vi "Main_Marvin Remake.vi"() -> ()   [LabVIEW 2017]
uses:
  PCAN_Driver/ControlCAN.llb/DevType.ctl
  PCAN_Driver/ControlCAN.llb/CAN Channel.ctl
  PCAN_Driver/ControlCAN.llb/VCI_INIT_CONFIG.ctl
  PCAN_Driver/ControlCAN.llb/InitFlag.ctl
  PCAN_Driver/ControlCAN.llb/Fliter.ctl
  PCAN_Driver/ControlCAN.llb/Mode.ctl
  <vilib>/Utility/miscctls.llb/LVRowAndColumnTypeDef.ctl
  <vilib>/Utility/config.llb/Read Key (String).vi
  <vilib>/Utility/config.llb/Write Key (String).vi
  <vilib>/Utility/cursorutil.llb/Set Cursor (Icon Pict).vi
  PCAN_Driver/ControlCAN.lvlib
  <vilib>/Utility/config.llb/NI_LVConfig.lvlib
panel:
  out "ClosePanel":bool=TRUE
  out "UUT SN Report":string
  out "Automation":bool
  out "Test Failed":bool
  out "AuxiOFFResult":bool
  out "AuxiONResult":bool
  out "SensCalResult":bool
  out "VisualInspectionResult":bool
  out "BurnResult":bool
  out "BurnSpeed":bool
  out "BurnTemp":bool
  out "BurnDC":bool
  out "TempControlResult":bool
  out "MotorTempResult":bool
  out "StopTimeResult":bool
  out "SpeedResult":bool=TRUE
  out "VenableDirectionResult":bool
  out "VenableResult":bool
  out "ComTestResult":bool=TRUE
  out "UUT SoftwareVer":string
  out "Next SN":i32
  in  "SetSN":bool
  out "Current SN":i32
  out "Cal":dbl
  out "AO[1]Meas":dbl
  out "FullSpeed2 Speed":dbl
  out "FullSpeed2 Current":dbl
  out "FullSpeed1 Current":dbl
  out "FullSpeed1 Speed":dbl
  out "MaxBurnInTempVal":dbl
  in  "Stop Burn-in":bool
  out "VISA Tester":refnum<visa-resource-name>
  out "UUT":u8
  out "CAN Status":bool
  in  "Channel 2":T1 caption="Channel" items=["Channel 1", "Channel 2"]
  out "Config_CANAT":T7 {"DevType" items=["USB-CAN"=3, "USB-CAN2"=4]; "CanIndex" items=["通道1", "通道2"]; "VCI_INIT_CONFIG"."Fliter" items=["接收所有类型"=3, "只接收标准帧"=4, "只接收扩展帧"=7]; "VCI_INIT_CONFIG"."Mode" items=["正常工作", "自测模式（环回）", "仅侦听模式"]; "VCI_INIT_CONFIG"."InitFlag" items=["使用Flash参数", "使用界面设置参数"]}
  out "Array":u64[][](array[numeric]) format="%016x"
  out "Motor Phase Current RMS":dbl
  out "Ambient Temperature":dbl
  out "Speed error":bool
  out "Commutation err":bool
  out "Under voltage/Over voltage":bool
  out "Derated drive temp":bool
  out "Motor Over temperature":bool
  out "Motor Sensor temp Fauilre":bool
  out "Drive Over temperature":bool
  out "Drive Sensor temp Failure":bool
  out "Ambient Over temp":bool
  out "Ambient Sensor temp":bool
  out "DC Voltage":dbl
  out "DC Current":dbl
  out "Power transistor Heat sink Temp.":dbl
  out "Motor Stator Temp.":dbl
  out "Motor Speed RPM":dbl
  out "ECS State":u16
  out "UUT":string="EBAY"
  in  "Logger Path":path
  in  "Report":bool
  in  "Start":bool
  in  "ATR":string[][](table)=[["Test Communication", "-", "-", "-", "-", ""], ["Set S/N", "-", "-", "-", "-", ""], ["Set Board Number", "-", "-", "-", "-", ""], [" ", "", "", "", "", ""], ["Test Communication", "-", "-", "-", "-", ""], ["Get S/N", "-", "-", "-", "", ""], ["Get Board Number", "-", "-", "-", "", ""], ["Get FW", "-", "-", "-", "", ""], ["Enable Motor", "", "", "", "", ""], ["Small position command", "", "", "", "", ""], ["Measure delta", "", "", "", "", ""], ["Velocity command", "", "", "", "", ""]]
  in  "Settings":bool
  in  "Refresh Button":bool
  out "Status":bool
  in  "VISA Marvin":refnum<visa-resource-name>="COM6"
  in  "Serial Com":bool
  in  "Help Button":bool
  out "Pannel User Message":string
  in  "Stop Button":bool
  # "Marvin"
  # "REDLER TECHNOLOGIES LTD"
  # "ver 1.2l"
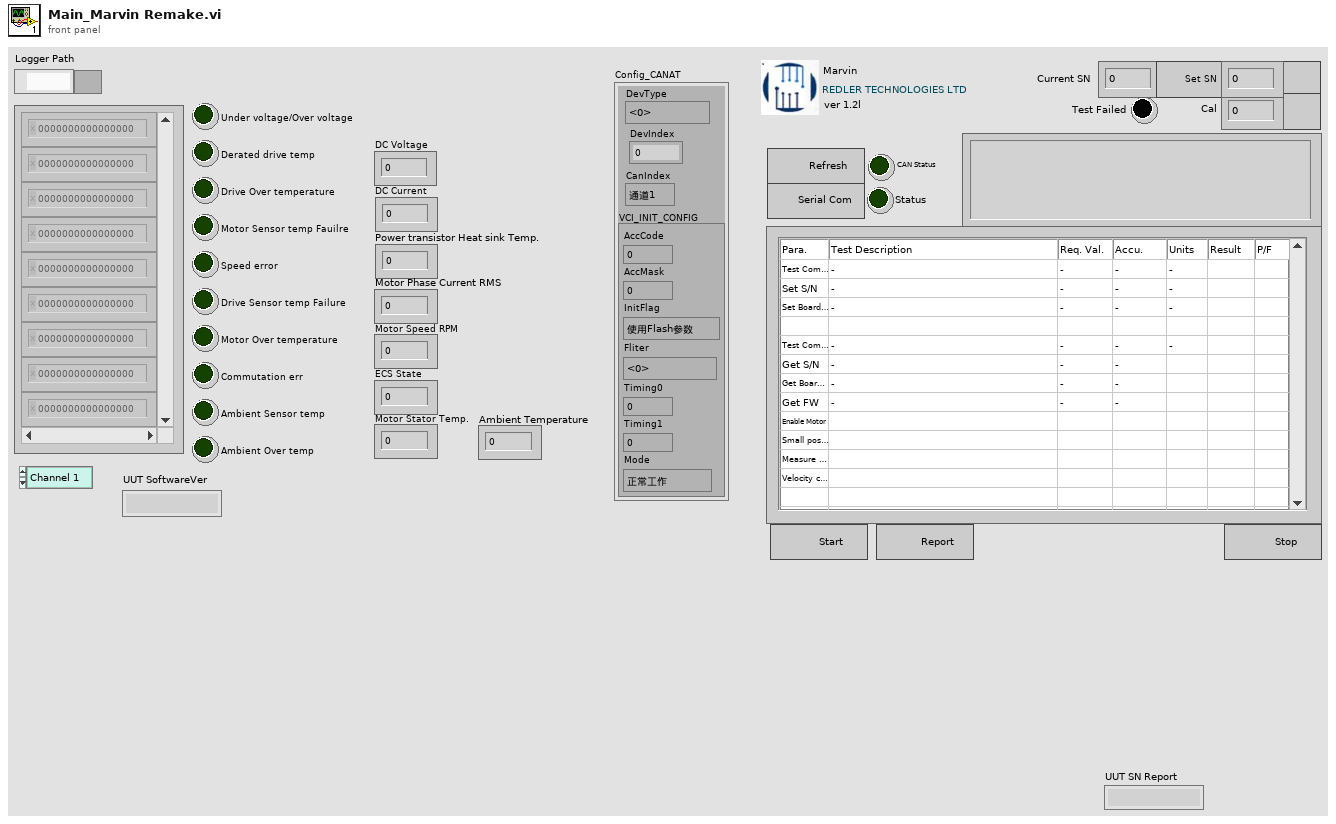
[diagram p1: front panel]
types:
  T1 = typedef "ControlCAN.lvlib/CAN Channel.ctl" = u32
  T2 = typedef "ControlCAN.lvlib/DevType.ctl" = u32
  T3 = typedef "ControlCAN.lvlib/VCI_INIT_CONFIG.ctl" = cluster{"AccCode":u32, "AccMask":u32, "InitFlag":T4, "Fliter":T5, "Timing0":u8, "Timing1":u8, "Mode":T6}
  T4 = typedef "ControlCAN.lvlib/InitFlag.ctl" = u32
  T5 = typedef "ControlCAN.lvlib/Fliter.ctl" = u8
  T6 = typedef "ControlCAN.lvlib/Mode.ctl" = u8
  T7 = cluster{"DevType":T2, "DevIndex":u32, "CanIndex":T1, "VCI_INIT_CONFIG":T3}
  T8 = cluster{"VISA":refnum<visa-resource-name>, "Array Test":enum16{"Auxiliary", "Temp Sens Cal", "Com Test", "Enable Test", "Speed Command", "Stop Time", "Temp Control", "Burn in", "Visual Inspec", "Empty"}[]}
  T9 = cluster{"ID":u32, "MSGTYPE":u8, "LEN":u8, "aDATA":u8[]}[]
  T10 = enum16{"Erase ATR Table", "Stop", "MainProgram", "Initialize"}
  T11 = enum16{"K15", "K16", "K17", "Venable", "Firmeware", "Fan", "Power", "120C", "110C", "100C", "90C", "80C", "70C", "60C", "50C", "40C", "30C", "25C", "20C", "10C", "0C"}
  T12 = enum16{"Stop", "Result", "FullSpeed2", "MD[1]=1", "FullSpeed1", "MD[1]=0"}
  T13 = enum8{"Term1", "Term2", "Current", "Fan", "TempCPU"}
  T14 = enum16{"Stop", "AO[1]=Meas.", "TA[5]", "AO[1]=0", "Start"}
  T15 = enum16{"Stop", "BurnIn", "Ambient Temp", "MotorSpeed", "DC Current Measure", "Start"}
  T16 = enum16{"Auxiliary", "Temp Sens Cal", "Com Test", "Enable Test", "Speed Command", "Stop Time", "Temp Control", "Burn in", "Visual Inspec", "Empty"}[]
  T17 = enum16{"K15", "K16", "K17", "Venable", "Firmeware", "Fan", "Power", "120C", "110C", "100C", "90C", "80C", "70C", "60C", "50C", "40C", "30C", "25C", "20C", "10C", "0C"}[]
  T18 = enum32{"6000", "11500", "15100", "11500-2", "6000-2"}[]
  T19 = enum8{"Enabled", "Disabled", "Disabled and Grayed Out"}
  T20 = typedef "LVRowAndColumnTypeDef.ctl" = cluster{"Row":i32, "Column":i32}
  T21 = enum32{"Invalid", "Standard", "Closed", "Hidden", "Minimized", "Maximized"}
  T22 = cluster{"ID":u32, "MSGTYPE":u8, "LEN":u8, "aDATA":u8[]}
  T23 = enum16{"Auxiliary", "Temp Sens Cal", "Com Test", "Enable Test", "Speed Command", "Stop Time", "Temp Control", "Burn in", "Visual Inspec", "Empty"}
  T24 = enum16{"open", "replace", "create", "open or create", "replace or create", "replace or create with confirmation"}
  T25 = typedef "NI_LVConfig.lvlib/Config Data RefNum.ctl" = refnum<k1>
  T26 = typedef "ControlCAN.lvlib/VCI_CAN_OBJ.ctl" = cluster{"ID":u32, "TimeStamp":u32, "TimeFlag":u8, "SendType":u8, "RemoteFlag":u8, "ExternFlag":u8, "DataLen":u8, "Data":u8[], "Reserved":u8[]}
  T27 = cluster{"Type":enum16{"接收", "发送"}, "Channel":T1, "Time":timestamp, "VCI_CAN_OBJ":T26}[]
  T28 = cluster{"Type":enum16{"接收", "发送"}, "Channel":T1, "Time":timestamp, "VCI_CAN_OBJ":T26}
  T29 = typedef "LVPoint32TypeDef.ctl" = cluster{"Horizontal":i32, "Vertical":i32}
  T30 = enum8{"Term1", "Term2", "Current", "Fan", "TempCPU"}[]
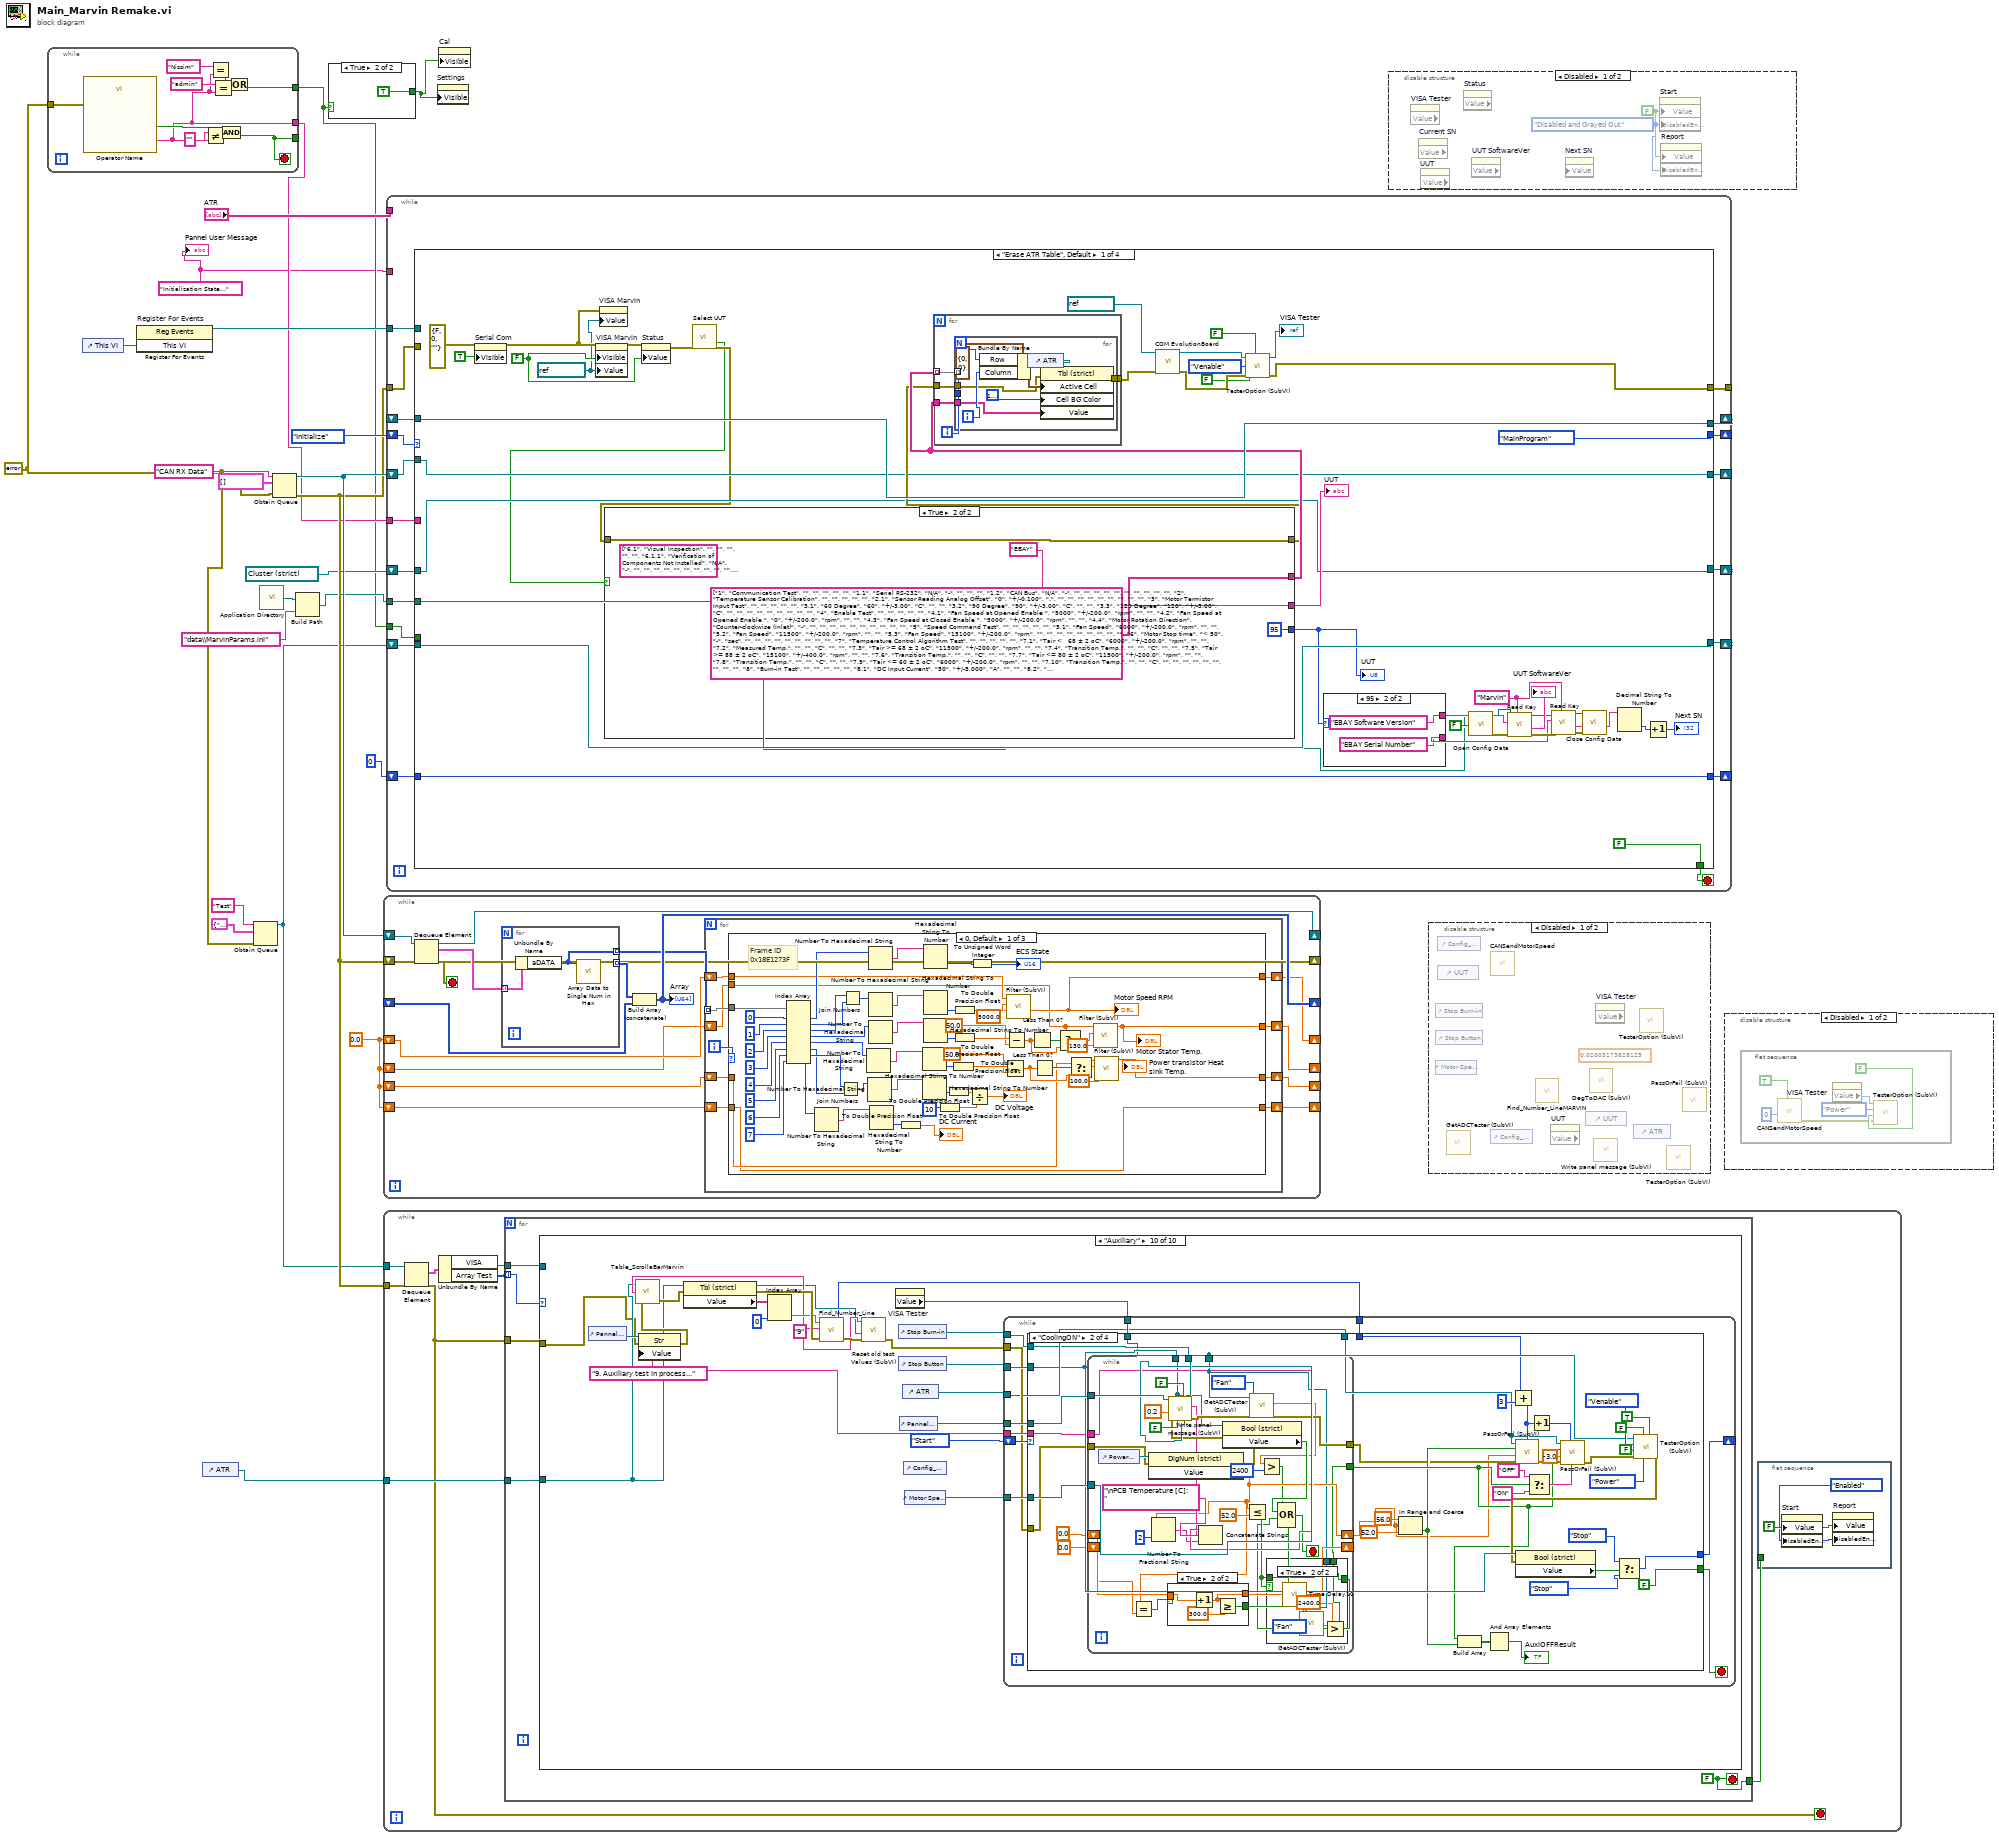
[diagram p0: block diagram]
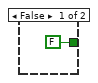
[diagram p2: hidden frame]
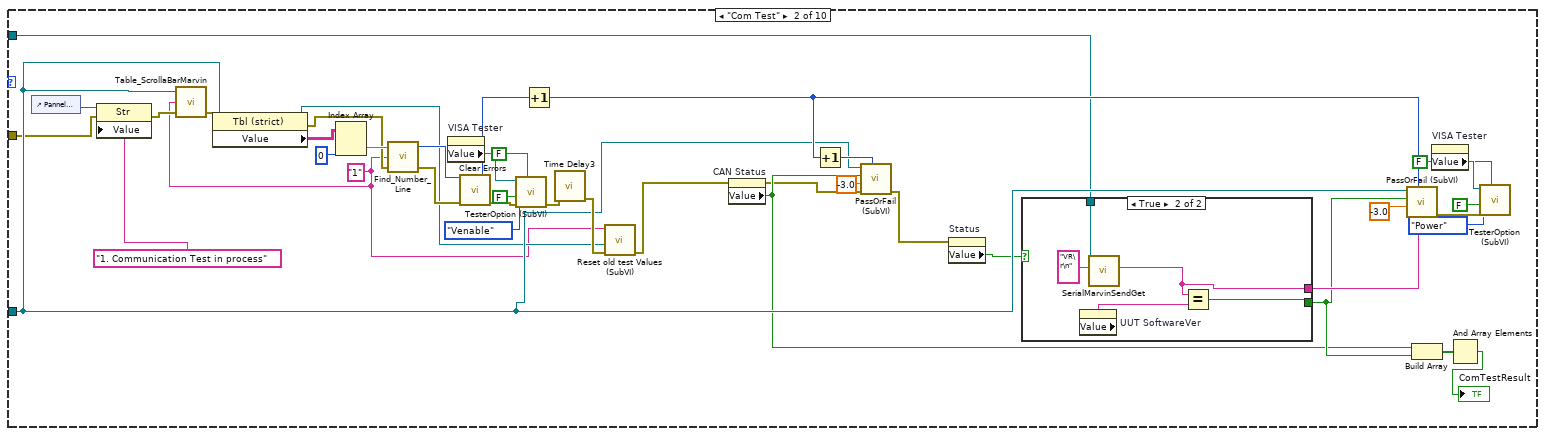
[diagram p7: hidden frame]
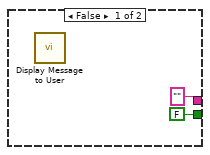
[diagram p8: hidden frame]
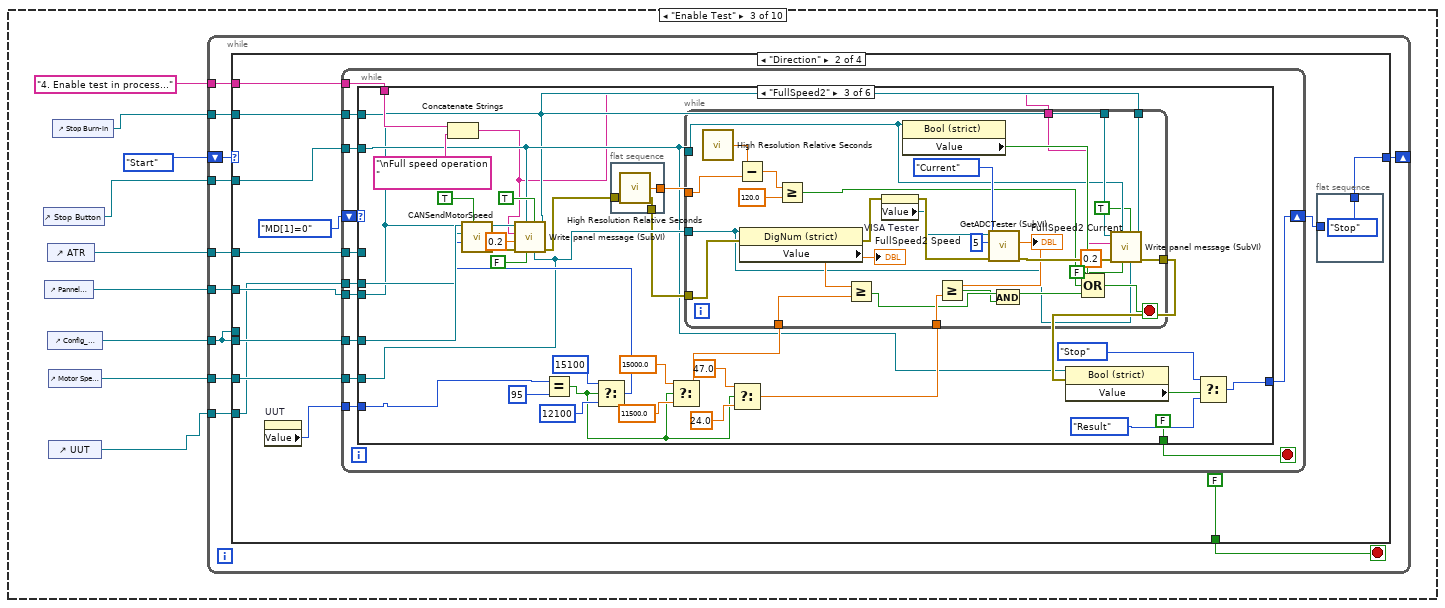
[diagram p9: hidden frame]
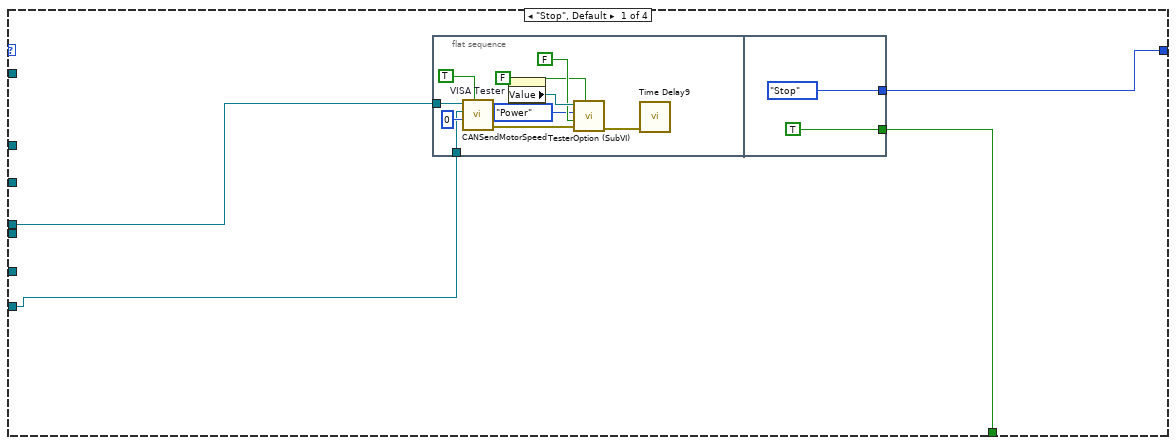
[diagram p10: hidden frame]
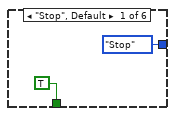
[diagram p11: hidden frame]
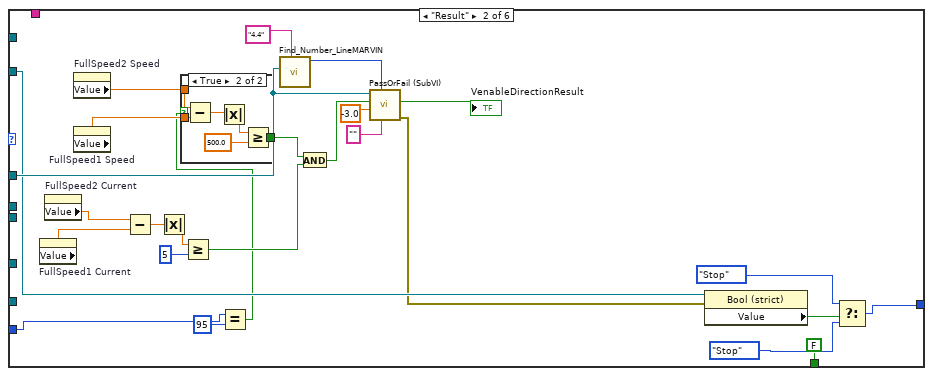
[diagram p12: hidden frame]
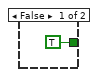
[diagram p13: hidden frame]
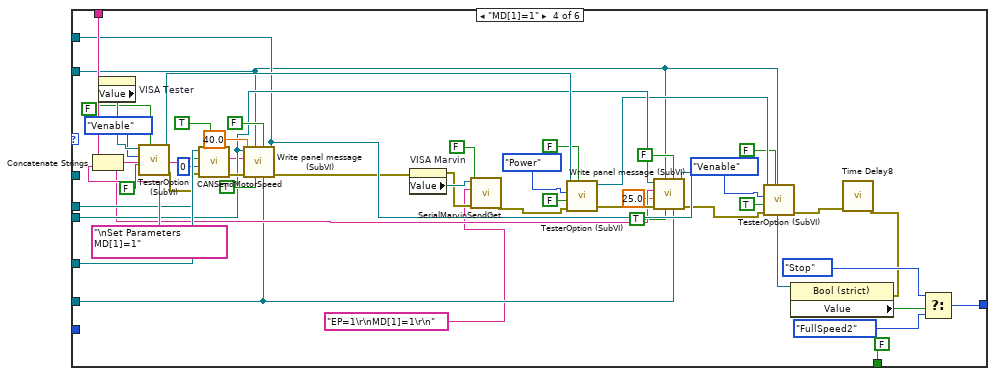
[diagram p14: hidden frame]
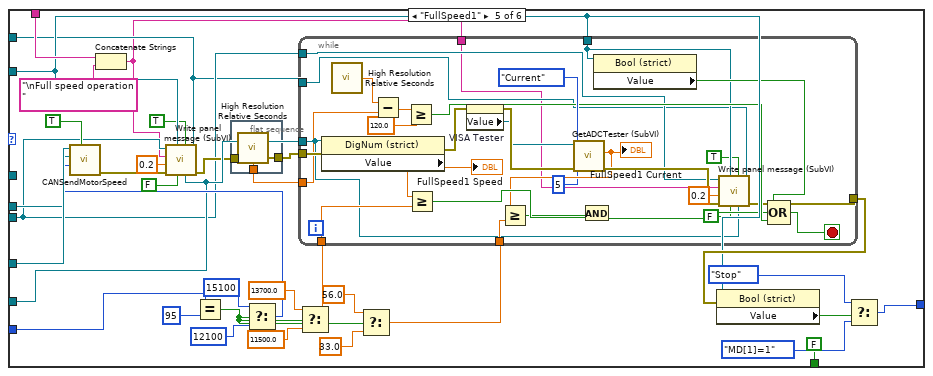
[diagram p15: hidden frame]
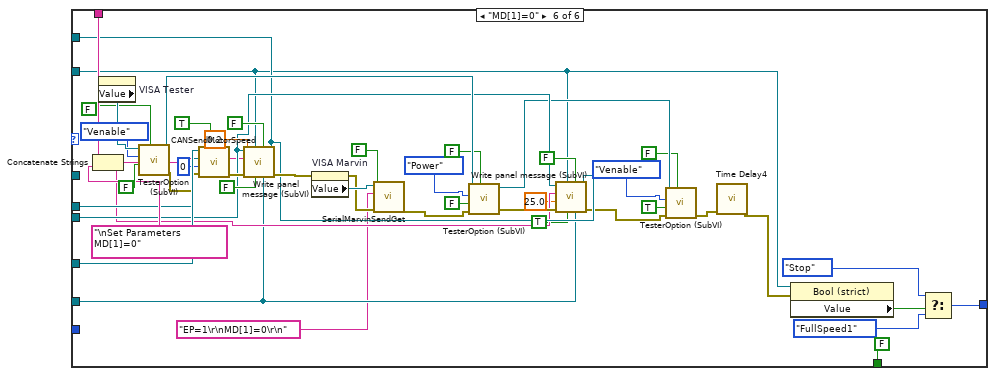
[diagram p16: hidden frame]
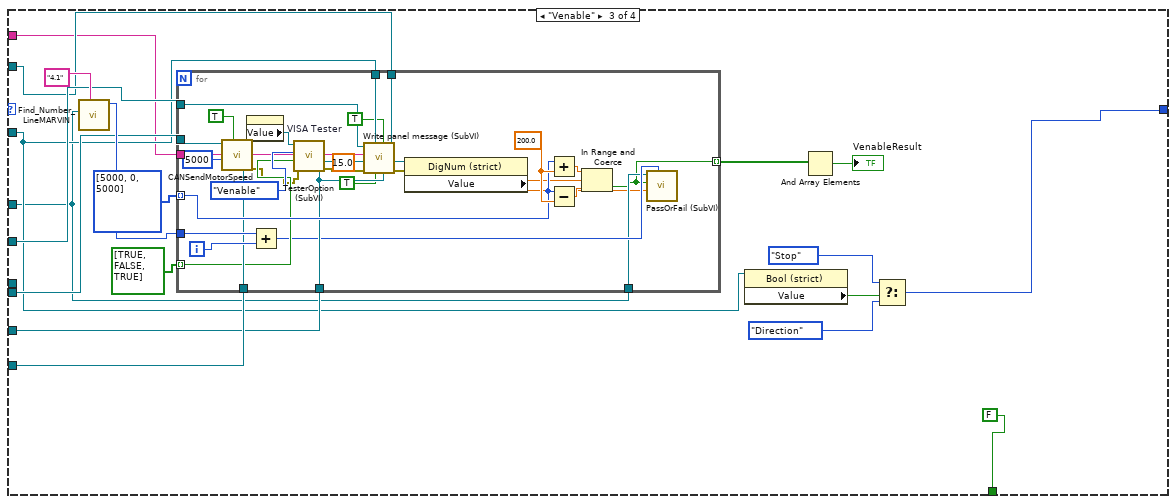
[diagram p17: hidden frame]
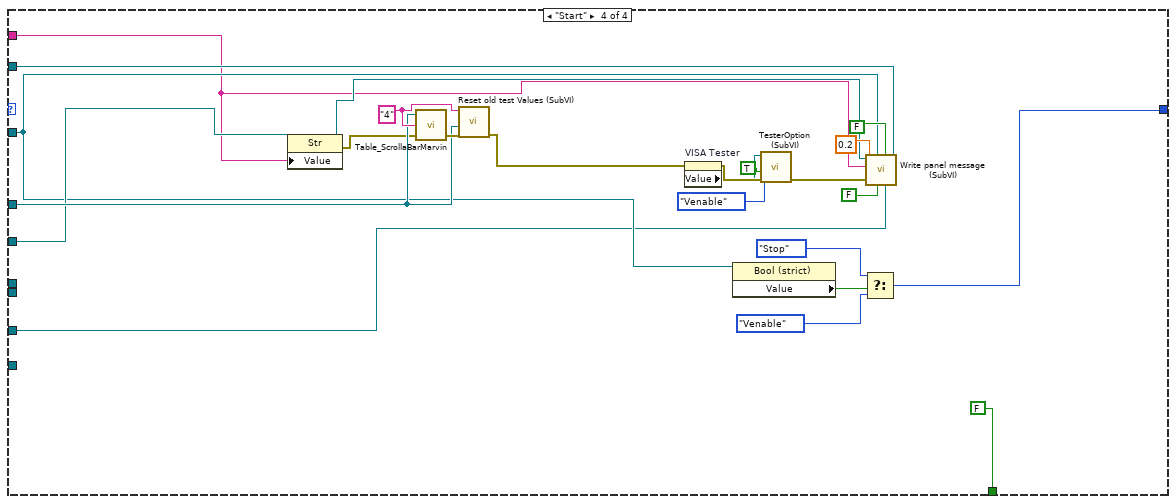
[diagram p18: hidden frame]
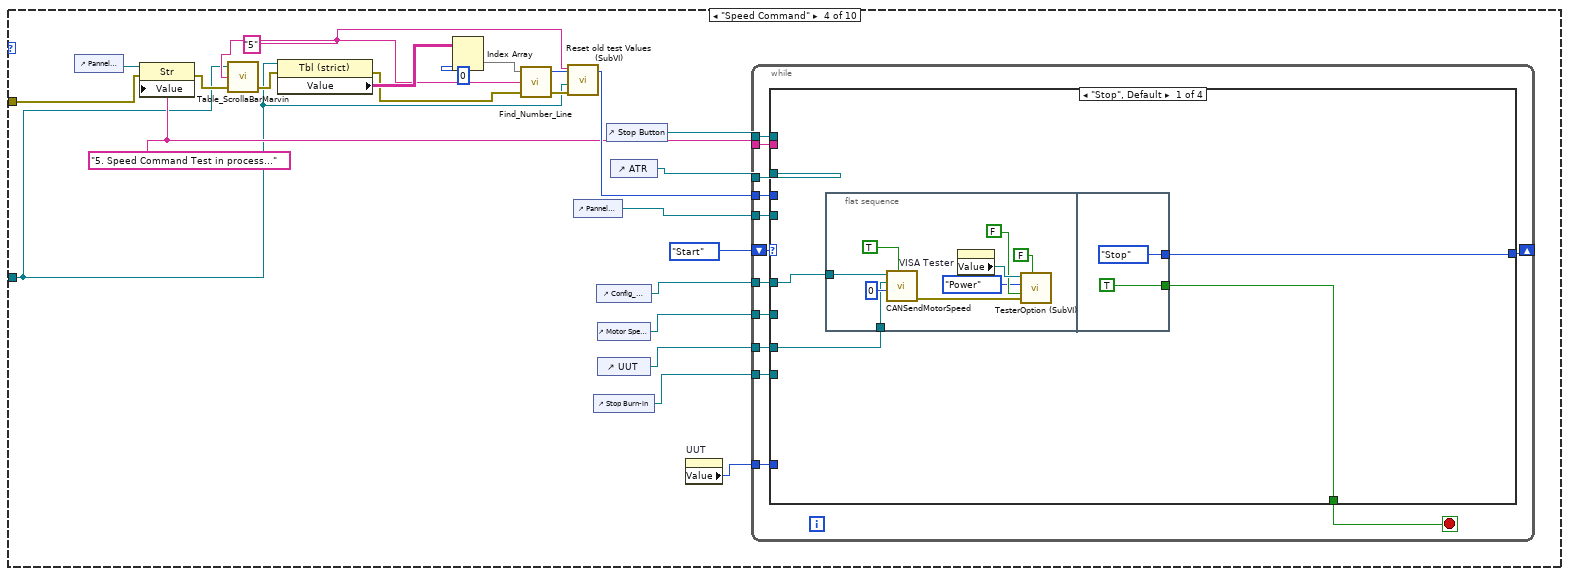
[diagram p19: hidden frame]
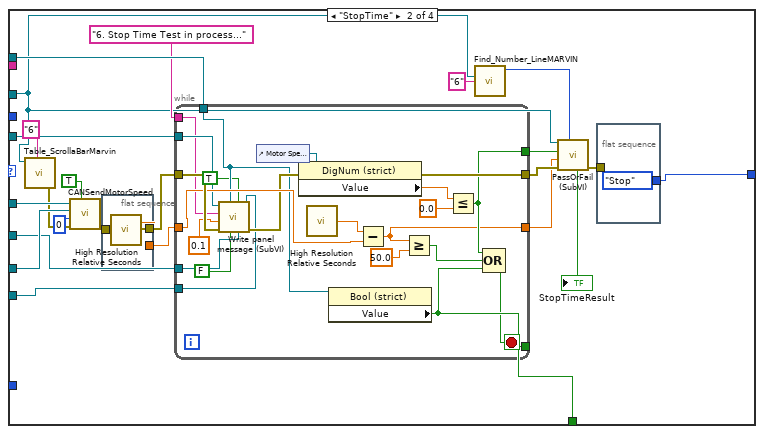
[diagram p20: hidden frame]
diagram:
  w2 = "Initialization State..."
  w13 = 0.0
  w12 = errorcluster {"status"=FALSE, "code"=0, "source"=""} ("error in (no error)")
  n1 = while {
    tunnel: [w31] -> _
    tunnel: [w27] -> w7
    tunnel: [w28] -> w3
    tunnel: w12 -> [w24]
    stop <- w31 stop-if-true
    n2 = call "Operator Name"("error in (no error)"=w24) -> ("Operator Name"=w27:string, "OK"=w32:bool)  [unwired: 16 in, 1 out]
    n3 = Not Equal?(x=w27, y="") -> (x != y?=w33:bool)
    n4 = Equal?(x="Nissim", y=w27) -> (x = y?=w25:bool)
    n5 = Equal?(x="admin", y=w27) -> (x = y?=w29:bool)
    n6 = And(x=w32, y=w33) -> (x .and. y?=w31:bool)
    n7 = Or(x=w25, y=w29) -> (x .or. y?=w28:bool)
  }
  n8 = control-ref of="This VI"() -> (w9:refnum<vi>)
  n9 = register-events "Register For Events"(w9) -> (reference out=w8:refnum<event-registration>)  [unwired: 2 in, 1 out]
  n10 = control-ref of="ATR"() -> (w1:refnum<vi>)
  n11 = Obtain Queue(name (unnamed)="Test", element data type=T8 {"VISA"="COM1", "Array Test"=[]}, error in (no error)=w12) -> (queue out=w17:refnum<queue>)  [unwired: 2 in, 2 out]
  n12 = call <vilib>:"Application Directory.vi"() -> ("Application Directory"=w11:path)
  n13 = Obtain Queue(name (unnamed)="CAN RX Data", element data type=T9 [], error in (no error)=w12) -> (queue out=w20:refnum<queue>, error out=w18:errorcluster)  [unwired: 2 in, 1 out]
  n14 = Build Path(base path=w11, name or relative path="data\\MarvinParams.ini") -> (appended path=w5:path)
  n15 = case shown="True" w3 {
    tunnel: [FALSE TRUE] -> w4
    frame False {
    }
    frame True {
    }
  }
  n16 = while {
    shift-right: [w51] -> _
    shift-left: w20 -> [w53]
    shift-right: [w49] -> _
    shift-left: _ -> [w50]
    shift-right: [w45] -> _
    shift-left: w18 -> [w45]
    shift-right: [w43] -> _
    shift-left: w13 -> [w44]
    shift-right: [w42] -> _
    shift-left: w13 -> [w41]
    shift-right: [w40] -> _
    shift-left: w13 -> [w39]
    shift-right: [w38] -> _
    shift-left: w13 -> [w37]
    stop <- w52 stop-if-true
    n17 = Dequeue Element(queue=w53, error in (no error)=w45) -> (queue out=w51:refnum<queue>, element=w46:T9, error out=w52:errorcluster)  [unwired: 1 in, 1 out]
    n18 = for {
      tunnel: [w182] -> w48 mode=indexing
      tunnel: w46 -> [w181] mode=indexing
      tunnel: [w180] -> w47 mode=indexing
      n19 = Unbundle By Name(w181) -> ("aDATA"=w180:u8[])
      n20 = call "Array Data to Single Num in Hex.vi"("aDATA"=w180) -> ("Numeric"=w182:u64)  [unwired: 10 in]
    }
    n21 = Build Array (concatenate)(w48, w50) -> (w49:u64[][])
    "Array" <- w49
    n22 = for {
      tunnel: w47 -> [w63] mode=indexing
      shift-right: [w60] -> w43
      shift-left: w44 -> [w61]
      shift-right: [w59] -> w42
      shift-left: w41 -> [w58]
      shift-right: [w57] -> w40
      shift-left: w39 -> [w56]
      shift-right: [w55] -> w38
      shift-left: w37 -> [w54]
      i -> [w62]
      n23 = case shown="0, Default" w62 {
        tunnel: w63 -> [w103 w136 w175]
        tunnel: w61 -> [w77 w125 w164]
        tunnel: [w75 w125 w164] -> w60
        tunnel: [w72 w124 w163] -> w59
        tunnel: w58 -> [w71 w124 w163]
        tunnel: [w66 w123 w162] -> w57
        tunnel: w56 -> [w65 w123 w162]
        tunnel: [w64 w122 w157] -> w55
        tunnel: w54 -> [w64 w122 w156]
        frame 0, Default {
          # "Frame ID\n0x18E1273F"
          n24 = Index Array(array=w103, index #1=0 ("index"), index #2=1 ("index"), index #3=2 ("index"), index #4=3 ("index"), index #5=4 ("index"), index #6=5 ("index"), index #7=6 ("index"), index #8=7 ("index")) -> (element #1=w87:u8, element #2=w89:u8, element #3=w90:u8, element #4=w94:u8, element #5=w97:u8, element #6=w101:u8, element #7=w102:u8, element #8=w100:u8)
          n25 = Number To Hexadecimal String(2:w100) -> (0:w114:string)  [unwired: 1 in]
          n26 = Join Numbers(hi=w102, lo=w101) -> ((hi.lo)=w121:u16)
          n27 = Join Numbers(hi=w90, lo=w89) -> ((hi.lo)=w91:u16)
          n28 = Number To Hexadecimal String(2:w97) -> (0:w98:string)  [unwired: 1 in]
          n29 = Number To Hexadecimal String(2:w121) -> (0:w120:string)  [unwired: 1 in]
          n30 = Number To Hexadecimal String(2:w87) -> (0:w88:string)  [unwired: 1 in]
          n31 = Number To Hexadecimal String(2:w91) -> (0:w92:string)  [unwired: 1 in]
          n32 = Number To Hexadecimal String(2:w94) -> (0:w95:string)  [unwired: 1 in]
          n33 = Hexadecimal String To Number(string=w114) -> (number=w113:u32)  [unwired: 2 in, 1 out]
          n34 = To Double Precision Float(number=w113) -> (double precision float=→"DC Current":dbl)
          n35 = Hexadecimal String To Number(string=w98) -> (number=w99:u32)  [unwired: 2 in, 1 out]
          n36 = Hexadecimal String To Number(string=w120) -> (number=w119:u32)  [unwired: 2 in, 1 out]
          n37 = Hexadecimal String To Number(string=w88) -> (number=w85:u32)  [unwired: 2 in, 1 out]
          n38 = Hexadecimal String To Number(string=w92) -> (number=w93:u32)  [unwired: 2 in, 1 out]
          n39 = Hexadecimal String To Number(string=w95) -> (number=w96:u32)  [unwired: 2 in, 1 out]
          n40 = To Double Precision Float(number=u32 10 ("y")) -> (double precision float=w117:dbl)
          n41 = To Double Precision Float(number=w119) -> (double precision float=w116:dbl)
          n42 = To Double Precision Float(number=w99) -> (double precision float=w82:dbl)
          n43 = To Double Precision Float(number=w93) -> (double precision float=w78:dbl)
          n44 = To Double Precision Float(number=w96) -> (double precision float=w84:dbl)
          n45 = Divide(x=w116, y=w117) -> (x/y=→"DC Voltage":dbl)
          n46 = To Unsigned Word Integer(number=w85) -> (unsigned 16bit integer=→"ECS State":u16)
          n47 = Subtract(x=w82, y=50.0 ("x")) -> (x-y=w70:dbl)
          n48 = Subtract(x=w84, y=50.0 ("x")) -> (x-y=w73:dbl)
          n49 = call "Filter (SubVI).vi"("Delta"=5000.0, "NewVal"=w78, "OldVal"=w77) -> ("Val"=w75:dbl)  [unwired: 8 in]
          "Motor Speed RPM" <- w75
          n50 = Less Than 0?(x=w73) -> (x < 0?=w80:bool)
          n51 = Less Than 0?(x=w70) -> (x < 0?=w79:bool)
          n52 = Select(t=w71, s=w80, f=w73) -> (s? t:f=w74:dbl)
          n53 = Select(t=w65, s=w79, f=w70) -> (s? t:f=w69:dbl)
          n54 = call "Filter (SubVI).vi"("Delta"=130.0, "NewVal"=w74, "OldVal"=w71) -> ("Val"=w72:dbl)  [unwired: 8 in]
          "Motor Stator Temp." <- w72
          n55 = call "Filter (SubVI).vi"("Delta"=100.0, "NewVal"=w69, "OldVal"=w65) -> ("Val"=w66:dbl)  [unwired: 8 in]
          "Power transistor Heat sink Temp." <- w66
        }
        frame 1 {
          # "Framde ID\n0x18E3273F"
          n56 = control-ref of="UUT"() -> (w126:refnum<vi>)
          n57 = property on="Property Node" class="DigNum (strict)"(reference=w126) -> ("Value"=w127:u8)  [unwired: 1 in, 2 out]
          n58 = Index Array(array=w136, index #1=0 ("index"), index #2=1 ("index")) -> (element #1=w134:u8, element #2=w129:u8)
          n59 = Number To Boolean Array(number=w134) -> (Boolean array=w133:bool[])
          n60 = Number To Boolean Array(number=w129) -> (Boolean array=w131:bool[])
          n61 = Boolean To (0,1)(Boolean=w131) -> (0, 1=w128:i16[])
          n62 = Boolean To (0,1)(Boolean=w133) -> (0, 1=w132:i16[])
          n63 = case shown="95" w127 {
            tunnel: w128 -> [_ w137]
            frame 0, Default {
            }
            frame 95 {
              n64 = for {
                tunnel: w137 -> [w142] mode=indexing
                i -> [w138]
                stop <- w140 stop-if-true
                n65 = Not Equal To 0?(x=w142) -> (x != 0?=w141:bool)
                n66 = case shown="0, Default" w138 {
                  tunnel: w141 -> [w143 w144]
                  frame 0, Default {
                    "Ambient Sensor temp" <- w143
                  }
                  frame 1 {
                    "Ambient Over temp" <- w144
                  }
                }
                n67 = Equal?(x=w138, y=1.0) -> (x = y?=w140:bool)
              }
            }
          }
          n68 = for {
            tunnel: w132 -> [w146] mode=indexing
            i -> [w147]
            n69 = Not Equal To 0?(x=w146) -> (x != 0?=w145:bool)
            n70 = case shown="1" w147 {
              tunnel: w145 -> [w148 w149 w150 w151 w152 w153 w154 w155]
              frame 0, Default {
                "Drive Sensor temp Failure" <- w148
              }
              frame 1 {
                "Drive Over temperature" <- w149
              }
              frame 2 {
                "Motor Sensor temp Fauilre" <- w150
              }
              frame 3 {
                "Motor Over temperature" <- w151
              }
              frame 4 {
                "Derated drive temp" <- w152
              }
              frame 5 {
                "Under voltage/Over voltage" <- w153
              }
              frame 6 {
                "Commutation err" <- w154
              }
              frame 7 {
                "Speed error" <- w155
              }
            }
          }
        }
        frame 2 {
          # "Frame ID\n0x18E2273F"
          n71 = Index Array(array=w175, index #1=0 ("index"), index #2=1 ("index")) -> (element #1=w172:u8, element #2=w169:u8)
          n72 = disable-structure shown="Enabled" {
            disable-tunnel: [w178 w179] -> w173
            disable-tunnel: w172 -> [w177 w179]
            frame Disabled {
              n73 = Number To Hexadecimal String(2:w177) -> (0:w176:string)  [unwired: 1 in]
              n74 = Hexadecimal String To Number(string=w176) -> (number=w178:u32)  [unwired: 2 in, 1 out]
            }
            frame Enabled {
            }
          }
          n75 = Number To Hexadecimal String(2:w169) -> (0:w167:string)  [unwired: 1 in]
          n76 = Hexadecimal String To Number(string=w167) -> (number=w168:u32)  [unwired: 2 in, 1 out]
          n77 = To Double Precision Float(number=w168) -> (double precision float=w166:dbl)
          n78 = To Double Precision Float(number=w173) -> (double precision float=→"Motor Phase Current RMS":dbl)
          n79 = Subtract(x=w166, y=50.0) -> (x-y=w160:dbl)
          n80 = Less Than 0?(x=w160) -> (x < 0?=w161:bool)
          n81 = Select(t=w156, s=w161, f=w160) -> (s? t:f=w159:dbl)
          n82 = call "Filter (SubVI).vi"("Delta"=65.0, "NewVal"=w159, "OldVal"=w156) -> ("Val"=w157:dbl)  [unwired: 8 in]
          "Ambient Temperature" <- w157
        }
      }
    }
  }
  n83 = while {
    tunnel: w1 -> [w190]
    tunnel: w18 -> [w188]
    tunnel: w17 -> [w189]
    stop <- w184 stop-if-true
    n84 = Dequeue Element(queue=w189, error in (no error)=w188) -> (element=w187:T8, error out=w184:errorcluster)  [unwired: 1 in, 2 out]
    n85 = Unbundle By Name(w187) -> ("VISA"=w186:refnum<visa-resource-name>, "Array Test"=w185:T16)
    n86 = for {
      tunnel: w185 -> [w194] mode=indexing
      tunnel: w186 -> [w197]
      tunnel: w190 -> [w196]
      tunnel: w184 -> [w195]
      tunnel: [w193] -> w183
      stop <- w193 stop-if-true
      w193 = FALSE
      n87 = case shown="\"Auxiliary\"" w194 {
        tunnel: w197 -> [_ w221 _ _ w803 _ _ _ w1358 _]
        tunnel: w196 -> [_ w228 _ w638 w799 w962 _ w1344 w1365 w1577]
        tunnel: w195 -> [_ w225 _ w653 w809 w960 _ w1343 w1363 w1576]
        frame "Empty", Default {
        }
        frame "Com Test" {
          w204 = "1" ("Test Paragraph")
          n88 = control-ref of="Pannel User Message"() -> (w226:refnum<vi>)
          n89 = property class="Str"(reference=w226, error in=w225, "Value"="1. Communication Test in process") -> (error out=w224:errorcluster)  [unwired: 1 out]
          n90 = call "Table_ScrollaBarMarvin.vi"("error in"=w224, "Line to focus"=w204, "reference in"=w228) -> ("error out"=w227:errorcluster)  [unwired: 2 out]
          n91 = property class="Tbl (strict)"(reference=w228, error in=w227) -> (reference out=w205:refnum<vi>, error out=w235:errorcluster, "Value"=w236:string[][])
          n92 = Index Array(array=w236, index (col)=0 ("disabled index (col)")) -> (element=w237:string[])  [unwired: 1 in]
          n93 = call "Find_Number_Line.vi"("error in"=w235, "Test Paragraph"=w204, "Row Headers[]"=w237) -> ("error out"=w233:errorcluster, "Line number"=w232:i32)  [unwired: 1 out]
          n94 = property on="VISA Tester" class="VISAName"() -> ("Value"=w215:refnum<visa-resource-name>)  [unwired: 2 in, 2 out]
          n95 = call <vilib>:"Clear Errors.vi"("error in (no error)"=w233) -> ("error out"=w217:errorcluster)  [unwired: 5 in, 1 out]
          n96 = call "TesterOption (SubVI).vi"("2 Options"=FALSE, "error in (no error)"=w217, "On/Off"=FALSE, "Tester Option"=T11."Venable", "VISA Refnum in"=w215) -> ("error out"=w216:errorcluster)  [unwired: 5 in, 1 out]
          n97 = Increment(x=w232) -> (x+1=w231:i32)
          n98 = call "Time Delay3"("error in (no error)"=w216) -> ("error out"=w229:errorcluster)  [unwired: 10 in]
          n99 = call "Reset old test Values (SubVI).vi"("error in"=w229, "Atr in"=w205, "Test Paragraph"=w204) -> ("error out"=w199:errorcluster)  [unwired: 8 in]
          n100 = property on="CAN Status" class="Bool (strict)"(error in=w199) -> (error out=w198:errorcluster, "Value"=w200:bool)  [unwired: 1 in, 1 out]
          n101 = Increment(x=w231) -> (x+1=w230:i32)
          n102 = call "PassOrFail (SubVI).vi"("index (row)"=w230, "error in (no error)"=w198, "Data in"=-3.0, "Pass?Fail"=w200, "Table in"=w228) -> ("error out"=w220:errorcluster)  [unwired: 6 in]
          n103 = property on="Status" class="Bool (strict)"(error in=w220) -> ("Value"=w222:bool)  [unwired: 1 in, 2 out]
          n104 = case shown="True" w222 {
            tunnel: w221 -> [_ w244]
            tunnel: [FALSE w241] -> w202
            tunnel: ["" ("read buffer") w240] -> w219
            frame False {
              n105 = call "Display Message to User"() -> ()  [unwired: 10 in, 2 out]
            }
            frame True {
              n106 = property on="UUT SoftwareVer" class="Str"() -> ("Value"=w242:string)  [unwired: 2 in, 2 out]
              n107 = call "SerialMarvinSendGet.vi"("write buffer"="VR\r\n", "VISA resource name"=w244) -> ("read buffer"=w240:string)  [unwired: 8 in, 1 out]
              n108 = Equal?(x=w240, y=w242) -> (x = y?=w241:bool)
            }
          }
          n109 = call "PassOrFail (SubVI).vi"("String Res"=w219, "index (row)"=w231, "Data in"=-3.0, "Pass?Fail"=w202, "Table in"=w228) -> ("error out"=w211:errorcluster)  [unwired: 6 in]
          n110 = Build Array(w200, w202) -> (w203:bool[])
          n111 = property on="VISA Tester" class="VISAName"() -> ("Value"=w210:refnum<visa-resource-name>)  [unwired: 2 in, 2 out]
          n112 = And Array Elements(Boolean array=w203) -> (logical AND=→"ComTestResult":bool)
          n113 = call "TesterOption (SubVI).vi"("2 Options"=FALSE, "error in (no error)"=w211, "On/Off"=FALSE, "Tester Option"=T11."Power", "VISA Refnum in"=w210) -> ()  [unwired: 5 in, 2 out]
        }
        frame "Enable Test" {
          n114 = control-ref of="Stop Button"() -> (w247:refnum<vi>)
          n115 = control-ref of="Pannel User Message"() -> (w249:refnum<vi>)
          n116 = control-ref of="ATR"() -> (w248:refnum<vi>)
          n117 = control-ref of="Config_CANAT"() -> (w250:refnum<vi>)
          n118 = control-ref of="Motor Speed RPM"() -> (w251:refnum<vi>)
          n119 = control-ref of="UUT"() -> (w252:refnum<vi>)
          n120 = control-ref of="Stop Burn-in"() -> (w253:refnum<vi>)
          n121 = while {
            shift-right: [w258] -> _
            shift-left: enum16{"Stop", "Direction", "Venable", "Start"}."Start" -> [w264]
            tunnel: w247 -> [w263]
            tunnel: w248 -> [w262]
            tunnel: w249 -> [w261]
            tunnel: w250 -> [w254]
            tunnel: w251 -> [w260]
            tunnel: w252 -> [w255]
            tunnel: w253 -> [w257]
            tunnel: "4. Enable test in process..." ("Strin") -> [w256]
            stop <- w259 stop-if-true
            n122 = case shown="\"Direction\"" w264 {
              tunnel: w263 -> [_ w291 w572 w617]
              tunnel: w262 -> [_ w286 w570 w624]
              tunnel: w261 -> [_ w289 w574 w623]
              tunnel: w254 -> [_ w292 w577 _]
              tunnel: w260 -> [_ w288 w575 w615]
              tunnel: w255 -> [w265 w282 w576 _]
              tunnel: [w268 FALSE FALSE FALSE] -> w259
              tunnel: [w266 w285 w571 w621] -> w258
              tunnel: w257 -> [_ w290 w573 w616]
              tunnel: w256 -> [_ w287 w569 w614]
              tunnel: w254 -> [w267 _ _ _]
              frame "Stop", Default {
                n123 = flat-sequence {
                  tunnel: w265 -> [w274]
                  tunnel: w267 -> [w273]
                  tunnel: [TRUE] -> w268
                  tunnel: [enum16{"Stop", "Direction", "Venable", "Start"}."Stop"] -> w266
                  frame #0 {
                    n124 = call "CANSendMotorSpeed.vi"("Remote"=TRUE, "Motor Speed RPM"=u16 0, "UUT"=w274, "CAN Cluster in"=w273) -> ("error out"=w277:errorcluster)  [unwired: 7 in]
                    n125 = property on="VISA Tester" class="VISAName"() -> ("Value"=w278:refnum<visa-resource-name>)  [unwired: 2 in, 2 out]
                    n126 = call "TesterOption (SubVI).vi"("2 Options"=FALSE, "error in (no error)"=w277, "On/Off"=FALSE, "Tester Option"=T11."Power", "VISA Refnum in"=w278) -> ("error out"=w269:errorcluster)  [unwired: 5 in, 1 out]
                    n127 = call "Time Delay9"("error in (no error)"=w269) -> ()  [unwired: 10 in, 1 out]
                  }
                  frame #1 {
                  }
                }
              }
              frame "Direction" {
                n128 = property on="UUT" class="DigNum (strict)"() -> ("Value"=w281:u8)  [unwired: 2 in, 2 out]
                n129 = while {
                  shift-right: [w305] -> w284
                  shift-left: T12."MD[1]=0" -> [w306]
                  tunnel: w292 -> [w303]
                  tunnel: w282 -> [w302]
                  tunnel: w291 -> [w301]
                  tunnel: w290 -> [w300]
                  tunnel: w289 -> [w299]
                  tunnel: w288 -> [w298]
                  tunnel: w287 -> [w297]
                  tunnel: w286 -> [w296]
                  tunnel: w281 -> [w295]
                  stop <- w304 stop-if-true
                  n130 = case shown="\"FullSpeed2\"" w306 {
                    tunnel: [T12."Stop" w330 w372 w452 w485 w565] -> w305
                    tunnel: [TRUE FALSE FALSE FALSE FALSE FALSE] -> w304
                    tunnel: w303 -> [_ _ w370 w446 w483 w559]
                    tunnel: w302 -> [_ _ w366 w425 w479 w537]
                    tunnel: w301 -> [_ w317 w345 w416 w461 w527]
                    tunnel: w300 -> [_ _ w343 w426 w459 w538]
                    tunnel: w299 -> [_ _ w344 w427 w460 w539]
                    tunnel: w298 -> [_ _ w361 w414 w475 w533]
                    tunnel: w297 -> [_ _ w356 w435 w473 w547]
                    tunnel: w296 -> [_ w321 _ _ _ _]
                    tunnel: w295 -> [_ w309 w341 _ w454 _]
                    frame "Stop", Default {
                    }
                    frame "Result" {
                      n131 = property on="FullSpeed1 Current" class="DigNum (strict)"() -> ("Value"=w325:dbl)  [unwired: 2 in, 2 out]
                      n132 = property on="FullSpeed2 Current" class="DigNum (strict)"() -> ("Value"=w326:dbl)  [unwired: 2 in, 2 out]
                      n133 = property on="FullSpeed2 Speed" class="DigNum (strict)"() -> ("Value"=w328:dbl)  [unwired: 2 in, 2 out]
                      n134 = property on="FullSpeed1 Speed" class="DigNum (strict)"() -> ("Value"=w327:dbl)  [unwired: 2 in, 2 out]
                      n135 = Subtract(x=w326, y=w325) -> (x-y=w324:dbl)
                      n136 = Absolute Value(x=w324) -> (abs(x)=w313:dbl)
                      n137 = Greater Or Equal?(x=w313, y=u32 5) -> (x >= y?=w319:bool)
                      n138 = Equal?(x=w309, y=u8 95) -> (x = y?=w311:bool)
                      n139 = case shown="True" w311 {
                        tunnel: w328 -> [_ w339]
                        tunnel: w327 -> [_ w338]
                        tunnel: [TRUE w335] -> w320
                        frame False {
                        }
                        frame True {
                          n140 = Subtract(x=w339, y=w338) -> (x-y=w340:dbl)
                          n141 = Absolute Value(x=w340) -> (abs(x)=w337:dbl)
                          n142 = Greater Or Equal?(x=w337, y=500.0) -> (x >= y?=w335:bool)
                        }
                      }
                      n143 = call "Find_Number_LineMARVIN.vi"("Test Paragraph"="4.4", "TableIn"=w321) -> ("Line number"=w318:i32)  [unwired: 3 in, 3 out]
                      n144 = And(x=w320, y=w319) -> (x .and. y?=w310:bool)
                      "VenableDirectionResult" <- w310
                      n145 = call "PassOrFail (SubVI).vi"("String Res"="", "index (row)"=w318, "Data in"=-3.0, "Pass?Fail"=w310, "Table in"=w321) -> ("error out"=w316:errorcluster)  [unwired: 6 in]
                      n146 = property class="Bool (strict)"(reference=w317, error in=w316) -> ("Value"=w333:bool)  [unwired: 2 out]
                      n147 = Select(t=T12."Stop", s=w333, f=T12."Stop") -> (s? t:f=w330:T12)
                    }
                    frame "FullSpeed2" {
                      n148 = Concatenate Strings(w356, "\nFull speed operation " ("string")) -> (w342:string)
                      n149 = Equal?(x=w341, y=u8 95) -> (x = y?=w351:bool)
                      n150 = Select(t=u16 15100, s=w351, f=u16 12100 ("y")) -> (s? t:f=w365:u16)
                      n151 = call "CANSendMotorSpeed.vi"("Remote"=TRUE, "Motor Speed RPM"=w365, "UUT"=w366, "CAN Cluster in"=w370) -> ("error out"=w363:errorcluster)  [unwired: 7 in]
                      n152 = call "Write panel message (SubVI).vi"("Stop BurnIn"=w343, 4:"rpm"=w361, 5:"rpm"=TRUE ("rpm"), "PrintTime"=FALSE, "Stop"=w345, "error in (no error)"=w363, "Time to wait"=0.2, "Strin"=w342, "String in"=w344) -> ("error out"=w348:errorcluster)  [unwired: 2 in]
                      n153 = flat-sequence {
                        tunnel: w348 -> [w377]
                        tunnel: [w377] -> w347
                        tunnel: [w376] -> w346
                        frame #0 {
                          n154 = call <vilib>:"High Resolution Relative Seconds.vi"() -> ("relative seconds"=w376:dbl)
                        }
                      }
                      n155 = Select(t=15000.0, s=w351, f=11500.0) -> (s? t:f=w350:dbl)
                      n156 = Select(t=47.0, s=w351, f=24.0) -> (s? t:f=w349:dbl)
                      n157 = while {
                        tunnel: w361 -> [w379]
                        tunnel: w347 -> [w407]
                        tunnel: [w387] -> w358
                        tunnel: w350 -> [w400]
                        tunnel: w349 -> [w399]
                        tunnel: w346 -> [w395]
                        tunnel: w345 -> [w385]
                        tunnel: w344 -> [w386]
                        tunnel: w343 -> [w383]
                        tunnel: w342 -> [w382]
                        stop <- w397 stop-if-true
                        n158 = call <vilib>:"High Resolution Relative Seconds.vi"() -> ("relative seconds"=w396:dbl)
                        n159 = Subtract(x=w396, y=w395) -> (x-y=w394:dbl)
                        n160 = property class="DigNum (strict)"(reference=w379, error in=w407) -> (error out=w406:errorcluster, "Value"=w401:dbl)  [unwired: 1 out]
                        "FullSpeed2 Speed" <- w401
                        n161 = Greater Or Equal?(x=w394, y=120.0) -> (x >= y?=w392:bool)
                        n162 = Greater Or Equal?(x=w401, y=w400) -> (x >= y?=w391:bool)
                        n163 = property on="VISA Tester" class="VISAName"(error in=w406) -> (error out=w405:errorcluster, "Value"=w404:refnum<visa-resource-name>)  [unwired: 1 in, 1 out]
                        n164 = property class="Bool (strict)"(reference=w385) -> ("Value"=w390:bool)  [unwired: 1 in, 2 out]
                        n165 = call "GetADCTester (SubVI).vi"("error in (no error)"=w405, "GetADCTester"=T13."Current", "TimeToGet"=5, "VISA Refnum in"=w404) -> ("error out"=w402:errorcluster, "ADCValOutput Single"=w398:dbl)  [unwired: 5 in, 1 out]
                        "FullSpeed2 Current" <- w398
                        n166 = Greater Or Equal?(x=w398, y=w399) -> (x >= y?=w388:bool)
                        n167 = And(x=w391, y=w388) -> (x .and. y?=w389:bool)
                        n168 = Compound Arithmetic op=OR(w390, w392, w389) -> (w397:bool)
                        n169 = call "Write panel message (SubVI).vi"("Stop BurnIn"=w383, 4:"rpm"=w379, 5:"rpm"=TRUE ("rpm"), "PrintTime"=FALSE, "Stop"=w385, "error in (no error)"=w402, "Time to wait"=0.2, "Strin"=w382, "String in"=w386) -> ("error out"=w387:errorcluster)  [unwired: 2 in]
                      }
                      n170 = property class="Bool (strict)"(reference=w345, error in=w358) -> ("Value"=w375:bool)  [unwired: 2 out]
                      n171 = Select(t=T12."Stop", s=w375, f=T12."Result") -> (s? t:f=w372:T12)
                    }
                    frame "MD[1]=1" {
                      n172 = Concatenate Strings(w435, "\nSet Parameters MD[1]=1" ("Strin")) -> (w424:string)
                      n173 = property on="VISA Tester" class="VISAName"() -> ("Value"=w440:refnum<visa-resource-name>)  [unwired: 2 in, 2 out]
                      n174 = call "TesterOption (SubVI).vi"("2 Options"=FALSE, "On/Off"=FALSE, "Tester Option"=T11."Venable", "VISA Refnum in"=w440) -> ("error out"=w441:errorcluster, "VISA Refnum out"=w431:refnum<visa-resource-name>)  [unwired: 6 in]
                      n175 = call "CANSendMotorSpeed.vi"("Remote"=TRUE, "error in (no error)"=w441, "Motor Speed RPM"=u16 0, "UUT"=w425, "CAN Cluster in"=w446) -> ("error out"=w443:errorcluster)  [unwired: 6 in]
                      n176 = call "Write panel message (SubVI).vi"("Stop BurnIn"=w426, 4:"rpm"=w414, 5:"rpm"=FALSE ("rpm"), "PrintTime"=TRUE, "Stop"=w416, "error in (no error)"=w443, "Time to wait"=40.0, "Strin"=w424, "String in"=w427) -> ("error out"=w413:errorcluster)  [unwired: 2 in]
                      n177 = property on="VISA Marvin" class="VISAName"(error in=w413) -> (error out=w442:errorcluster, "Value"=w448:refnum<visa-resource-name>)  [unwired: 1 in, 1 out]
                      n178 = call "SerialMarvinSendGet.vi"("error in (no error)"=w442, "Clear Log"=FALSE, "write buffer"="EP=1\r\nMD[1]=1\r\n", "VISA resource name"=w448) -> ("error out"=w430:errorcluster)  [unwired: 6 in, 1 out]
                      n179 = call "TesterOption (SubVI).vi"("2 Options"=FALSE, "error in (no error)"=w430, "On/Off"=FALSE, "Tester Option"=T11."Power", "VISA Refnum in"=w431) -> ("error out"=w428:errorcluster, "VISA Refnum out"=w417:refnum<visa-resource-name>)  [unwired: 5 in]
                      n180 = call "Write panel message (SubVI).vi"("Stop BurnIn"=w426, 4:"rpm"=w414, 5:"rpm"=FALSE ("rpm"), "PrintTime"=TRUE, "Stop"=w416, "error in (no error)"=w428, "Time to wait"=25.0, "Strin"=w424, "String in"=w427) -> ("error out"=w418:errorcluster)  [unwired: 2 in]
                      n181 = call "TesterOption (SubVI).vi"("2 Options"=FALSE, "error in (no error)"=w418, "On/Off"=TRUE, "Tester Option"=T11."Venable", "VISA Refnum in"=w417) -> ("error out"=w415:errorcluster)  [unwired: 5 in, 1 out]
                      n182 = call "Time Delay8"("error in (no error)"=w415) -> ("error out"=w411:errorcluster)  [unwired: 10 in]
                      n183 = property class="Bool (strict)"(reference=w416, error in=w411) -> ("Value"=w453:bool)  [unwired: 2 out]
                      n184 = Select(t=T12."Stop", s=w453, f=T12."FullSpeed2") -> (s? t:f=w452:T12)
                    }
                    frame "FullSpeed1" {
                      n185 = Concatenate Strings(w473, "\nFull speed operation " ("string")) -> (w458:string)
                      n186 = Equal?(x=w454, y=u8 95) -> (x = y?=w471:bool)
                      n187 = flat-sequence {
                        tunnel: w464 -> [w490]
                        tunnel: [w490] -> w463
                        tunnel: [w489] -> w462
                        frame #0 {
                          n188 = call <vilib>:"High Resolution Relative Seconds.vi"() -> ("relative seconds"=w489:dbl)
                        }
                      }
                      n189 = Select(t=u16 15100, s=w471, f=u16 12100 ("y")) -> (s? t:f=w478:u16)
                      n190 = call "CANSendMotorSpeed.vi"("Remote"=TRUE, "Motor Speed RPM"=w478, "UUT"=w479, "CAN Cluster in"=w483) -> ("error out"=w476:errorcluster)  [unwired: 7 in]
                      n191 = call "Write panel message (SubVI).vi"("Stop BurnIn"=w459, 4:"rpm"=w475, 5:"rpm"=TRUE ("rpm"), "PrintTime"=FALSE, "Stop"=w461, "error in (no error)"=w476, "Time to wait"=0.2, "Strin"=w458, "String in"=w460) -> ("error out"=w464:errorcluster)  [unwired: 2 in]
                      n192 = Select(t=13700.0, s=w471, f=11500.0) -> (s? t:f=w466:dbl)
                      n193 = Select(t=56.0, s=w471, f=33.0) -> (s? t:f=w465:dbl)
                      n194 = while {
                        tunnel: w475 -> [w492]
                        tunnel: w463 -> [w520]
                        tunnel: [w500] -> w474
                        tunnel: w466 -> [w512]
                        tunnel: w465 -> [w509]
                        tunnel: w462 -> [w507]
                        tunnel: w461 -> [w498]
                        tunnel: w460 -> [w499]
                        tunnel: w459 -> [w496]
                        tunnel: w458 -> [w495]
                        stop <- w514 stop-if-true
                        n195 = property class="DigNum (strict)"(reference=w492, error in=w520) -> (error out=w519:errorcluster, "Value"=w513:dbl)  [unwired: 1 out]
                        "FullSpeed1 Speed" <- w513
                        n196 = call <vilib>:"High Resolution Relative Seconds.vi"() -> ("relative seconds"=w508:dbl)
                        n197 = Subtract(x=w508, y=w507) -> (x-y=w506:dbl)
                        n198 = Greater Or Equal?(x=w506, y=120.0) -> (x >= y?=w504:bool)
                        n199 = Greater Or Equal?(x=w513, y=w512) -> (x >= y?=w511:bool)
                        n200 = property on="VISA Tester" class="VISAName"(error in=w519) -> (error out=w518:errorcluster, "Value"=w517:refnum<visa-resource-name>)  [unwired: 1 in, 1 out]
                        n201 = call "GetADCTester (SubVI).vi"("error in (no error)"=w518, "GetADCTester"=T13."Current", "TimeToGet"=5, "VISA Refnum in"=w517) -> ("error out"=w515:errorcluster, "ADCValOutput Single"=w510:dbl)  [unwired: 5 in, 1 out]
                        "FullSpeed1 Current" <- w510
                        n202 = Greater Or Equal?(x=w510, y=w509) -> (x >= y?=w501:bool)
                        n203 = And(x=w501, y=w511) -> (x .and. y?=w502:bool)
                        n204 = property class="Bool (strict)"(reference=w498) -> ("Value"=w503:bool)  [unwired: 1 in, 2 out]
                        n205 = call "Write panel message (SubVI).vi"("Stop BurnIn"=w496, 4:"rpm"=w492, 5:"rpm"=TRUE ("rpm"), "PrintTime"=FALSE, "Stop"=w498, "error in (no error)"=w515, "Time to wait"=0.2, "Strin"=w495, "String in"=w499) -> ("error out"=w500:errorcluster)  [unwired: 2 in]
                        n206 = Compound Arithmetic op=OR(w503, w502, w504) -> (w514:bool)
                      }
                      n207 = property class="Bool (strict)"(reference=w461, error in=w474) -> ("Value"=w488:bool)  [unwired: 2 out]
                      n208 = Select(t=T12."Stop", s=w488, f=T12."MD[1]=1") -> (s? t:f=w485:T12)
                    }
                    frame "MD[1]=0" {
                      n209 = Concatenate Strings(w547, "\nSet Parameters MD[1]=0" ("Strin")) -> (w536:string)
                      n210 = property on="VISA Tester" class="VISAName"() -> ("Value"=w553:refnum<visa-resource-name>)  [unwired: 2 in, 2 out]
                      n211 = call "TesterOption (SubVI).vi"("2 Options"=FALSE, "On/Off"=FALSE, "Tester Option"=T11."Venable", "VISA Refnum in"=w553) -> ("error out"=w554:errorcluster, "VISA Refnum out"=w543:refnum<visa-resource-name>)  [unwired: 6 in]
                      n212 = call "CANSendMotorSpeed.vi"("Remote"=TRUE, "error in (no error)"=w554, "Motor Speed RPM"=u16 0, "UUT"=w537, "CAN Cluster in"=w559) -> ("error out"=w556:errorcluster)  [unwired: 6 in]
                      n213 = call "Write panel message (SubVI).vi"("Stop BurnIn"=w538, 4:"rpm"=w533, 5:"rpm"=FALSE ("rpm"), "PrintTime"=FALSE, "Stop"=w527, "error in (no error)"=w556, "Time to wait"=0.2, "Strin"=w536, "String in"=w539) -> ("error out"=w550:errorcluster)  [unwired: 2 in]
                      n214 = property on="VISA Marvin" class="VISAName"(error in=w550) -> (error out=w555:errorcluster, "Value"=w561:refnum<visa-resource-name>)  [unwired: 1 in, 1 out]
                      n215 = call "SerialMarvinSendGet.vi"("error in (no error)"=w555, "Clear Log"=FALSE, "write buffer"="EP=1\r\nMD[1]=0\r\n", "VISA resource name"=w561) -> ("error out"=w542:errorcluster)  [unwired: 6 in, 1 out]
                      n216 = call "TesterOption (SubVI).vi"("2 Options"=FALSE, "error in (no error)"=w542, "On/Off"=FALSE, "Tester Option"=T11."Power", "VISA Refnum in"=w543) -> ("error out"=w540:errorcluster, "VISA Refnum out"=w528:refnum<visa-resource-name>)  [unwired: 5 in]
                      n217 = call "Write panel message (SubVI).vi"("Stop BurnIn"=w538, 4:"rpm"=w533, 5:"rpm"=FALSE ("rpm"), "PrintTime"=TRUE, "Stop"=w527, "error in (no error)"=w540, "Time to wait"=25.0, "Strin"=w536, "String in"=w539) -> ("error out"=w529:errorcluster)  [unwired: 2 in]
                      n218 = call "TesterOption (SubVI).vi"("2 Options"=FALSE, "error in (no error)"=w529, "On/Off"=TRUE, "Tester Option"=T11."Venable", "VISA Refnum in"=w528) -> ("error out"=w526:errorcluster)  [unwired: 5 in, 1 out]
                      n219 = call "Time Delay4"("error in (no error)"=w526) -> ("error out"=w522:errorcluster)  [unwired: 10 in]
                      n220 = property class="Bool (strict)"(reference=w527, error in=w522) -> ("Value"=w566:bool)  [unwired: 2 out]
                      n221 = Select(t=T12."Stop", s=w566, f=T12."FullSpeed1") -> (s? t:f=w565:T12)
                    }
                  }
                }
                n222 = flat-sequence {
                  tunnel: [enum16{"Stop", "Direction", "Venable", "Start"}."Stop"] -> w285
                  tunnel: w284 -> [_]
                  frame #0 {
                  }
                }
              }
              frame "Venable" {
                n223 = call "Find_Number_LineMARVIN.vi"("Test Paragraph"="4.1", "TableIn"=w570) -> ("Line number"=w578:i32)  [unwired: 3 in, 3 out]
                n224 = for {
                  tunnel: u16[] [5000, 0, 5000] -> [w607] mode=indexing
                  tunnel: bool[] [TRUE, FALSE, TRUE] -> [w602] mode=indexing
                  tunnel: w578 -> [w608]
                  tunnel: w577 -> [w606]
                  tunnel: w576 -> [w605]
                  tunnel: w575 -> [w593]
                  tunnel: w574 -> [w597]
                  tunnel: w572 -> [w596]
                  tunnel: w573 -> [w595]
                  tunnel: w570 -> [w589]
                  tunnel: w569 -> [w587]
                  tunnel: [w586] -> w568 mode=indexing
                  i -> [w609]
                  w611 = 200.0 ("y")
                  n225 = call "CANSendMotorSpeed.vi"("Remote"=TRUE, "Motor Speed RPM"=u16 5000, "UUT"=w605, "CAN Cluster in"=w606) -> ("error out"=w601:errorcluster)  [unwired: 7 in]
                  n226 = property on="VISA Tester" class="VISAName"() -> ("Value"=w600:refnum<visa-resource-name>)  [unwired: 2 in, 2 out]
                  n227 = Add(x=w608, y=w609) -> (x+y=w590:i32)
                  n228 = call "TesterOption (SubVI).vi"("error in (no error)"=w601, "On/Off"=w602, "Tester Option"=T11."Venable", "VISA Refnum in"=w600) -> ("error out"=w599:errorcluster)  [unwired: 6 in, 1 out]
                  n229 = call "Write panel message (SubVI).vi"("Stop BurnIn"=w595, 4:"rpm"=w593, 5:"rpm"=TRUE ("rpm"), "PrintTime"=TRUE, "Stop"=w596, "error in (no error)"=w599, "Time to wait"=15.0, "Strin"=w587, "String in"=w597) -> ("error out"=w598:errorcluster)  [unwired: 2 in]
                  n230 = property class="DigNum (strict)"(reference=w593, error in=w598) -> ("Value"=w588:dbl)  [unwired: 2 out]
                  n231 = Add(x=w607, y=w611) -> (x+y=w613:dbl)
                  n232 = Subtract(x=w607, y=w611) -> (x-y=w612:dbl)
                  n233 = In Range and Coerce(upper limit=w613, x=w588, lower limit=w612) -> (In Range?=w586:bool)  [unwired: 1 out]
                  n234 = call "PassOrFail (SubVI).vi"("index (row)"=w590, "Data in"=w588, "Pass?Fail"=w586, "Table in"=w589) -> ()  [unwired: 7 in, 1 out]
                }
                n235 = property class="Bool (strict)"(reference=w572) -> ("Value"=w585:bool)  [unwired: 1 in, 2 out]
                n236 = And Array Elements(Boolean array=w568) -> (logical AND=→"VenableResult":bool)
                n237 = Select(t=enum16{"Stop", "Direction", "Venable", "Start"}."Stop", s=w585, f=enum16{"Stop", "Direction", "Venable", "Start"}."Direction") -> (s? t:f=w571:enum16{"Stop", "Direction", "Venable", "Start"})
              }
              frame "Start" {
                w632 = "4" ("Test Paragraph")
                n238 = property class="Str"(reference=w623, "Value"=w614) -> (reference out=w633:refnum<vi>, error out=w620:errorcluster)  [unwired: 1 in]
                n239 = call "Table_ScrollaBarMarvin.vi"("error in"=w620, "Line to focus"=w632, "reference in"=w624) -> ("error out"=w629:errorcluster)  [unwired: 2 out]
                n240 = call "Reset old test Values (SubVI).vi"("error in"=w629, "Atr in"=w624, "Test Paragraph"=w632) -> ("error out"=w628:errorcluster)  [unwired: 8 in]
                n241 = property on="VISA Tester" class="VISAName"(error in=w628) -> (error out=w627:errorcluster, "Value"=w626:refnum<visa-resource-name>)  [unwired: 1 in, 1 out]
                n242 = property class="Bool (strict)"(reference=w617) -> ("Value"=w637:bool)  [unwired: 1 in, 2 out]
                n243 = call "TesterOption (SubVI).vi"("error in (no error)"=w627, "On/Off"=TRUE, "Tester Option"=T11."Venable", "VISA Refnum in"=w626) -> ("error out"=w625:errorcluster)  [unwired: 6 in, 1 out]
                n244 = Select(t=enum16{"Stop", "Direction", "Venable", "Start"}."Stop", s=w637, f=enum16{"Stop", "Direction", "Venable", "Start"}."Venable") -> (s? t:f=w621:enum16{"Stop", "Direction", "Venable", "Start"})
                n245 = call "Write panel message (SubVI).vi"("Stop BurnIn"=w616, 4:"rpm"=w615, 5:"rpm"=FALSE ("rpm"), "PrintTime"=FALSE, "Stop"=w617, "error in (no error)"=w625, "Time to wait"=0.2, "Strin"=w614, "String in"=w633) -> ()  [unwired: 2 in, 1 out]
              }
            }
          }
        }
        frame "Speed Command" {
          w642 = "5. Speed Command Test in process..." ("Value")
          w639 = "5" ("Test Paragraph")
          n246 = control-ref of="Pannel User Message"() -> (w654:refnum<vi>)
          n247 = property class="Str"(reference=w654, error in=w653, "Value"=w642) -> (error out=w652:errorcluster)  [unwired: 1 out]
          n248 = call "Table_ScrollaBarMarvin.vi"("error in"=w652, "Line to focus"=w639, "reference in"=w638) -> ("error out"=w655:errorcluster)  [unwired: 2 out]
          n249 = property class="Tbl (strict)"(reference=w638, error in=w655) -> (error out=w657:errorcluster, "Value"=w658:string[][])  [unwired: 1 out]
          n250 = Index Array(array=w658, index (col)=0 ("disabled index (col)")) -> (element=w659:string[])  [unwired: 1 in]
          n251 = call "Find_Number_Line.vi"("error in"=w657, "Test Paragraph"=w639, "Row Headers[]"=w659) -> ("error out"=w640:errorcluster, "Line number"=w643:i32)  [unwired: 1 out]
          n252 = call "Reset old test Values (SubVI).vi"("error in"=w640, "Atr in"=w638, "Test Paragraph"=w639) -> ()  [unwired: 8 in, 1 out]
          n253 = control-ref of="Pannel User Message"() -> (w647:refnum<vi>)
          n254 = control-ref of="Stop Burn-in"() -> (w651:refnum<vi>)
          n255 = control-ref of="Config_CANAT"() -> (w648:refnum<vi>)
          n256 = control-ref of="Motor Speed RPM"() -> (w649:refnum<vi>)
          n257 = control-ref of="UUT"() -> (w650:refnum<vi>)
          n258 = control-ref of="Stop Button"() -> (w645:refnum<vi>)
          n259 = control-ref of="ATR"() -> (w646:refnum<vi>)
          n260 = property on="UUT" class="DigNum (strict)"() -> ("Value"=w641:u8)  [unwired: 2 in, 2 out]
          n261 = while {
            shift-right: [w671] -> _
            shift-left: enum16{"Stop", "StopTime", "Speeds", "Start"}."Start" -> [w672]
            tunnel: w645 -> [w670]
            tunnel: w646 -> [w669]
            tunnel: w647 -> [w668]
            tunnel: w648 -> [w667]
            tunnel: w649 -> [w666]
            tunnel: w650 -> [w665]
            tunnel: w651 -> [w664]
            tunnel: w643 -> [w663]
            tunnel: w642 -> [w662]
            tunnel: w641 -> [w660]
            stop <- w661 stop-if-true
            n262 = case shown="\"Stop\", Default" w672 {
              tunnel: [w676 w705 w746 w790] -> w671
              tunnel: w670 -> [_ w700 w750 w788]
              tunnel: w669 -> [_ w690 w754 _]
              tunnel: w668 -> [_ w701 w751 _]
              tunnel: w667 -> [w674 w703 w753 _]
              tunnel: w666 -> [_ w698 w748 _]
              tunnel: w665 -> [w675 w702 w745 _]
              tunnel: w664 -> [_ w699 w749 _]
              tunnel: w663 -> [_ _ w755 _]
              tunnel: w662 -> [_ _ w752 _]
              tunnel: [w673 w704 w747 FALSE ("Value")] -> w661
              tunnel: w660 -> [_ _ w738 _]
              frame "Stop", Default {
                n263 = flat-sequence {
                  tunnel: w675 -> [w679]
                  tunnel: w674 -> [w678]
                  tunnel: [enum16{"Stop", "StopTime", "Speeds", "Start"}."Stop"] -> w676
                  tunnel: [TRUE] -> w673
                  frame #0 {
                    n264 = call "CANSendMotorSpeed.vi"("Remote"=TRUE, "Motor Speed RPM"=u16 0, "UUT"=w679, "CAN Cluster in"=w678) -> ("error out"=w684:errorcluster)  [unwired: 7 in]
                    n265 = property on="VISA Tester" class="VISAName"() -> ("Value"=w685:refnum<visa-resource-name>)  [unwired: 2 in, 2 out]
                    n266 = call "TesterOption (SubVI).vi"("2 Options"=FALSE, "error in (no error)"=w684, "On/Off"=FALSE, "Tester Option"=T11."Power", "VISA Refnum in"=w685) -> ()  [unwired: 5 in, 2 out]
                  }
                  frame #1 {
                  }
                }
              }
              frame "StopTime" {
                n267 = call "Table_ScrollaBarMarvin.vi"("Line to focus"="6", "reference in"=w690) -> ("error out"=w691:errorcluster)  [unwired: 1 in, 2 out]
                n268 = call "CANSendMotorSpeed.vi"("Remote"=TRUE, "error in (no error)"=w691, "Motor Speed RPM"=u16 0, "UUT"=w702, "CAN Cluster in"=w703) -> ("error out"=w709:errorcluster)  [unwired: 6 in]
                n269 = flat-sequence {
                  tunnel: [w735] -> w708
                  tunnel: w709 -> [w734]
                  tunnel: [w734] -> w710
                  frame #0 {
                    n270 = call <vilib>:"High Resolution Relative Seconds.vi"() -> ("relative seconds"=w735:dbl)
                  }
                }
                n271 = while {
                  tunnel: [w730] -> w704
                  tunnel: w701 -> [w728]
                  tunnel: w700 -> [w727]
                  tunnel: w699 -> [w725]
                  tunnel: w698 -> [w724]
                  tunnel: "6. Stop Time Test in process..." ("Value") -> [w712]
                  tunnel: [w720] -> w688
                  tunnel: w710 -> [w732]
                  tunnel: [w721] -> w696
                  tunnel: w708 -> [w731]
                  tunnel: [w719] -> w692
                  stop <- w711 stop-if-true
                  n272 = call "Write panel message (SubVI).vi"("Stop BurnIn"=w725, 4:"rpm"=w724, 5:"rpm"=TRUE ("rpm"), "PrintTime"=FALSE, "Stop"=w727, "error in (no error)"=w732, "Time to wait"=0.1, "Strin"=w712, "String in"=w728) -> ("error out"=w729:errorcluster)  [unwired: 2 in]
                  n273 = control-ref of="Motor Speed RPM"() -> (w718:refnum<vi>)
                  n274 = property class="DigNum (strict)"(reference=w718, error in=w729) -> (error out=w721:errorcluster, "Value"=w717:dbl)  [unwired: 1 out]
                  n275 = call <vilib>:"High Resolution Relative Seconds.vi"() -> ("relative seconds"=w715:dbl)
                  n276 = property class="Bool (strict)"(reference=w727) -> ("Value"=w730:bool)  [unwired: 1 in, 2 out]
                  n277 = Subtract(x=w715, y=w731) -> (x-y=w719:dbl)
                  n278 = Greater Or Equal?(x=w719, y=50.0) -> (x >= y?=w713:bool)
                  n279 = Less Or Equal?(x=w717, y=0.0) -> (x <= y?=w720:bool)
                  n280 = Compound Arithmetic op=OR(w720, w713, w730) -> (w711:bool)
                }
                "StopTimeResult" <- w688
                n281 = call "Find_Number_LineMARVIN.vi"("Test Paragraph"="6", "TableIn"=w690) -> ("Line number"=w693:i32)  [unwired: 3 in, 3 out]
                n282 = call "PassOrFail (SubVI).vi"("index (row)"=w693, "error in (no error)"=w696, "Data in"=w692, "Pass?Fail"=w688, "Table in"=w690) -> ("error out"=w695:errorcluster)  [unwired: 6 in]
                n283 = flat-sequence {
                  tunnel: [enum16{"Stop", "StopTime", "Speeds", "Start"}."Stop"] -> w705
                  tunnel: w695 -> [_]
                  frame #0 {
                  }
                }
              }
              frame "Speeds" {
                n284 = Equal?(x=w738, y=u8 95) -> (x = y?=w743:bool)
                n285 = Select(t=u16[] [6000, 11500, 15100], s=w743, f=u16[] [6000, 9000, 12100]) -> (s? t:f=w740:u16[])
                n286 = for {
                  tunnel: w740 -> [w781] mode=indexing
                  tunnel: w755 -> [w774]
                  tunnel: w754 -> [w773]
                  tunnel: w745 -> [w772]
                  tunnel: w753 -> [w771]
                  tunnel: w752 -> [w770]
                  tunnel: w751 -> [w769]
                  tunnel: w750 -> [w768]
                  tunnel: w749 -> [w766]
                  tunnel: w748 -> [w764]
                  tunnel: [w762] -> w747
                  tunnel: [w761] -> w739
                  tunnel: [w760] -> w737 mode=indexing
                  i -> [w780]
                  stop <- w762 stop-if-true
                  w782 = 200.0 ("y")
                  n287 = Increment(x=w780) -> (x+1=w779:i32)
                  n288 = Add(x=w774, y=w779) -> (x+y=w775:i32)
                  n289 = call "CANSendMotorSpeed.vi"("Remote"=TRUE, "Motor Speed RPM"=w781, "UUT"=w772, "CAN Cluster in"=w771) -> ("error out"=w786:errorcluster)  [unwired: 7 in]
                  n290 = control-ref of="Motor Speed RPM"() -> (w787:refnum<vi>)
                  n291 = call "Write panel message (SubVI).vi"("Stop BurnIn"=w766, 4:"rpm"=w764, 5:"rpm"=TRUE ("rpm"), "PrintTime"=TRUE, "Stop"=w768, "error in (no error)"=w786, "Time to wait"=25.0 ("Delay Time (sec)"), "Strin"=w770, "String in"=w769) -> ("error out"=w778:errorcluster)  [unwired: 2 in]
                  n292 = property class="DigNum (strict)"(reference=w787, error in=w778) -> (error out=w785:errorcluster, "Value"=w763:dbl)  [unwired: 1 out]
                  n293 = property class="Bool (strict)"(reference=w768) -> ("Value"=w762:bool)  [unwired: 1 in, 2 out]
                  n294 = Add(x=w781, y=w782) -> (x+y=w784:dbl)
                  n295 = Subtract(x=w781, y=w782) -> (x-y=w783:dbl)
                  n296 = In Range and Coerce(upper limit=w784, x=w763, lower limit=w783) -> (In Range?=w760:bool)  [unwired: 1 out]
                  n297 = call "PassOrFail (SubVI).vi"("index (row)"=w775, "error in (no error)"=w785, "Data in"=w763, "Pass?Fail"=w760, "Table in"=w773) -> ("error out"=w761:errorcluster)  [unwired: 6 in]
                }
                n298 = flat-sequence {
                  tunnel: w747 -> [w759]
                  tunnel: [w757] -> w746
                  tunnel: w739 -> [_]
                  frame #0 {
                    n299 = Select(t=enum16{"Stop", "StopTime", "Speeds", "Start"}."Stop", s=w759, f=enum16{"Stop", "StopTime", "Speeds", "Start"}."StopTime") -> (s? t:f=w757:enum16{"Stop", "StopTime", "Speeds", "Start"})
                  }
                }
                n300 = And Array Elements(Boolean array=w737) -> (logical AND=→"SpeedResult":bool)
              }
              frame "Start" {
                n301 = property on="VISA Tester" class="VISAName"() -> ("Value"=w798:refnum<visa-resource-name>)  [unwired: 2 in, 2 out]
                n302 = call "TesterOption (SubVI).vi"("2 Options"=FALSE, "On/Off"=TRUE, "Tester Option"=T11."Venable", "VISA Refnum in"=w798) -> ("error out"=w789:errorcluster)  [unwired: 6 in, 1 out]
                n303 = property class="Bool (strict)"(reference=w788, error in=w789) -> ("Value"=w794:bool)  [unwired: 2 out]
                n304 = Select(t=enum16{"Stop", "StopTime", "Speeds", "Start"}."Stop", s=w794, f=enum16{"Stop", "StopTime", "Speeds", "Start"}."Speeds") -> (s? t:f=w790:enum16{"Stop", "StopTime", "Speeds", "Start"})
              }
            }
          }
        }
        frame "Stop Time" {
          w802 = "3. Motor Temperature test in process..." ("Value")
          w800 = "3" ("Test Paragraph")
          n305 = control-ref of="Pannel User Message"() -> (w810:refnum<vi>)
          n306 = property class="Str"(reference=w810, error in=w809, "Value"=w802) -> (error out=w808:errorcluster)  [unwired: 1 out]
          n307 = call "Table_ScrollaBarMarvin.vi"("error in"=w808, "Line to focus"=w800, "reference in"=w799) -> ("error out"=w812:errorcluster)  [unwired: 2 out]
          n308 = property class="Tbl (strict)"(reference=w799, error in=w812) -> (reference out=w805:refnum<vi>, error out=w814:errorcluster, "Value"=w815:string[][])
          n309 = Index Array(array=w815, index (col)=0 ("disabled index (col)")) -> (element=w816:string[])  [unwired: 1 in]
          n310 = call "Find_Number_LineMARVIN.vi"("Test Paragraph"=w800, "error in"=w814, "TableIn"=w799, "Row Headers[]"=w816) -> ("error out"=w811:errorcluster, "Line number"=w804:i32)  [unwired: 1 in, 2 out]
          n311 = call "Reset old test Values (SubVI).vi"("error in"=w811, "Atr in"=w799, "Test Paragraph"=w800) -> ("error out"=w801:errorcluster)  [unwired: 8 in]
          n312 = property on="Status" class="Bool (strict)"(error in=w801) -> (error out=w806:errorcluster, "Value"=w807:bool)  [unwired: 1 in, 1 out]
          n313 = case shown="True" w807 {
            selector: w807 -> [w820 _]
            tunnel: w806 -> [w822 _]
            tunnel: w805 -> [w819 _]
            tunnel: w804 -> [w818 w825]
            tunnel: w803 -> [_ w830]
            tunnel: w802 -> [_ w826]
            frame False {
              n314 = flat-sequence {
                tunnel: w822 -> [w823]
                tunnel: [w823] -> w821
                frame #0 {
                  n315 = One Button Dialog(message="Please establish RS connection.") -> ()  [unwired: 1 in, 1 out]
                }
              }
              n316 = Increment(x=w818) -> (x+1=w817:i32)
              n317 = call "PassOrFail (SubVI).vi"("index (row)"=w817, "error in (no error)"=w821, "Pass?Fail"=w820, "Table in"=w819) -> ()  [unwired: 7 in, 1 out]
            }
            frame True {
              n318 = control-ref of="Stop Burn-in"() -> (w832:refnum<vi>)
              n319 = control-ref of="Pannel User Message"() -> (w834:refnum<vi>)
              n320 = control-ref of="Config_CANAT"() -> (w828:refnum<vi>)
              n321 = control-ref of="ATR"() -> (w835:refnum<vi>)
              n322 = control-ref of="Motor Speed RPM"() -> (w836:refnum<vi>)
              n323 = control-ref of="UUT"() -> (w827:refnum<vi>)
              n324 = control-ref of="Stop Button"() -> (w833:refnum<vi>)
              n325 = property on="VISA Tester" class="VISAName"() -> ("Value"=w829:refnum<visa-resource-name>)  [unwired: 2 in, 2 out]
              n326 = while {
                shift-right: [w840] -> _
                shift-left: T14."Start" -> [w850]
                tunnel: w832 -> [w849]
                tunnel: w833 -> [w848]
                tunnel: w834 -> [w847]
                tunnel: w835 -> [w846]
                tunnel: w836 -> [w845]
                tunnel: w830 -> [w844]
                tunnel: w829 -> [w843]
                tunnel: w828 -> [w842]
                tunnel: w827 -> [w841]
                tunnel: w826 -> [w838]
                tunnel: w825 -> [w837]
                stop <- w839 stop-if-true
                n327 = case shown="\"TA[5]\"" w850 {
                  tunnel: w849 -> [_ w873 w932]
                  tunnel: w848 -> [_ w865 w934]
                  tunnel: w847 -> [_ w874 w936]
                  tunnel: w846 -> [_ w863 _]
                  tunnel: w845 -> [_ w872 w931]
                  tunnel: w844 -> [_ w877 _]
                  tunnel: w843 -> [w853 w876 w925]
                  tunnel: w842 -> [_ _ w942]
                  tunnel: w841 -> [_ _ w941]
                  tunnel: [w851 w866 w927] -> w840
                  tunnel: [w852 FALSE FALSE] -> w839
                  tunnel: w838 -> [_ w875 _]
                  tunnel: w837 -> [_ w862 _]
                  frame "Stop", Default {
                    n328 = flat-sequence {
                      tunnel: w853 -> [w854]
                      tunnel: [TRUE] -> w852
                      tunnel: [T14."Stop"] -> w851
                      frame #0 {
                        n329 = call "TesterOption (SubVI).vi"("2 Options"=FALSE, "On/Off"=FALSE, "Tester Option"=T11."Power", "VISA Refnum in"=w854) -> ()  [unwired: 6 in, 2 out]
                      }
                      frame #1 {
                      }
                    }
                  }
                  frame "TA[5]" {
                    w878 = T17 [enum."60C", enum."90C", enum."120C"] items=["K15", "K16", "K17", "Venable", "Firmeware", "Fan", "Power", "120C", "110C", "100C", "90C", "80C", "70C", "60C", "50C", "40C", "30C", "25C", "20C", "10C", "0C"]
                    n330 = for {
                      tunnel: w878 -> [w902] mode=indexing
                      tunnel: w877 -> [w901]
                      tunnel: w876 -> [w900]
                      tunnel: w875 -> [w899]
                      tunnel: w874 -> [w898]
                      tunnel: w865 -> [w897]
                      tunnel: w873 -> [w896]
                      tunnel: w872 -> [w895]
                      tunnel: dbl[] [60.0, 90.0, 120.0] -> [w885] mode=indexing
                      tunnel: [w884] -> w864
                      tunnel: w863 -> [w891]
                      tunnel: w862 -> [w890]
                      tunnel: [w879] -> w861 mode=indexing
                      i -> [w888]
                      w883 = 3.0 ("y")
                      n331 = for {
                        N: 5 -> [_]
                        tunnel: w902 -> [w904]
                        tunnel: w901 -> [w920]
                        tunnel: w900 -> [w916]
                        tunnel: w899 -> [w914]
                        tunnel: w898 -> [w913]
                        tunnel: w897 -> [w912]
                        tunnel: w896 -> [w910]
                        tunnel: w895 -> [w907]
                        tunnel: [w906] -> w894 mode=indexing
                        tunnel: [w905] -> w892
                        n332 = call "TesterOption (SubVI).vi"("2 Options"=FALSE, "On/Off"=TRUE, "Tester Option"=w904, "VISA Refnum in"=w916) -> ("error out"=w917:errorcluster)  [unwired: 6 in, 1 out]
                        n333 = call "Write panel message (SubVI).vi"("Stop BurnIn"=w910, 4:"rpm"=w907, 5:"rpm"=FALSE ("rpm"), "PrintTime"=FALSE, "Stop"=w912, "error in (no error)"=w917, "Time to wait"=1.0, "Strin"=w914, "String in"=w913) -> ("error out"=w915:errorcluster)  [unwired: 2 in]
                        n334 = call "SerialMarvinSendGet.vi"("error in (no error)"=w915, "write buffer"="TA[2]\r\n", "VISA resource name"=w920) -> ("error out"=w905:errorcluster, "read buffer"=w918:string)  [unwired: 7 in]
                        n335 = Fract/Exp String To Number(string=w918) -> (number=w906:dbl)  [unwired: 3 in, 1 out]
                      }
                      n336 = Increment(x=w888) -> (x+1=w887:i32)
                      n337 = Add Array Elements(numeric array=w894) -> (sum=w893:dbl)
                      n338 = Add(x=w885, y=w883) -> (x+y=w882:dbl)
                      n339 = Subtract(x=w885, y=w883) -> (x-y=w881:dbl)
                      n340 = Divide(x=w893, y=5.0) -> (x/y=w880:dbl)
                      n341 = In Range and Coerce(upper limit=w882, x=w880, lower limit=w881) -> (In Range?=w879:bool)  [unwired: 1 out]
                      n342 = Add(x=w890, y=w887) -> (x+y=w889:i32)
                      n343 = call "PassOrFail (SubVI).vi"("index (row)"=w889, "error in (no error)"=w892, "Data in"=w880, "Pass?Fail"=w879, "Table in"=w891) -> ("error out"=w884:errorcluster)  [unwired: 6 in]
                    }
                    n344 = property class="Bool (strict)"(reference=w865, error in=w864) -> ("Value"=w870:bool)  [unwired: 2 out]
                    n345 = Select(t=T14."Stop", s=w870, f=T14."Stop") -> (s? t:f=w866:T14)
                    n346 = And Array Elements(Boolean array=w861) -> (logical AND=→"MotorTempResult":bool)
                  }
                  frame "Start" {
                    n347 = call "Write panel message (SubVI).vi"("Stop BurnIn"=w932, 4:"rpm"=w931, 5:"rpm"=FALSE ("rpm"), "PrintTime"=FALSE, "Stop"=w934, "Time to wait"=0.1, "Strin"="3. Motor Temperature test in process...\nInitialization state...", "String in"=w936) -> ("error out"=w937:errorcluster)  [unwired: 3 in]
                    n348 = call "TesterOption (SubVI).vi"("2 Options"=FALSE, "error in (no error)"=w937, "On/Off"=FALSE, "Tester Option"=T11."Venable", "VISA Refnum in"=w925) -> ("error out"=w939:errorcluster)  [unwired: 5 in, 1 out]
                    n349 = call "CANSendMotorSpeed.vi"("Remote"=TRUE, "error in (no error)"=w939, "Motor Speed RPM"=u16 0, "UUT"=w941, "CAN Cluster in"=w942) -> ("error out"=w924:errorcluster)  [unwired: 6 in]
                    n350 = property class="Bool (strict)"(reference=w934, error in=w924) -> ("Value"=w946:bool)  [unwired: 2 out]
                    n351 = Select(t=T14."Stop", s=w946, f=T14."TA[5]") -> (s? t:f=w927:T14)
                  }
                }
              }
            }
          }
        }
        frame "Temp Control" {
          w949 = "7. Temperature control test in process..." ("Value")
          w947 = "7" ("Test Paragraph")
          n352 = control-ref of="Pannel User Message"() -> (w961:refnum<vi>)
          n353 = property class="Str"(reference=w961, error in=w960, "Value"=w949) -> (error out=w959:errorcluster)  [unwired: 1 out]
          n354 = control-ref of="Pannel User Message"() -> (w954:refnum<vi>)
          n355 = control-ref of="Motor Speed RPM"() -> (w952:refnum<vi>)
          n356 = control-ref of="Stop Button"() -> (w956:refnum<vi>)
          n357 = control-ref of="ATR"() -> (w955:refnum<vi>)
          n358 = control-ref of="Config_CANAT"() -> (w953:refnum<vi>)
          n359 = control-ref of="UUT"() -> (w951:refnum<vi>)
          n360 = control-ref of="Stop Burn-in"() -> (w950:refnum<vi>)
          n361 = call "Table_ScrollaBarMarvin.vi"("error in"=w959, "Line to focus"=w947, "reference in"=w962) -> ("error out"=w958:errorcluster)  [unwired: 2 out]
          n362 = call "Reset old test Values (SubVI).vi"("error in"=w958, "Atr in"=w962, "Test Paragraph"=w947) -> ("error out"=w948:errorcluster)  [unwired: 8 in]
          n363 = while {
            tunnel: w948 -> [w974]
            shift-right: [w972] -> _
            shift-left: enum16{"Stop", "Algorithm", "Start"}."Start" -> [w973]
            tunnel: w956 -> [w971]
            tunnel: w955 -> [w970]
            tunnel: w954 -> [w969]
            tunnel: w953 -> [w968]
            tunnel: w952 -> [w967]
            tunnel: w951 -> [w966]
            tunnel: w950 -> [w964]
            tunnel: w949 -> [w963]
            stop <- w965 stop-if-true
            n364 = case shown="\"Start\"" w973 {
              tunnel: w974 -> [_ _ w1095]
              tunnel: [w975 w995 w1084] -> w972
              tunnel: w971 -> [_ w1006 w1088]
              tunnel: w970 -> [_ w1002 _]
              tunnel: w969 -> [_ w1007 _]
              tunnel: w968 -> [w978 _ w1081]
              tunnel: w967 -> [_ w1003 _]
              tunnel: w966 -> [w977 _ w1080]
              tunnel: [w976 FALSE FALSE] -> w965
              tunnel: w964 -> [_ w1005 _]
              tunnel: w963 -> [_ w1004 _]
              frame "Stop", Default {
                n365 = flat-sequence {
                  tunnel: w978 -> [w983]
                  tunnel: w977 -> [w981]
                  tunnel: [TRUE] -> w976
                  tunnel: [enum16{"Stop", "Algorithm", "Start"}."Stop"] -> w975
                  frame #0 {
                    n366 = call "CANSendMotorSpeed.vi"("Remote"=TRUE, "Motor Speed RPM"=u16 0, "UUT"=w981, "CAN Cluster in"=w983) -> ("error out"=w979:errorcluster)  [unwired: 7 in]
                    n367 = property on="VISA Tester" class="VISAName"() -> ("Value"=w987:refnum<visa-resource-name>)  [unwired: 2 in, 2 out]
                    n368 = call "TesterOption (SubVI).vi"("2 Options"=FALSE, "error in (no error)"=w979, "On/Off"=FALSE, "Tester Option"=T11."Power", "VISA Refnum in"=w987) -> ()  [unwired: 5 in, 2 out]
                  }
                  frame #1 {
                  }
                  frame #2 {
                  }
                }
              }
              frame "Algorithm" {
                w990 = T18 [enum."6000", enum."11500", enum."15100", enum."11500-2", enum."6000-2"] items=["6000", "11500", "15100", "11500-2", "6000-2"]
                # "Speed Goal"
                # "Speed Ind"
                # "Temp Goal"
                # "50 Deg"
                n369 = for {
                  tunnel: w1007 -> [w1034]
                  tunnel: w1006 -> [w1033]
                  tunnel: w1005 -> [w1032]
                  tunnel: w1004 -> [w1031]
                  tunnel: w1003 -> [w1030]
                  tunnel: w1002 -> [w1017]
                  tunnel: string[] ["7.1", "7.3", "7.5", "7.7", "7.9"] -> [w1015] mode=indexing
                  shift-right: [w1027] -> _
                  shift-left: 1202.0 ("Rt") -> [w1028]
                  tunnel: dbl[] [68.0, 68.0, 88.0, 80.0, 60.0] -> [w1026] mode=indexing
                  tunnel: dbl[] [6000.0, 11500.0, 15100.0, 11500.0, 6000.0] -> [w1025] mode=indexing
                  tunnel: dbl[] [6000.0, 6400.0, 11700.0, 14600.0, 11000.0] -> [w1024] mode=indexing
                  tunnel: [w1013] -> w996
                  tunnel: [w1012] -> w992 mode=indexing
                  tunnel: [w1011] -> w993 mode=indexing
                  tunnel: w990 -> [w1010] mode=indexing
                  stop <- w1029 stop-if-true
                  n370 = call <vilib>:"High Resolution Relative Seconds.vi"() -> ("relative seconds"=w1023:dbl)
                  n371 = while {
                    tunnel: w1034 -> [w1062]
                    tunnel: w1033 -> [w1054]
                    tunnel: w1032 -> [w1061]
                    tunnel: w1031 -> [w1040]
                    tunnel: w1030 -> [w1063]
                    shift-right: [w1059] -> w1027
                    shift-left: w1028 -> [w1058]
                    tunnel: w1010 -> [w1060]
                    tunnel: w1026 -> [w1057]
                    tunnel: w1025 -> [w1056]
                    tunnel: w1024 -> [w1055]
                    tunnel: w1023 -> [w1051]
                    tunnel: [w1046] -> w1018
                    tunnel: [w1045] -> w1011
                    tunnel: [w1044] -> w1016
                    tunnel: [w1043] -> w1012
                    tunnel: [w1042] -> w1014
                    stop <- w1052 stop-if-true
                    n372 = call "DegToDAC (SubVI).vi"("R2"=0.0, "Rt"=w1058) -> ("error out"=w1070:errorcluster, "output array"=w1071:u8[])  [unwired: 8 in]
                    n373 = call <vilib>:"High Resolution Relative Seconds.vi"() -> ("relative seconds"=w1050:dbl)
                    n374 = property on="VISA Tester" class="VISAName"() -> ("Value"=w1073:refnum<visa-resource-name>)  [unwired: 2 in, 2 out]
                    n375 = Byte Array To String(unsigned byte array=w1071) -> (string=w1072:string)
                    n376 = Subtract(x=w1051, y=w1050) -> (x-y=w1049:dbl)
                    n377 = VISA Write(VISA resource name=w1073, write buffer=w1072, error in (no error)=w1070) -> (error out=w1069:errorcluster)  [unwired: 2 out]
                    n378 = Greater Or Equal?(x=w1049, y=120.0) -> (x >= y?=w1047:bool)
                    n379 = call <vilib>:"Clear Errors.vi"("error in (no error)"=w1069) -> ("error out"=w1068:errorcluster)  [unwired: 5 in, 1 out]
                    n380 = control-ref of="Ambient Temperature"() -> (w1041:refnum<vi>)
                    n381 = property class="DigNum (strict)"(reference=w1041) -> ("Value"=w1039:dbl)  [unwired: 1 in, 2 out]
                    n382 = property class="Bool (strict)"(reference=w1054) -> ("Value"=w1053:bool)  [unwired: 1 in, 2 out]
                    n383 = Number To Fractional String(number=w1039, precision (6)=i16 2) -> (F-format string=w1036:string)  [unwired: 2 in]
                    n384 = Concatenate Strings(w1040, "\nAmbient  Temp. [C]: " ("string"), w1036) -> (w1035:string)
                    n385 = call "Write panel message (SubVI).vi"("Stop BurnIn"=w1061, 4:"rpm"=w1063, 5:"rpm"=TRUE ("rpm"), "PrintTime"=TRUE, "Stop"=w1054, "error in (no error)"=w1068, "Time to wait"=3.0, "Strin"=w1035, "String in"=w1062) -> ("error out"=w1067:errorcluster)  [unwired: 2 in]
                    n386 = call "TempAlgoTest (SubVI).vi"("Temp"=w1041, "Speed Ind"=w1055, "Motor Speed RPM"=w1063, "Round"=w1060, "Temp Up In"=w1058, "error in (no error)"=w1067, "String in"=w1062, "Temp Goal"=w1057, "Stop"=w1054, "Speed Goal"=w1056, "Stop BurnIn"=w1061, "Strin"=w1035) -> (14:"Speed Pass/Fail"=w1045:bool, "Temp  Pass/Fail"=w1044:dbl, "Temp Up Out"=w1059:dbl, 17:"Speed Pass/Fail"=w1046:dbl, "Temp Pass/Fail"=w1043:bool, "error out"=w1042:errorcluster)  [unwired: 2 in]
                    n387 = Compound Arithmetic op=OR(w1047, w1045, w1053) -> (w1052:bool)
                  }
                  n388 = property class="Bool (strict)"(reference=w1033) -> ("Value"=w1029:bool)  [unwired: 1 in, 2 out]
                  n389 = call "Find_Number_LineMARVIN.vi"("Test Paragraph"=w1015, "error in"=w1014, "TableIn"=w1017) -> ("error out"=w1019:errorcluster, "Line number"=w1022:i32)  [unwired: 2 in, 2 out]
                  n390 = Increment(x=w1022) -> (x+1=w1021:i32)
                  n391 = call "PassOrFail (SubVI).vi"("index (row)"=w1021, "error in (no error)"=w1019, "Data in"=w1016, "Pass?Fail"=w1012, "Table in"=w1017) -> ("error out"=w1020:errorcluster)  [unwired: 6 in]
                  n392 = call "PassOrFail (SubVI).vi"("index (row)"=w1022, "error in (no error)"=w1020, "Data in"=w1018, "Pass?Fail"=w1011, "Table in"=w1017) -> ("error out"=w1013:errorcluster)  [unwired: 6 in]
                }
                n393 = Build Array (concatenate)(w993, w992) -> (w994:bool[])
                n394 = flat-sequence {
                  tunnel: w996 -> [_]
                  tunnel: [enum16{"Stop", "Algorithm", "Start"}."Stop"] -> w995
                  frame #0 {
                  }
                }
                n395 = And Array Elements(Boolean array=w994) -> (logical AND=→"TempControlResult":bool)
              }
              frame "Start" {
                n396 = call <vilib>:"Clear Errors.vi"("error in (no error)"=w1095) -> ("error out"=w1077:errorcluster)  [unwired: 5 in, 1 out]
                n397 = property on="VISA Tester" class="VISAName"() -> ("Value"=w1094:refnum<visa-resource-name>)  [unwired: 2 in, 2 out]
                n398 = call "TesterOption (SubVI).vi"("On/Off 2"=TRUE, "Tester Option 2"=T11."Venable", "2 Options"=TRUE, "error in (no error)"=w1077, "On/Off"=TRUE, "Tester Option"=T11."K16", "VISA Refnum in"=w1094) -> ("error out"=w1076:errorcluster)  [unwired: 3 in, 1 out]
                n399 = call "Time Delay12"("error in (no error)"=w1076) -> ("error out"=w1075:errorcluster)  [unwired: 10 in]
                n400 = call "CANSendMotorSpeed.vi"("Remote"=FALSE, "error in (no error)"=w1075, "Motor Speed RPM"=u16 0, "UUT"=w1080, "CAN Cluster in"=w1081) -> ("error out"=w1082:errorcluster)  [unwired: 6 in]
                n401 = property class="Bool (strict)"(reference=w1088, error in=w1082) -> ("Value"=w1087:bool)  [unwired: 2 out]
                n402 = Select(t=enum16{"Stop", "Algorithm", "Start"}."Stop", s=w1087, f=enum16{"Stop", "Algorithm", "Start"}."Algorithm") -> (s? t:f=w1084:enum16{"Stop", "Algorithm", "Start"})
              }
            }
          }
        }
        frame "Burn in" {
          n403 = control-ref of="Stop Button"() -> (w1099:refnum<vi>)
          n404 = control-ref of="Pannel User Message"() -> (w1102:refnum<vi>)
          n405 = control-ref of="ATR"() -> (w1098:refnum<vi>)
          n406 = control-ref of="Config_CANAT"() -> (w1101:refnum<vi>)
          n407 = control-ref of="UUT"() -> (w1100:refnum<vi>)
          n408 = control-ref of="Stop Burn-in"() -> (w1097:refnum<vi>)
          n409 = property on="UUT" class="DigNum (strict)"() -> ("Value"=w1096:u8)  [unwired: 2 in, 2 out]
          n410 = while {
            tunnel: w1102 -> [w1113]
            tunnel: w1098 -> [w1112]
            tunnel: w1101 -> [w1111]
            tunnel: w1100 -> [w1110]
            tunnel: w1099 -> [w1109]
            shift-right: [w1108] -> _
            shift-left: T15."Start" -> [w1115]
            shift-right: [w1114] -> _
            shift-left: _ -> [w1106]
            tunnel: w1097 -> [w1105]
            tunnel: w1096 -> [w1104]
            stop <- w1107 stop-if-true
            n411 = case shown="\"DC Current Measure\"" w1115 {
              tunnel: [w1118 w1152 w1220 w1249 w1282 w1318] -> w1114
              tunnel: w1113 -> [_ w1144 _ _ _ w1317]
              tunnel: w1112 -> [_ w1147 w1193 w1236 w1268 w1304]
              tunnel: w1111 -> [_ w1143 _ _ _ w1316]
              tunnel: w1110 -> [_ w1140 _ _ _ w1295]
              tunnel: w1109 -> [_ _ w1222 w1251 w1286 w1310]
              tunnel: [w1116 T15."Stop" w1223 w1252 w1287 w1306] -> w1108
              tunnel: [w1117 FALSE FALSE FALSE FALSE FALSE] -> w1107
              tunnel: w1106 -> [w1118 w1152 w1220 w1249 w1282 _]
              tunnel: w1105 -> [_ _ _ _ _ w1300]
              tunnel: w1104 -> [_ w1132 w1184 w1228 w1260 w1294]
              frame "Stop", Default {
                n412 = flat-sequence {
                  tunnel: [TRUE] -> w1117
                  tunnel: [T15."Stop"] -> w1116
                  frame #0 {
                    n413 = property on="VISA Tester" class="VISAName"() -> ("Value"=w1122:refnum<visa-resource-name>)  [unwired: 2 in, 2 out]
                    n414 = call "TesterOption (SubVI).vi"("On/Off"=FALSE, "Tester Option"=T11."Power", "VISA Refnum in"=w1122) -> ("error out"=w1119:errorcluster)  [unwired: 7 in, 1 out]
                    n415 = property on="Stop Burn-in" class="Bool (strict)"(error in=w1119, "Visible"=FALSE) -> ()  [unwired: 1 in, 2 out]
                  }
                  frame #1 {
                  }
                }
              }
              frame "BurnIn" {
                w1136 = FALSE ("Stop Burn-in")
                n416 = control-ref of="Motor Speed RPM"() -> (w1146:refnum<vi>)
                n417 = control-ref of="Stop Button"() -> (w1145:refnum<vi>)
                n418 = property on="Stop Burn-in" class="Bool (strict)"("Visible"=TRUE) -> (error out=w1148:errorcluster)  [unwired: 2 in, 1 out]
                n419 = Equal?(x=w1132, y=u8 95) -> (x = y?=w1129:bool)
                n420 = Select(t="8. " ("Test Paragraph"), s=w1129, f="7. " ("Test Paragraph")) -> (s? t:f=w1128:string)
                n421 = Select(t="8.4" ("Test Paragraph"), s=w1129, f="7.4" ("Test Paragraph")) -> (s? t:f=w1133:string)
                n422 = call "Find_Number_LineMARVIN.vi"("Test Paragraph"=w1133, "error in"=w1148, "TableIn"=w1147) -> ("error out"=w1150:errorcluster, "Line number"=w1151:i32)  [unwired: 2 in, 2 out]
                n423 = Select(t=u16 15100, s=w1129, f=u16 12100 ("y")) -> (s? t:f=w1138:u16)
                n424 = for {
                  tunnel: w1150 -> [w1172]
                  tunnel: dbl[] [600.0, 600.0, 600.0] -> [w1176] mode=indexing
                  tunnel: w1151 -> [w1181]
                  tunnel: w1147 -> [w1171]
                  tunnel: w1146 -> [w1170]
                  tunnel: w1145 -> [w1169]
                  tunnel: w1144 -> [w1168]
                  tunnel: w1143 -> [w1164]
                  tunnel: w1140 -> [w1163]
                  tunnel: w1138 -> [w1162]
                  tunnel: [w1160] -> w1137
                  tunnel: w1128 -> [w1157]
                  tunnel: [w1156] -> w1127 mode=indexing
                  i -> [w1178]
                  n425 = call "CANSendMotorSpeed.vi"("Remote"=TRUE, "error in (no error)"=w1172, "Motor Speed RPM"=w1162, "UUT"=w1163, "CAN Cluster in"=w1164) -> ("error out"=w1166:errorcluster)  [unwired: 6 in]
                  n426 = control-ref of="Stop Burn-in"() -> (w1167:refnum<vi>)
                  n427 = Concatenate Strings(w1157, "Burn-in test in process..." ("Strin")) -> (w1158:string)
                  n428 = Add(x=w1181, y=w1178) -> (x+y=w1177:i32)
                  n429 = call "Write panel message (SubVI).vi"("Stop BurnIn"=w1167, 4:"rpm"=w1170, 5:"rpm"=TRUE ("rpm"), "PrintTime"=TRUE, "Stop"=w1169, "error in (no error)"=w1166, "Time to wait"=w1176, "Strin"=w1158, "String in"=w1168) -> ("error out"=w1173:errorcluster)  [unwired: 2 in]
                  n430 = control-ref of="Power transistor Heat sink Temp."() -> (w1182:refnum<vi>)
                  n431 = property on="MaxBurnInTempVal" class="DigNum (strict)"() -> ("Value"=w1180:dbl)  [unwired: 2 in, 2 out]
                  n432 = property class="DigNum (strict)"(reference=w1182, error in=w1173) -> (error out=w1161:errorcluster, "Value"=w1179:dbl)  [unwired: 1 out]
                  n433 = Less Or Equal?(x=w1179, y=w1180) -> (x <= y?=w1156:bool)
                  n434 = call "PassOrFail (SubVI).vi"("index (row)"=w1177, "error in (no error)"=w1161, "Data in"=w1179, "Pass?Fail"=w1156, "Table in"=w1171) -> ("error out"=w1160:errorcluster)  [unwired: 6 in]
                }
                n435 = And Array Elements(Boolean array=w1127) -> (logical AND=→"BurnResult":bool)
                n436 = property on="Stop Burn-in" class="Bool (strict)"(error in=w1137, "Value"=w1136, "Visible"=w1136) -> ()  [unwired: 1 in, 2 out]
              }
              frame "Ambient Temp" {
                w1198 = 2 ("disabled index (col)")
                n437 = control-ref of="Power transistor Heat sink Temp."() -> (w1208:refnum<vi>)
                n438 = Equal?(x=w1184, y=u8 95) -> (x = y?=w1187:bool)
                n439 = Select(t="8.3" ("Test Paragraph"), s=w1187, f="7.3" ("Test Paragraph")) -> (s? t:f=w1185:string)
                n440 = call "Find_Number_LineMARVIN.vi"("Test Paragraph"=w1185, "TableIn"=w1193) -> ("error out"=w1219:errorcluster, "Line number"=w1199:i32)  [unwired: 3 in, 2 out]
                n441 = property class="DigNum (strict)"(reference=w1208, error in=w1219) -> (error out=w1210:errorcluster, "Value"=w1200:dbl)  [unwired: 1 out]
                n442 = Select(t=25.0 ("y"), s=w1187, f=25.0 ("y")) -> (s? t:f=w1209:dbl)
                n443 = Select(t=13.0 ("y"), s=w1187, f=13.0) -> (s? t:f=w1211:dbl)
                n444 = Add(x=w1209, y=w1211) -> (x+y=w1218:dbl)
                n445 = Subtract(x=w1209, y=w1211) -> (x-y=w1217:dbl)
                n446 = In Range and Coerce(upper limit=w1218, x=w1200, lower limit=w1217) -> (In Range?=w1183:bool)  [unwired: 1 out]
                "BurnTemp" <- w1183
                n447 = call "PassOrFail (SubVI).vi"("index (row)"=w1199, "error in (no error)"=w1210, "Data in"=w1200, "Pass?Fail"=w1183, "Table in"=w1193) -> ("error out"=w1190:errorcluster)  [unwired: 6 in]
                n448 = property class="Tbl (strict)"(reference=w1193, error in=w1190) -> (reference out=w1192:refnum<vi>, error out=w1207:errorcluster, "Value"=w1206:string[][])
                n449 = Add(x=w1200, y=25.0) -> (x+y=w1191:dbl)
                "MaxBurnInTempVal" <- w1191
                n450 = Number To Fractional String(number=w1191, precision (6)=i16 0) -> (F-format string=w1205:string)  [unwired: 2 in]
                n451 = Concatenate Strings("< " ("string"), w1205) -> (w1194:string)
                n452 = Increment(x=w1199) -> (x+1=w1197:i32)
                n453 = Increment(x=w1197) -> (x+1=w1196:i32)
                n454 = Increment(x=w1196) -> (x+1=w1195:i32)
                n455 = Replace Array Subset(array=w1206, new element #1=w1194, index (row) #1=w1197, index (col) #1=w1198, new element #2=w1194, index (row) #2=w1196, index (col) #2=w1198, new element #3=w1194, index (row) #3=w1195, index (col) #3=w1198) -> (w1204:string[][])
                n456 = property class="Tbl (strict)"(reference=w1192, error in=w1207, "Value"=w1204) -> (error out=w1189:errorcluster)  [unwired: 1 out]
                n457 = property class="Bool (strict)"(reference=w1222, error in=w1189) -> ("Value"=w1226:bool)  [unwired: 2 out]
                n458 = Select(t=T15."Stop", s=w1226, f=T15."BurnIn") -> (s? t:f=w1223:T15)
              }
              frame "MotorSpeed" {
                n459 = control-ref of="Motor Speed RPM"() -> (w1234:refnum<vi>)
                n460 = Equal?(x=w1228, y=u8 95) -> (x = y?=w1231:bool)
                n461 = Select(t="8.2" ("Test Paragraph"), s=w1231, f="7.2" ("Test Paragraph")) -> (s? t:f=w1229:string)
                n462 = call "Find_Number_LineMARVIN.vi"("Test Paragraph"=w1229, "TableIn"=w1236) -> ("error out"=w1248:errorcluster, "Line number"=w1239:i32)  [unwired: 3 in, 2 out]
                n463 = property class="DigNum (strict)"(reference=w1234, error in=w1248) -> (error out=w1237:errorcluster, "Value"=w1238:dbl)  [unwired: 1 out]
                n464 = Select(t=15100.0 ("y"), s=w1231, f=12100.0 ("y")) -> (s? t:f=w1235:dbl)
                n465 = Select(t=200.0 ("y"), s=w1231, f=200.0) -> (s? t:f=w1240:dbl)
                n466 = Add(x=w1235, y=w1240) -> (x+y=w1247:dbl)
                n467 = Subtract(x=w1235, y=w1240) -> (x-y=w1246:dbl)
                n468 = In Range and Coerce(upper limit=w1247, x=w1238, lower limit=w1246) -> (In Range?=w1227:bool)  [unwired: 1 out]
                "BurnSpeed" <- w1227
                n469 = call "PassOrFail (SubVI).vi"("index (row)"=w1239, "error in (no error)"=w1237, "Data in"=w1238, "Pass?Fail"=w1227, "Table in"=w1236) -> ("error out"=w1233:errorcluster)  [unwired: 6 in]
                n470 = property class="Bool (strict)"(reference=w1251, error in=w1233) -> ("Value"=w1255:bool)  [unwired: 2 out]
                n471 = Select(t=T15."Stop", s=w1255, f=T15."Ambient Temp") -> (s? t:f=w1252:T15)
              }
              frame "DC Current Measure" {
                n472 = property on="VISA Tester" class="VISAName"() -> (error out=w1280:errorcluster, "Value"=w1284:refnum<visa-resource-name>)  [unwired: 2 in, 1 out]
                n473 = call "GetADCTester (SubVI).vi"("error in (no error)"=w1280, "GetADCTester"=T13."Current", "TimeToGet"=10, "VISA Refnum in"=w1284) -> ("error out"=w1281:errorcluster, "ADCValOutput Single"=w1267:dbl)  [unwired: 5 in, 1 out]
                n474 = Equal?(x=w1260, y=u8 95) -> (x = y?=w1264:bool)
                n475 = Select(t="8.1" ("Test Paragraph"), s=w1264, f="7.1" ("Test Paragraph")) -> (s? t:f=w1262:string)
                n476 = call "Find_Number_LineMARVIN.vi"("Test Paragraph"=w1262, "error in"=w1281, "TableIn"=w1268) -> ("error out"=w1279:errorcluster, "Line number"=w1269:i32)  [unwired: 2 in, 2 out]
                n477 = Select(t=50.0 ("y"), s=w1264, f=28.0 ("y")) -> (s? t:f=w1271:dbl)
                n478 = Select(t=5.0 ("y"), s=w1264, f=3.0) -> (s? t:f=w1270:dbl)
                n479 = Add(x=w1271, y=w1270) -> (x+y=w1278:dbl)
                n480 = Subtract(x=w1271, y=w1270) -> (x-y=w1277:dbl)
                n481 = In Range and Coerce(upper limit=w1278, x=w1267, lower limit=w1277) -> (In Range?=w1258:bool)  [unwired: 1 out]
                "BurnDC" <- w1258
                n482 = call "PassOrFail (SubVI).vi"("index (row)"=w1269, "error in (no error)"=w1279, "Data in"=w1267, "Pass?Fail"=w1258, "Table in"=w1268) -> ("error out"=w1266:errorcluster)  [unwired: 6 in]
                n483 = property class="Bool (strict)"(reference=w1286, error in=w1266) -> ("Value"=w1257:bool)  [unwired: 2 out]
                n484 = Not(x=w1258) -> (.not. x?=w1256:bool)
                n485 = Or(x=w1256, y=w1257) -> (x .or. y?=w1259:bool)
                n486 = Select(t=T15."Stop", s=w1259, f=T15."MotorSpeed") -> (s? t:f=w1287:T15)
              }
              frame "Start" {
                n487 = Equal?(x=w1294, y=u8 95) -> (x = y?=w1296:bool)
                n488 = Select(t="8" ("Test Paragraph"), s=w1296, f="7" ("Test Paragraph")) -> (s? t:f=w1291:string)
                n489 = Concatenate Strings(w1291, ". Burn-in test in process...\nFull Speed Operation" ("Value")) -> (w1290:string)
                n490 = property class="Str"(reference=w1317, "Value"=w1290) -> (reference out=w1314:refnum<vi>, error out=w1299:errorcluster)  [unwired: 1 in]
                n491 = call "Find_Number_LineMARVIN.vi"("Test Paragraph"=w1291, "error in"=w1299, "TableIn"=w1304) -> ("error out"=w1324:errorcluster, "Line number"=w1325:i32)  [unwired: 2 in, 2 out]
                n492 = Select(t=u16 15100 ("y"), s=w1296, f=u16 12100 ("y")) -> (s? t:f=w1331:u16)
                n493 = call "Table_ScrollaBarMarvin.vi"("error in"=w1324, "Line to focus"=w1291, "reference in"=w1304) -> ("error out"=w1326:errorcluster)  [unwired: 2 out]
                n494 = call "Reset old test Values (SubVI).vi"("error in"=w1326, "Atr in"=w1304, "Test Paragraph"=w1291) -> ("error out"=w1327:errorcluster)  [unwired: 8 in]
                n495 = Increment(x=w1325) -> (x+1=w1318:i32)
                n496 = property on="VISA Tester" class="VISAName"(error in=w1327) -> (error out=w1328:errorcluster, "Value"=w1329:refnum<visa-resource-name>)  [unwired: 1 in, 1 out]
                n497 = call "TesterOption (SubVI).vi"("2 Options"=FALSE, "error in (no error)"=w1328, "On/Off"=TRUE, "Tester Option"=T11."Venable", "VISA Refnum in"=w1329) -> ("error out"=w1330:errorcluster)  [unwired: 5 in, 1 out]
                n498 = call "CANSendMotorSpeed.vi"("Remote"=TRUE, "error in (no error)"=w1330, "Motor Speed RPM"=w1331, "UUT"=w1295, "CAN Cluster in"=w1316) -> ("error out"=w1315:errorcluster)  [unwired: 6 in]
                n499 = control-ref of="Motor Speed RPM"() -> (w1303:refnum<vi>)
                n500 = call "Write panel message (SubVI).vi"("Stop BurnIn"=w1300, 4:"rpm"=w1303, 5:"rpm"=TRUE ("rpm"), "PrintTime"=TRUE, "Stop"=w1310, "error in (no error)"=w1315, "Time to wait"=50.0, "Strin"=w1290, "String in"=w1314) -> ("error out"=w1302:errorcluster)  [unwired: 2 in]
                n501 = property class="Bool (strict)"(reference=w1310, error in=w1302) -> ("Value"=w1309:bool)  [unwired: 2 out]
                n502 = Select(t=T15."Stop", s=w1309, f=T15."DC Current Measure") -> (s? t:f=w1306:T15)
              }
            }
          }
        }
        frame "Visual Inspec" {
          n503 = property on="VISA Tester" class="VISAName"() -> ("Value"=w1342:refnum<visa-resource-name>)  [unwired: 2 in, 2 out]
          n504 = call "TesterOption (SubVI).vi"("2 Options"=FALSE, "error in (no error)"=w1343, "On/Off"=FALSE, "Tester Option"=T11."Power", "VISA Refnum in"=w1342) -> ("error out"=w1338:errorcluster)  [unwired: 5 in, 1 out]
          n505 = local read "UUT"() -> (w1334:u8)
          n506 = Equal?(x=w1334, y=u8 95) -> (x = y?=w1335:bool)
          n507 = case shown="False" w1335 {
            tunnel: w1344 -> [w1348 w1352]
            tunnel: w1338 -> [w1347 w1351]
            tunnel: [w1345 w1350] -> w1337
            tunnel: [w1346 w1349] -> w1333
            frame False {
              n508 = call "VisualInspectionAHU.vi"("error in (no error)"=w1347, "TableRef"=w1348) -> ("error out"=w1346:errorcluster, "VisualInspectionResult"=w1345:bool)  [unwired: 8 in]
            }
            frame True {
              n509 = call "VisualInspectionEBAY.vi"("error in (no error)"=w1351, "TableRef"=w1352) -> ("error out"=w1349:errorcluster, "VisualInspectionResult"=w1350:bool)  [unwired: 8 in]
            }
          }
          "VisualInspectionResult" <- w1337
          n510 = property on="Automation" class="Bool (strict)"(error in=w1333) -> ("Value"=w1332:bool)  [unwired: 1 in, 2 out]
          n511 = case shown="True" w1332 {
            frame False {
            }
            frame True {
              w1353 = TRUE ("Value (Signaling)")
              n512 = property on="SetSN" class="Bool (strict)"("Val(Sgnl)"=w1353, "Value"=w1353) -> ()  [unwired: 2 in, 2 out]
            }
          }
        }
        frame "Temp Sens Cal" {
          w1357 = "2. Temperature sensor calibration test in process..." ("Value")
          w1355 = "2" ("Test Paragraph")
          n513 = control-ref of="Pannel User Message"() -> (w1364:refnum<vi>)
          n514 = property class="Str"(reference=w1364, error in=w1363, "Value"=w1357) -> (error out=w1362:errorcluster)  [unwired: 1 out]
          n515 = call "Table_ScrollaBarMarvin.vi"("error in"=w1362, "Line to focus"=w1355, "reference in"=w1365) -> ("error out"=w1367:errorcluster)  [unwired: 2 out]
          n516 = property class="Tbl (strict)"(reference=w1365, error in=w1367) -> (reference out=w1354:refnum<vi>, error out=w1369:errorcluster, "Value"=w1370:string[][])
          n517 = Index Array(array=w1370, index (col)=0 ("disabled index (col)")) -> (element=w1371:string[])  [unwired: 1 in]
          n518 = call "Find_Number_Line.vi"("error in"=w1369, "Test Paragraph"=w1355, "Row Headers[]"=w1371) -> ("error out"=w1366:errorcluster, "Line number"=w1359:i32)  [unwired: 1 out]
          n519 = property on="Status" class="Bool (strict)"(error in=w1366) -> (error out=w1360:errorcluster, "Value"=w1361:bool)  [unwired: 1 in, 1 out]
          n520 = call "Reset old test Values (SubVI).vi"("error in"=w1360, "Atr in"=w1354, "Test Paragraph"=w1355) -> ("error out"=w1356:errorcluster)  [unwired: 8 in]
          n521 = case shown="True" w1361 {
            selector: w1361 -> [w1375 _]
            tunnel: w1356 -> [w1377 _]
            tunnel: w1354 -> [w1374 _]
            tunnel: w1359 -> [w1373 _]
            tunnel: w1358 -> [_ w1384]
            tunnel: w1357 -> [_ w1380]
            frame False {
              n522 = flat-sequence {
                tunnel: w1377 -> [w1378]
                tunnel: [w1378] -> w1376
                frame #0 {
                  n523 = One Button Dialog(message="Please establish RS connection.") -> ()  [unwired: 1 in, 1 out]
                }
              }
              n524 = Increment(x=w1373) -> (x+1=w1372:i32)
              n525 = call "PassOrFail (SubVI).vi"("index (row)"=w1372, "error in (no error)"=w1376, "Pass?Fail"=w1375, "Table in"=w1374) -> ()  [unwired: 7 in, 1 out]
            }
            frame True {
              n526 = control-ref of="Stop Burn-in"() -> (w1386:refnum<vi>)
              n527 = control-ref of="Pannel User Message"() -> (w1388:refnum<vi>)
              n528 = control-ref of="Config_CANAT"() -> (w1382:refnum<vi>)
              n529 = control-ref of="ATR"() -> (w1389:refnum<vi>)
              n530 = control-ref of="Motor Speed RPM"() -> (w1390:refnum<vi>)
              n531 = control-ref of="UUT"() -> (w1381:refnum<vi>)
              n532 = control-ref of="Stop Button"() -> (w1387:refnum<vi>)
              n533 = property on="VISA Tester" class="VISAName"() -> ("Value"=w1383:refnum<visa-resource-name>)  [unwired: 2 in, 2 out]
              n534 = while {
                shift-right: [w1393] -> _
                shift-left: T14."Start" -> [w1403]
                tunnel: w1386 -> [w1402]
                tunnel: w1387 -> [w1401]
                tunnel: w1388 -> [w1400]
                tunnel: w1389 -> [w1399]
                tunnel: w1390 -> [w1398]
                tunnel: w1384 -> [w1397]
                tunnel: w1383 -> [w1396]
                tunnel: w1382 -> [w1395]
                tunnel: w1381 -> [w1394]
                tunnel: w1380 -> [w1391]
                stop <- w1392 stop-if-true
                n535 = case shown="\"AO[1]=Meas.\"" w1403 {
                  tunnel: w1402 -> [_ w1438 w1465 w1520 w1550]
                  tunnel: w1401 -> [_ w1439 w1457 w1506 w1552]
                  tunnel: w1400 -> [_ w1436 w1466 w1518 w1554]
                  tunnel: w1399 -> [_ w1416 _ _ _]
                  tunnel: w1398 -> [_ w1440 w1464 w1521 w1549]
                  tunnel: w1397 -> [_ w1449 w1469 w1530 w1546]
                  tunnel: w1396 -> [w1406 w1445 w1468 w1526 w1534]
                  tunnel: w1395 -> [_ _ _ _ w1560]
                  tunnel: w1394 -> [_ _ _ _ w1559]
                  tunnel: [w1404 w1425 w1458 w1509 w1537] -> w1393
                  tunnel: [w1405 FALSE FALSE FALSE FALSE] -> w1392
                  tunnel: w1391 -> [_ _ w1467 _ _]
                  frame "Stop", Default {
                    n536 = flat-sequence {
                      tunnel: w1406 -> [w1407]
                      tunnel: [TRUE] -> w1405
                      tunnel: [T14."Stop"] -> w1404
                      frame #0 {
                        n537 = call "TesterOption (SubVI).vi"("2 Options"=FALSE, "On/Off"=FALSE, "Tester Option"=T11."Power", "VISA Refnum in"=w1407) -> ()  [unwired: 6 in, 2 out]
                      }
                      frame #1 {
                      }
                    }
                  }
                  frame "AO[1]=Meas." {
                    n538 = property on="AO[1]Meas" class="DigNum (strict)"() -> ("Value"=w1419:dbl)  [unwired: 2 in, 2 out]
                    n539 = Number To Fractional String(number=w1419) -> (F-format string=w1427:string)  [unwired: 3 in]
                    n540 = Search and Replace String(input string="EP=1\r\nAO[1]=0\r\n" ("write buffer"), search string="0", replace string=w1427) -> (result string=w1426:string)  [unwired: 5 in, 3 out]
                    n541 = call "SerialMarvinSendGet.vi"("Clear Log"=FALSE, "write buffer"=w1426, "VISA resource name"=w1449) -> ("error out"=w1444:errorcluster)  [unwired: 7 in, 1 out]
                    n542 = call "TesterOption (SubVI).vi"("2 Options"=FALSE, "error in (no error)"=w1444, "On/Off"=FALSE, "Tester Option"=T11."Power", "VISA Refnum in"=w1445) -> ("error out"=w1443:errorcluster, "VISA Refnum out"=w1430:refnum<visa-resource-name>)  [unwired: 5 in]
                    n543 = call "Write panel message (SubVI).vi"("Stop BurnIn"=w1438, 4:"rpm"=w1440, 5:"rpm"=FALSE ("rpm"), "PrintTime"=TRUE, "Stop"=w1439, "error in (no error)"=w1443, "Time to wait"=20.0, "Strin"="2. Temperature sensor calibration test in process...\nSet Parameters...", "String in"=w1436) -> ("error out"=w1431:errorcluster)  [unwired: 2 in]
                    n544 = call "TesterOption (SubVI).vi"("2 Options"=FALSE, "error in (no error)"=w1431, "On/Off"=FALSE, "Tester Option"=T11."Venable", "VISA Refnum in"=w1430) -> ("error out"=w1424:errorcluster)  [unwired: 5 in, 1 out]
                    n545 = flat-sequence {
                      tunnel: [T14."Stop"] -> w1425
                      tunnel: w1417 -> [_]
                      frame #0 {
                      }
                    }
                    n546 = In Range and Coerce(upper limit=0.1, x=w1419, lower limit=-0.1) -> (In Range?=w1414:bool)  [unwired: 1 out]
                    "SensCalResult" <- w1414
                    n547 = call "Find_Number_LineMARVIN.vi"("Test Paragraph"="2.1", "error in"=w1424, "TableIn"=w1416) -> ("error out"=w1418:errorcluster, "Line number"=w1422:i32)  [unwired: 2 in, 2 out]
                    n548 = call "PassOrFail (SubVI).vi"("Test#"="2", "index (row)"=w1422, "error in (no error)"=w1418, "Data in"=w1419, "Pass?Fail"=w1414, "Table in"=w1416) -> ("error out"=w1417:errorcluster)  [unwired: 5 in]
                  }
                  frame "TA[5]" {
                    w1470 = T17 [enum."50C", enum."80C", enum."100C", enum."120C"] items=["K15", "K16", "K17", "Venable", "Firmeware", "Fan", "Power", "120C", "110C", "100C", "90C", "80C", "70C", "60C", "50C", "40C", "30C", "25C", "20C", "10C", "0C"]
                    n549 = for {
                      tunnel: w1470 -> [w1485] mode=indexing
                      tunnel: w1469 -> [w1484]
                      tunnel: w1468 -> [w1483]
                      tunnel: w1467 -> [w1482]
                      tunnel: w1466 -> [w1481]
                      tunnel: w1457 -> [w1480]
                      tunnel: w1465 -> [w1479]
                      tunnel: w1464 -> [w1478]
                      tunnel: dbl[] [0.59774, 0.65238, 0.68545, 0.71584] -> [w1473] mode=indexing
                      tunnel: [w1472] -> w1453 mode=indexing
                      tunnel: [w1471] -> w1456
                      n550 = for {
                        N: 5 -> [_]
                        tunnel: w1485 -> [w1503]
                        tunnel: w1484 -> [w1502]
                        tunnel: w1483 -> [w1498]
                        tunnel: w1482 -> [w1496]
                        tunnel: w1481 -> [w1495]
                        tunnel: w1480 -> [w1494]
                        tunnel: w1479 -> [w1492]
                        tunnel: w1478 -> [w1489]
                        tunnel: [w1488] -> w1477 mode=indexing
                        tunnel: [w1487] -> w1471
                        n551 = call "TesterOption (SubVI).vi"("2 Options"=FALSE, "On/Off"=TRUE, "Tester Option"=w1503, "VISA Refnum in"=w1498) -> ("error out"=w1499:errorcluster)  [unwired: 6 in, 1 out]
                        n552 = call "Write panel message (SubVI).vi"("Stop BurnIn"=w1492, 4:"rpm"=w1489, 5:"rpm"=FALSE ("rpm"), "PrintTime"=FALSE, "Stop"=w1494, "error in (no error)"=w1499, "Time to wait"=1.0, "Strin"=w1496, "String in"=w1495) -> ("error out"=w1497:errorcluster)  [unwired: 2 in]
                        n553 = call "SerialMarvinSendGet.vi"("error in (no error)"=w1497, "write buffer"="TA[5]\r\n", "VISA resource name"=w1502) -> ("error out"=w1487:errorcluster, "read buffer"=w1500:string)  [unwired: 7 in]
                        n554 = Fract/Exp String To Number(string=w1500) -> (number=w1488:dbl)  [unwired: 3 in, 1 out]
                      }
                      n555 = Add Array Elements(numeric array=w1477) -> (sum=w1476:dbl)
                      n556 = Divide(x=w1476, y=5.0) -> (x/y=w1474:dbl)
                      n557 = Subtract(x=w1474, y=w1473) -> (x-y=w1472:dbl)
                    }
                    n558 = property class="Bool (strict)"(reference=w1457, error in=w1456) -> ("Value"=w1462:bool)  [unwired: 2 out]
                    n559 = Select(t=T14."Stop", s=w1462, f=T14."AO[1]=Meas.") -> (s? t:f=w1458:T14)
                    n560 = Array Size(array=w1453) -> (size(s)=w1452:i32)
                    n561 = Add Array Elements(numeric array=w1453) -> (sum=w1455:dbl)
                    n562 = Divide(x=w1455, y=w1452) -> (x/y=→"AO[1]Meas":dbl)
                  }
                  frame "AO[1]=0" {
                    n563 = call "SerialMarvinSendGet.vi"("write buffer"="EP=1\r\nAO[1]=0\r\n", "VISA resource name"=w1530) -> ("error out"=w1525:errorcluster)  [unwired: 8 in, 1 out]
                    n564 = call "TesterOption (SubVI).vi"("2 Options"=FALSE, "error in (no error)"=w1525, "On/Off"=FALSE, "Tester Option"=T11."Power", "VISA Refnum in"=w1526) -> ("error out"=w1524:errorcluster, "VISA Refnum out"=w1512:refnum<visa-resource-name>)  [unwired: 5 in]
                    n565 = call "Write panel message (SubVI).vi"("Stop BurnIn"=w1520, 4:"rpm"=w1521, 5:"rpm"=FALSE ("rpm"), "PrintTime"=TRUE, "Stop"=w1506, "error in (no error)"=w1524, "Time to wait"=20.0, "Strin"="2. Temperature sensor calibration test in process...\nSet Parameters...", "String in"=w1518) -> ("error out"=w1513:errorcluster)  [unwired: 2 in]
                    n566 = call "TesterOption (SubVI).vi"("2 Options"=FALSE, "error in (no error)"=w1513, "On/Off"=FALSE, "Tester Option"=T11."Venable", "VISA Refnum in"=w1512) -> ("error out"=w1507:errorcluster)  [unwired: 5 in, 1 out]
                    n567 = property class="Bool (strict)"(reference=w1506, error in=w1507) -> ("Value"=w1511:bool)  [unwired: 2 out]
                    n568 = Select(t=T14."Stop", s=w1511, f=T14."TA[5]") -> (s? t:f=w1509:T14)
                  }
                  frame "Start" {
                    n569 = call "Write panel message (SubVI).vi"("Stop BurnIn"=w1550, 4:"rpm"=w1549, 5:"rpm"=FALSE ("rpm"), "PrintTime"=FALSE, "Stop"=w1552, "Time to wait"=0.1, "Strin"="2. Temperature sensor calibration test in process...\nInitialization state...", "String in"=w1554) -> ("error out"=w1555:errorcluster)  [unwired: 3 in]
                    n570 = call "TesterOption (SubVI).vi"("2 Options"=FALSE, "error in (no error)"=w1555, "On/Off"=FALSE, "Tester Option"=T11."Venable", "VISA Refnum in"=w1534) -> ("error out"=w1557:errorcluster)  [unwired: 5 in, 1 out]
                    n571 = call "CANSendMotorSpeed.vi"("Remote"=TRUE, "error in (no error)"=w1557, "Motor Speed RPM"=u16 0, "UUT"=w1559, "CAN Cluster in"=w1560) -> ("error out"=w1544:errorcluster)  [unwired: 6 in]
                    n572 = call "SerialMarvinSendGet.vi"("error in (no error)"=w1544, "write buffer"="AO[1]\r\n", "VISA resource name"=w1546) -> ("error out"=w1533:errorcluster, "read buffer"=w1543:string)  [unwired: 7 in]
                    n573 = Equal?(x=w1543, y="0.0") -> (x = y?=w1535:bool)
                    n574 = property class="Bool (strict)"(reference=w1552, error in=w1533) -> ("Value"=w1564:bool)  [unwired: 2 out]
                    n575 = Select(t=T14."TA[5]", s=w1535, f=T14."AO[1]=0") -> (s? t:f=w1539:T14)
                    n576 = Select(t=T14."Stop", s=w1564, f=w1539) -> (s? t:f=w1537:T14)
                  }
                }
              }
            }
          }
        }
        frame "Auxiliary" {
          w1568 = "9. Auxiliary test in process..." ("Value")
          w1580 = "9" ("Test Paragraph")
          n577 = control-ref of="Pannel User Message"() -> (w1579:refnum<vi>)
          n578 = property class="Str"(reference=w1579, error in=w1576, "Value"=w1568) -> (error out=w1578:errorcluster)  [unwired: 1 out]
          n579 = call "Table_ScrollaBarMarvin.vi"("error in"=w1578, "Line to focus"=w1580, "reference in"=w1577) -> ("error out"=w1586:errorcluster)  [unwired: 2 out]
          n580 = property class="Tbl (strict)"(reference=w1577, error in=w1586) -> (reference out=w1575:refnum<vi>, error out=w1585:errorcluster, "Value"=w1584:string[][])
          n581 = Index Array(array=w1584, index (col)=0 ("disabled index (col)")) -> (element=w1583:string[])  [unwired: 1 in]
          n582 = call "Find_Number_Line.vi"("error in"=w1585, "Test Paragraph"=w1580, "Row Headers[]"=w1583) -> ("error out"=w1581:errorcluster, "Line number"=w1566:i32)  [unwired: 1 out]
          n583 = call "Reset old test Values (SubVI).vi"("error in"=w1581, "Atr in"=w1575, "Test Paragraph"=w1580) -> ("error out"=w1573:errorcluster)  [unwired: 8 in]
          n584 = property on="VISA Tester" class="VISAName"() -> ("Value"=w1567:refnum<visa-resource-name>)  [unwired: 2 in, 2 out]
          n585 = control-ref of="Stop Burn-in"() -> (w1570:refnum<vi>)
          n586 = control-ref of="Stop Button"() -> (w1571:refnum<vi>)
          n587 = control-ref of="Pannel User Message"() -> (w1572:refnum<vi>)
          n588 = control-ref of="ATR"() -> (w1565:refnum<vi>)
          n589 = control-ref of="Config_CANAT"() -> ()  [unwired: 1 out]
          n590 = control-ref of="Motor Speed RPM"() -> (w1569:refnum<vi>)
          n591 = while {
            shift-right: [w1591] -> _
            shift-left: enum16{"Stop", "CoolingON", "HotGunON", "Start"}."Start" -> [w1598]
            tunnel: w1573 -> [w1589]
            tunnel: w1572 -> [w1597]
            tunnel: w1571 -> [w1596]
            tunnel: w1570 -> [w1595]
            tunnel: w1569 -> [w1594]
            tunnel: w1568 -> [w1593]
            tunnel: w1567 -> [w1592]
            tunnel: w1566 -> [w1588]
            tunnel: w1565 -> [w1587]
            stop <- w1590 stop-if-true
            n592 = case shown="\"CoolingON\"" w1598 {
              tunnel: w1597 -> [_ w1644 w1736 w1796]
              tunnel: w1596 -> [_ w1636 w1731 w1782]
              tunnel: w1595 -> [_ w1643 w1735 w1795]
              tunnel: w1594 -> [_ w1642 w1734 w1791]
              tunnel: w1593 -> [_ w1629 w1724 w1790]
              tunnel: w1592 -> [_ w1630 w1725 w1783]
              tunnel: [w1600 w1632 w1727 w1778] -> w1591
              tunnel: [w1599 FALSE FALSE FALSE] -> w1590
              tunnel: w1589 -> [_ w1628 w1723 _]
              tunnel: w1588 -> [_ w1623 w1718 _]
              tunnel: w1587 -> [_ w1619 w1715 _]
              frame "Stop", Default {
                n593 = flat-sequence {
                  tunnel: [enum16{"Stop", "CoolingON", "HotGunON", "Start"}."Stop"] -> w1600
                  tunnel: [TRUE] -> w1599
                  frame #0 {
                    n594 = property on="VISA Tester" class="VISAName"() -> ("Value"=w1604:refnum<visa-resource-name>)  [unwired: 2 in, 2 out]
                    n595 = call "TesterOption (SubVI).vi"("2 Options"=FALSE, "On/Off"=FALSE, "Tester Option"=T11."Power", "VISA Refnum in"=w1604) -> ()  [unwired: 6 in, 2 out]
                  }
                  frame #1 {
                  }
                }
              }
              frame "CoolingON" {
                n596 = while {
                  tunnel: w1644 -> [w1679]
                  tunnel: w1643 -> [w1678]
                  tunnel: w1642 -> [w1674]
                  tunnel: [w1671] -> w1608
                  tunnel: w1636 -> [w1662]
                  tunnel: w1630 -> [w1648]
                  tunnel: w1629 -> [w1666]
                  tunnel: w1628 -> [w1663]
                  shift-right: [w1655] -> _
                  shift-left: 0.0 -> [w1656]
                  shift-right: [w1651] -> w1607
                  shift-left: 0.0 ("Value") -> [w1653]
                  tunnel: [w1646] -> w1611
                  stop <- w1660 stop-if-true
                  n597 = control-ref of="Power transistor Heat sink Temp."() -> (w1672:refnum<vi>)
                  n598 = property class="DigNum (strict)"(reference=w1672, error in=w1663) -> (error out=w1669:errorcluster, "Value"=w1651:dbl)  [unwired: 1 out]
                  n599 = Equal?(x=w1651, y=w1653) -> (x = y?=w1652:bool)
                  n600 = Number To Fractional String(number=w1651, precision (6)=i16 2) -> (F-format string=w1665:string)  [unwired: 2 in]
                  n601 = case shown="True" w1652 {
                    tunnel: w1656 -> [_ w1699]
                    tunnel: [0.0 w1697] -> w1655
                    tunnel: [FALSE w1696] -> w1654
                    frame False {
                    }
                    frame True {
                      n602 = Increment(x=w1699) -> (x+1=w1697:dbl)
                      n603 = Greater Or Equal?(x=w1697, y=300.0) -> (x >= y?=w1696:bool)
                    }
                  }
                  n604 = Concatenate Strings(w1666, "\nPCB Temperature [C]: " ("string"), w1665) -> (w1664:string)
                  n605 = call "Write panel message (SubVI).vi"("Stop BurnIn"=w1678, 4:"rpm"=w1674, 5:"rpm"=FALSE ("rpm"), "PrintTime"=FALSE, "Stop"=w1662, "error in (no error)"=w1669, "Time to wait"=0.2, "Strin"=w1664, "String in"=w1679) -> ("error out"=w1668:errorcluster)  [unwired: 2 in]
                  n606 = property class="Bool (strict)"(reference=w1662) -> ("Value"=w1661:bool)  [unwired: 1 in, 2 out]
                  n607 = Less Or Equal?(x=w1651, y=52.0) -> (x <= y?=w1650:bool)
                  n608 = call "GetADCTester (SubVI).vi"("error in (no error)"=w1668, "GetADCTester"=T13."Fan", "VISA Refnum in"=w1648) -> ("error out"=w1671:errorcluster, "ADCValOutput Single"=w1658:dbl)  [unwired: 6 in, 1 out]
                  n609 = Greater?(x=w1658, y=u32 2400) -> (0:w1647:bool)
                  n610 = case shown="True" w1650 {
                    tunnel: [w1686 w1693] -> w1649
                    tunnel: w1650 -> [w1686 w1693]
                    tunnel: w1648 -> [w1684 w1691]
                    tunnel: [w1680 w1687] -> w1646
                    frame False {
                      n611 = call "Time Delay11"() -> ("error out"=w1683:errorcluster)  [unwired: 11 in]
                      n612 = call "GetADCTester (SubVI).vi"("error in (no error)"=w1683, "GetADCTester"=T13."Fan", "VISA Refnum in"=w1684) -> ("ADCValOutput Single"=w1682:dbl)  [unwired: 6 in, 2 out]
                      n613 = Greater?(x=w1682, y=2400.0) -> (0:w1680:bool)
                    }
                    frame True {
                      n614 = call "Time Delay10"() -> ("error out"=w1690:errorcluster)  [unwired: 11 in]
                      n615 = call "GetADCTester (SubVI).vi"("error in (no error)"=w1690, "GetADCTester"=T13."Fan", "VISA Refnum in"=w1691) -> ("ADCValOutput Single"=w1689:dbl)  [unwired: 6 in, 2 out]
                      n616 = Greater?(x=w1689, y=2400.0) -> (0:w1687:bool)
                    }
                  }
                  n617 = Compound Arithmetic op=OR(w1647, w1661, w1649, w1654) -> (w1660:bool)
                }
                n618 = In Range and Coerce(upper limit=56.0, x=w1607, lower limit=52.0) -> (In Range?=w1610:bool)  [unwired: 1 out]
                n619 = Build Array(w1611, w1610) -> (w1612:bool[])
                n620 = And Array Elements(Boolean array=w1612) -> (logical AND=→"AuxiOFFResult":bool)
                n621 = Add(x=w1623, y=3) -> (x+y=w1621:i32)
                n622 = call "PassOrFail (SubVI).vi"("index (row)"=w1621, "error in (no error)"=w1608, "Data in"=w1607, "Pass?Fail"=w1610, "Table in"=w1619) -> ("error out"=w1625:errorcluster)  [unwired: 6 in]
                n623 = Select(t="OFF", s=w1611, f="ON") -> (s? t:f=w1615:string)
                n624 = Increment(x=w1621) -> (x+1=w1620:i32)
                n625 = call "PassOrFail (SubVI).vi"("String Res"=w1615, "index (row)"=w1620, "error in (no error)"=w1625, "Data in"=-3.0, "Pass?Fail"=w1611, "Table in"=w1619) -> ("error out"=w1624:errorcluster)  [unwired: 5 in]
                n626 = call "TesterOption (SubVI).vi"("On/Off 2"=TRUE, "Tester Option 2"=T11."Power", "2 Options"=FALSE, "error in (no error)"=w1624, "On/Off"=FALSE, "Tester Option"=T11."Venable", "VISA Refnum in"=w1630) -> ("error out"=w1635:errorcluster)  [unwired: 3 in, 1 out]
                n627 = property class="Bool (strict)"(reference=w1636, error in=w1635) -> ("Value"=w1645:bool)  [unwired: 2 out]
                n628 = Select(t=enum16{"Stop", "CoolingON", "HotGunON", "Start"}."Stop", s=w1645, f=enum16{"Stop", "CoolingON", "HotGunON", "Start"}."Stop") -> (s? t:f=w1632:enum16{"Stop", "CoolingON", "HotGunON", "Start"})
              }
              frame "HotGunON" {
                n629 = while {
                  tunnel: w1736 -> [w1769]
                  tunnel: w1735 -> [w1768]
                  tunnel: w1734 -> [w1764]
                  tunnel: [w1760] -> w1705
                  tunnel: w1731 -> [w1751]
                  tunnel: w1725 -> [w1761]
                  tunnel: w1724 -> [w1755]
                  tunnel: w1723 -> [w1752]
                  shift-right: [w1744] -> _
                  shift-left: 0.0 -> [w1745]
                  shift-right: [w1741] -> _
                  shift-left: 0.0 ("Value") -> [w1742]
                  tunnel: [w1739] -> w1703
                  stop <- w1749 stop-if-true
                  n630 = control-ref of="Power transistor Heat sink Temp."() -> (w1762:refnum<vi>)
                  n631 = property class="DigNum (strict)"(reference=w1762, error in=w1752) -> (error out=w1758:errorcluster, "Value"=w1741:dbl)  [unwired: 1 out]
                  n632 = Equal?(x=w1741, y=w1742) -> (x = y?=w1740:bool)
                  n633 = Number To Fractional String(number=w1741, precision (6)=i16 2) -> (F-format string=w1754:string)  [unwired: 2 in]
                  n634 = case shown="True" w1740 {
                    tunnel: w1745 -> [_ w1775]
                    tunnel: [0.0 w1773] -> w1744
                    tunnel: [FALSE w1772] -> w1743
                    frame False {
                    }
                    frame True {
                      n635 = Increment(x=w1775) -> (x+1=w1773:dbl)
                      n636 = Greater Or Equal?(x=w1773, y=300.0) -> (x >= y?=w1772:bool)
                    }
                  }
                  n637 = Concatenate Strings(w1755, "\nPCB Temperature [C]: " ("string"), w1754) -> (w1753:string)
                  n638 = call "Write panel message (SubVI).vi"("Stop BurnIn"=w1768, 4:"rpm"=w1764, 5:"rpm"=FALSE ("rpm"), "PrintTime"=FALSE, "Stop"=w1751, "error in (no error)"=w1758, "Time to wait"=0.2, "Strin"=w1753, "String in"=w1769) -> ("error out"=w1757:errorcluster)  [unwired: 2 in]
                  n639 = property class="Bool (strict)"(reference=w1751) -> ("Value"=w1750:bool)  [unwired: 1 in, 2 out]
                  n640 = call "GetADCTester (SubVI).vi"("error in (no error)"=w1757, "GetADCTester"=T13."Fan", "VISA Refnum in"=w1761) -> ("error out"=w1760:errorcluster, "ADCValOutput Single"=w1747:dbl)  [unwired: 6 in, 1 out]
                  n641 = Greater Or Equal?(x=w1741, y=61.0) -> (x >= y?=w1738:bool)
                  n642 = Less?(x=w1747, y=u32 100) -> (x < y?=w1739:bool)
                  n643 = Compound Arithmetic op=OR(w1739, w1750, w1738, w1743) -> (w1749:bool)
                }
                n644 = control-ref of="Power transistor Heat sink Temp."() -> (w1708:refnum<vi>)
                n645 = property class="DigNum (strict)"(reference=w1708, error in=w1705) -> (error out=w1707:errorcluster, "Value"=w1706:dbl)  [unwired: 1 out]
                n646 = In Range and Coerce(upper limit=62.0, x=w1706, lower limit=58.0) -> (In Range?=w1702:bool)  [unwired: 1 out]
                n647 = Build Array(w1703, w1702) -> (w1704:bool[])
                n648 = Increment(x=w1718) -> (x+1=w1717:i32)
                n649 = call "PassOrFail (SubVI).vi"("index (row)"=w1717, "error in (no error)"=w1707, "Data in"=w1706, "Pass?Fail"=w1702, "Table in"=w1715) -> ("error out"=w1720:errorcluster)  [unwired: 6 in]
                n650 = And Array Elements(Boolean array=w1704) -> (logical AND=→"AuxiONResult":bool)
                n651 = Increment(x=w1717) -> (x+1=w1716:i32)
                n652 = Select(t="ON", s=w1703, f="OFF") -> (s? t:f=w1713:string)
                n653 = call "PassOrFail (SubVI).vi"("String Res"=w1713, "index (row)"=w1716, "error in (no error)"=w1720, "Data in"=-3.0, "Pass?Fail"=w1703, "Table in"=w1715) -> ("error out"=w1719:errorcluster)  [unwired: 5 in]
                n654 = call "TesterOption (SubVI).vi"("2 Options"=FALSE, "error in (no error)"=w1719, "On/Off"=FALSE, "Tester Option"=T11."Fan", "VISA Refnum in"=w1725) -> ("error out"=w1730:errorcluster)  [unwired: 5 in, 1 out]
                n655 = property class="Bool (strict)"(reference=w1731, error in=w1730) -> ("Value"=w1737:bool)  [unwired: 2 out]
                n656 = Select(t=enum16{"Stop", "CoolingON", "HotGunON", "Start"}."Stop", s=w1737, f=enum16{"Stop", "CoolingON", "HotGunON", "Start"}."CoolingON") -> (s? t:f=w1727:enum16{"Stop", "CoolingON", "HotGunON", "Start"})
              }
              frame "Start" {
                n657 = call "Write panel message (SubVI).vi"("Stop BurnIn"=w1795, 4:"rpm"=w1791, 5:"rpm"=FALSE ("rpm"), "PrintTime"=FALSE, "Stop"=w1782, "Time to wait"=0.1, "Strin"=w1790, "String in"=w1796) -> ("error out"=w1789:errorcluster)  [unwired: 3 in]
                n658 = call "TesterOption (SubVI).vi"("On/Off 2"=TRUE, "Tester Option 2"=T11."Fan", "2 Options"=TRUE, "error in (no error)"=w1789, "On/Off"=FALSE, "Tester Option"=T11."Venable", "VISA Refnum in"=w1783) -> ("error out"=w1781:errorcluster)  [unwired: 3 in, 1 out]
                n659 = call "Time Delay"("error in (no error)"=w1781) -> ("error out"=w1776:errorcluster)  [unwired: 10 in]
                n660 = property class="Bool (strict)"(reference=w1782, error in=w1776) -> ("Value"=w1797:bool)  [unwired: 2 out]
                n661 = Select(t=enum16{"Stop", "CoolingON", "HotGunON", "Start"}."Stop", s=w1797, f=enum16{"Stop", "CoolingON", "HotGunON", "Start"}."HotGunON") -> (s? t:f=w1778:enum16{"Stop", "CoolingON", "HotGunON", "Start"})
              }
            }
          }
        }
      }
    }
    n662 = flat-sequence {
      tunnel: w183 -> [_]
      frame #0 {
        w191 = T19."Enabled" ("Disabled")
        w192 = FALSE ("Start")
        n663 = property on="Start" class="Bool (strict)"("Value"=w192, "DisabledEnum"=w191) -> ()  [unwired: 2 in, 2 out]
        n664 = property on="Report" class="Bool (strict)"("Value"=w192, "DisabledEnum"=w191) -> ()  [unwired: 2 in, 2 out]
      }
    }
  }
  n665 = while {
    shift-right: [w1816] -> _
    shift-left: T10."Initialize" -> [w1815]
    shift-right: [w1812] -> _
    shift-left: _ -> [w1811]
    shift-right: [w1810] -> _
    shift-left: w20 -> [w1808]
    shift-right: [w1809] -> _
    shift-left: refnum<vi> refnum ("Config_CANAT") -> [w1807]
    shift-right: [w1805] -> _
    shift-left: w17 -> [w1806]
    tunnel: "ATR" -> [_]
    tunnel: w8 -> [w1804]
    tunnel: w7 -> [w1803]
    shift-right: [w1801] -> _
    shift-left: 0 -> [w1802]
    tunnel: w5 -> [w1800]
    tunnel: w3 -> [w1799]
    tunnel: w2 -> [_]
    tunnel: w18 -> [w1814]
    tunnel: [w1813] -> _
    stop <- w1798 stop-if-true
    n666 = case shown="\"Erase ATR Table\", Default" w1815 {
      tunnel: [T10."MainProgram" w1919 w1989 T10."Erase ATR Table"] -> w1816
      tunnel: [FALSE w1905 FALSE FALSE] -> w1798
      tunnel: [w1823 w1910 w1983 w2803] -> w1813
      tunnel: w1814 -> [_ w1930 w1987 _]
      tunnel: [w1860 refnum<visa-resource-name> refnum ("VISA resource name") w1984 w2808] -> w1812
      tunnel: w1811 -> [w1860 w1938 w1985 _]
      tunnel: [w1850 w1899 w1979 w2801] -> w1810
      tunnel: [w1849 refnum<vi> refnum ("Config_CANAT") w1980 w2804] -> w1809
      tunnel: w1808 -> [w1850 w1940 w1982 w2801]
      tunnel: w1807 -> [w1849 w1922 w1981 _]
      tunnel: w1806 -> [w1848 w1933 w1978 w2800]
      tunnel: [w1848 w1898 w1977 w2800] -> w1805
      tunnel: w1804 -> [_ _ w1976 _]
      tunnel: w1803 -> [_ _ w1975 _]
      tunnel: w1802 -> [w1837 w1924 w1974 w2797]
      tunnel: [w1837 w1924 w1973 w2797] -> w1801
      tunnel: w1800 -> [w1827 _ w1972 _]
      tunnel: w1799 -> [_ _ w1971 _]
      frame "Erase ATR Table", Default {
        w1831 = "Marvin" ("section")
        w1844 = refnum<visa-resource-name> "COM4" ("VISA resource name")
        w1855 = FALSE ("Visible")
        n667 = property on="Serial Com" class="Bool"(error in=errorcluster {"status"=FALSE, "code"=0, "source"=""} ("error out"), "Visible"=TRUE) -> (error out=w1845:errorcluster)  [unwired: 1 in, 1 out]
        n668 = property on="VISA Marvin" class="VISAName"(error in=w1845, "Visible"=w1855, "Value"=w1844) -> (error out=w1857:errorcluster)  [unwired: 1 in, 1 out]
        n669 = property on="VISA Marvin" class="VISAName"(error in=w1845, "Value"=w1844) -> ()  [unwired: 1 in, 2 out]
        n670 = property on="Status" class="Bool (strict)"(error in=w1857, "Value"=w1855) -> (error out=w1819:errorcluster)  [unwired: 1 in, 1 out]
        n671 = call "Select UUT"("error in (no error)"=w1819) -> ("EBAY"=w1817:bool, "error out"=w1818:errorcluster)  [unwired: 17 in]
        n672 = case shown="True" w1817 {
          tunnel: [string[][] [["1", "Communication Test", "", "", "", "", ""], ["1.1", "Serial RS-232", "N/A", "-", "", "", ""], ["1.2", "CAN Bus", "N/A", "-", "", "", ""], ["", "", "", "", "", "", ""], ["2", "Temperature Sensor Calibration", "", "", "", "", ""], ["2.1", "Sensor Reading Analog Offset", "0", "+/-0.100", ".", "", ""], ["", "", "", "", "", "", ""], ["3", "Motor Termistor Input Test", "", "", "", "", ""], ["3.1", "60 Degree", "60", "+/-3.00", "C", "", ""], ["3.2", "90 Degree", "90", "+/-3.00", "C", "", ""], ["3.3", "120 Degree", "120", "+/-3.00", "C", "", ""], ["", "", "", "", "", "", ""], ["4", "Enable Test", "", "", "", "", ""], ["4.1", "Fan Speed at Opened Enable ", "5000", "+/-200.0", "rpm", "", ""], ["4.2", "Fan Speed at Opened Enable ", "0", "+/-200.0", "rpm", "", ""], ["4.3", "Fan Speed at Closed Enable ", "5000", "+/-200.0", "rpm", "", ""], ["4.4", "Motor Rotation Direction", "Counter-clockwise (Inlet)", "-", "", "", ""], ["", "", "", "", "", "", ""], ["5", "Speed Command Test", "", "", "", "", ""], ["5.1", "Fan Speed", "6000", "+/-200.0", "rpm", "", ""], ["5.2", "Fan Speed", "9000", "+/-200.0", "rpm", "", ""], ["5.3", "Fan Speed", "12100", "+/-200.0", "rpm", "", ""], ["", "", "", "", "", "", ""], ["6", "Motor Stop time", "< 50", "-", "sec", "", ""], ["", "", "", "", "", "", ""], ["7", "Burn-in Test", "", "", "", "", ""], ["7.1", "DC Input Current", "28", "+/-5.000", "A", "", ""], ["7.2", "Fan Speed", "12100", "+/-200.0", "rpm", "", ""], ["7.3", "Ambient Temperature", "25", "+/-13.00", "C", "", ""], ["7.4", "After 10 min of operation", "", "-", "C", "", ""], ["7.5", "After 20 min of operation", "", "-", "C", "", ""], ["7.6", "After 30 min of operation", "", "-", "C", "", ""], ["", "", "", "", "", "", ""], ["8", "Visual Inspection", "", "", "", "", ""], ["8.1", "Verification of Components Not Installed", "N/A", "-", "", "", ""], ["8.2", "Manufacturing Defects", "N/A", "-", "", "", ""], ["", "", "", "", "", "", ""], ["9", "Power Supply Testing", "", "", "", "", ""], ["9.1", "Input Current Drawn", "", "", "", "", ""], ["9.2", "DC Input Current", "< 150", "-", "mA", "", ""], ["", "", "", "", "", "", ""], ["10", "Power Supply Voltages", "", "", "", "", ""], ["10.1", "12V", "12.0", "+/-0.500", "V", "", ""], ["10.2", "5V", "5.0", "+/-0.200", "V", "", ""], ["10.3", "3.3V", "3.3", "+/-0.100", "V", "", ""], ["10.4", "1.8V", "1.8", "+/-0.100", "V", "", ""], ["", "", "", "", "", "", ""], ["11", "Reverse Polarity Test - DC Input Current", "< 1", "-", "mA", "", ""], ["", "", "", "", "", "", ""], ["12", "Functional Test Procedure", "", "", "", "", ""], ["12.1", "Weight Check", "4180", "+/-10.00", "gr", "", ""], ["", "", "", "", "", "", ""], ["13", "Insulation Resistance Test", "", "", "", "", ""], ["13.1", "J3.B to Chassis", "> 1M", "-", "W", "", ""], ["13.2", "J1.16 to Chassis", "> 100K", "-", "W", "", ""], ["", "", "", "", "", "", ""], ["14", "Bonding Resistance", "", "", "", "", ""], ["14.1", "J1 Body to Chassis", "< 2m", "-", "W", "", ""], ["14.2", "J2  Body to Chassis", "< 2m", "-", "W", "", ""], ["14.3", "J3  Body to Chassis", "< 2m", "-", "W", "", ""], ["", "", "", "", "", "", ""], ["15", "CANbus Resistance Test", "", "", "", "", ""], ["15.1", "J1.17 to J1.18", "> 10K", "-", "W", "", ""], ["", "", "", "", "", "", ""], ["16", "Sealing Test", "N/A", "-", "", "", ""]] ("ArrAHU 2") string[][] [["1", "Communication Test", "", "", "", "", ""], ["1.1", "Serial RS-232", "N/A", "-", "", "", ""], ["1.2", "CAN Bus", "N/A", "-", "", "", ""], ["", "", "", "", "", "", ""], ["2", "Temperature Sensor Calibration", "", "", "", "", ""], ["2.1", "Sensor Reading Analog Offset", "0", "+/-0.100", ".", "", ""], ["", "", "", "", "", "", ""], ["3", "Motor Termistor Input Test", "", "", "", "", ""], ["3.1", "60 Degree", "60", "+/-3.00", "C", "", ""], ["3.2", "90 Degree", "90", "+/-3.00", "C", "", ""], ["3.3", "120 Degree", "120", "+/-3.00", "C", "", ""], ["", "", "", "", "", "", ""], ["4", "Enable Test", "", "", "", "", ""], ["4.1", "Fan Speed at Opened Enable ", "5000", "+/-200.0", "rpm", "", ""], ["4.2", "Fan Speed at Opened Enable ", "0", "+/-200.0", "rpm", "", ""], ["4.3", "Fan Speed at Closed Enable ", "5000", "+/-200.0", "rpm", "", ""], ["4.4", "Motor Rotation Direction", "Counter-clockwise (Inlet)", "-", "", "", ""], ["", "", "", "", "", "", ""], ["5", "Speed Command Test", "", "", "", "", ""], ["5.1", "Fan Speed", "6000", "+/-200.0", "rpm", "", ""], ["5.2", "Fan Speed", "11500", "+/-200.0", "rpm", "", ""], ["5.3", "Fan Speed", "15100", "+/-200.0", "rpm", "", ""], ["", "", "", "", "", "", ""], ["6", "Motor Stop time", "< 50", "-", "sec", "", ""], ["", "", "", "", "", "", ""], ["7", "Temperature Control Algorithm Test", "", "", "", "", ""], ["7.1", "Tair <   68 ± 2 oC", "6000", "+/-200.0", "rpm", "", ""], ["7.2", "Measured Temp.", "", "", "C", "", ""], ["7.3", "Tair >= 68 ± 2 oC", "11500", "+/-200.0", "rpm", "", ""], ["7.4", "Transition Temp.", "", "", "C", "", ""], ["7.5", "Tair >= 88 ± 2 oC", "15100", "+/-400.0", "rpm", "", ""], ["7.6", "Transition Temp.", "", "", "C", "", ""], ["7.7", "Tair <= 80 ± 2 oC", "11500", "+/-200.0", "rpm", "", ""], ["7.8", "Transition Temp.", "", "", "C", "", ""], ["7.9", "Tair <= 60 ± 2 oC", "6000", "+/-200.0", "rpm", "", ""], ["7.10", "Transition Temp.", "", "", "C", "", ""], ["", "", "", "", "", "", ""], ["8", "Burn-in Test", "", "", "", "", ""], ["8.1", "DC Input Current", "50", "+/-5.000", "A", "", ""], ["8.2", "Fan Speed", "15100", "+/-200.0", "rpm", "", ""], ["8.3", "Ambient Temperature", "25", "+/-13.00", "C", "", ""], ["8.4", "After 10 min of operation", "", "-", "C", "", ""], ["8.5", "After 20 min of operation", "", "-", "C", "", ""], ["8.6", "After 30 min of operation", "", "-", "C", "", ""], ["", "", "", "", "", "", ""], ["9", "Auxiliary Fan Test", "", "", "", "", ""], ["9.1", "Auxiliary Cooling Fan ON", "60", "+/-2.00", "C", "", ""], ["9.2", "Fan status", "ON", "-", "-", "", ""], ["9.3", "Auxiliary Cooling Fan OFF", "54", "+/-2.00", "C", "", ""], ["9.4", "Fan status", "OFF", "-", "-", "", ""], ["", "", "", "", "", "", ""], ["10", "Visual Inspection", "", "", "", "", ""], ["10.1", "Verification of Components Not Installed", "N/A", "-", "", "", ""], ["10.2", "Manufacturing Defects", "N/A", "-", "", "", ""], ["", "", "", "", "", "", ""], ["11", "Power Supply Testing", "", "", "", "", ""], ["11.1", "Input Current Drawn", "", "", "", "", ""], ["11.2", "DC Input Current", "< 150", "-", "mA", "", ""], ["", "", "", "", "", "", ""], ["12", "Power Supply Voltages", "", "", "", "", ""], ["12.1", "12V", "12.0", "+/-0.500", "V", "", ""], ["12.2", "5V", "5.0", "+/-0.200", "V", "", ""], ["12.3", "3.3V", "3.3", "+/-0.100", "V", "", ""], ["12.4", "1.8V", "1.8", "+/-0.100", "V", "", ""], ["", "", "", "", "", "", ""], ["13", "Reverse Polarity Test - DC Input Current", "< 1", "-", "mA", "", ""], ["", "", "", "", "", "", ""], ["14", "Functional Test Procedure", "", "", "", "", ""], ["14.1", "Weight Check", "4180", "+/-10.00", "gr", "", ""], ["", "", "", "", "", "", ""], ["15", "Insulation Resistance Test", "", "", "", "", ""], ["15.1", "J3.B to Chassis", "> 1M", "-", "W", "", ""], ["15.2", "J1.16 to Chassis", "> 100K", "-", "W", "", ""], ["", "", "", "", "", "", ""], ["16", "Bonding Resistance", "", "", "", "", ""], ["16.1", "J1 Body to Chassis", "< 2m", "-", "W", "", ""], ["16.2", "J2  Body to Chassis", "< 2m", "-", "W", "", ""], ["16.3", "J3  Body to Chassis", "< 2m", "-", "W", "", ""], ["", "", "", "", "", "", ""], ["17", "CANbus Resistance Test", "", "", "", "", ""], ["17.1", "J1.17 to J1.18", "> 10K", "-", "W", "", ""], ["", "", "", "", "", "", ""], ["18", "Sealing Test", "N/A", "-", "", "", ""]] ("ArrEbay 2")] -> w1853
          tunnel: ["AHU" "EBAY"] -> w1852
          tunnel: [w1870 w1882] -> w1851
          tunnel: w1818 -> [w1871 w1882]
          tunnel: [w1866 u8 95] -> w1824
          frame False {
            (unwired) string[][] [["6.1", "Visual Inspection", "", "", "", "", ""], ["6.1.1", "Verification of Components Not Installed", "N/A", "-", "", "", ""], ["", "", "", "", "", "", ""], ["6.1.2", "Manufacturing Defects", "N/A", "-", "", "", ""], ["", "", "", "", "", "", ""], ["6.2", "Power Supply Testing", "", "", "", "", ""], ["6.2.1", "Input Current Drawn", "", "", "", "", ""], ["6.2.1.1", "DC Input Current", "< 150", "-", "mA", "", ""], ["", "", "", "", "", "", ""], ["6.2.2", "Power Supply Voltages", "", "", "", "", ""], ["6.2.2.1", "12V", "12.0", "+/-0.500", "V", "", ""], ["6.2.2.2", "5V", "5.0", "+/-0.200", "V", "", ""], ["6.2.2.3", "3.3V", "3.3", "+/-0.100", "V", "", ""], ["6.2.2.4", "1.8V", "1.8", "+/-0.100", "V", "", ""], ["", "", "", "", "", "", ""], ["7", "Functional Test Procedure", "", "", "", "", ""], ["7.1", "Weight Check", "3800", "+/-100.0", "gr", "", ""], ["", "", "", "", "", "", ""], ["7.2", "Insulation Resistance Test", "", "", "", "", ""], ["7.2.1", "J3.B to Chassis", "> 1M", "-", "W", "", ""], ["7.2.2", "J1.16 to Chassis", "> 100K", "-", "W", "", ""], ["", "", "", "", "", "", ""], ["7.2", "Bonding Resistance", "", "", "", "", ""], ["7.2.3", "J1 Body to Chassis", "< 2m", "-", "W", "", ""], ["7.2.4", "J2  Body to Chassis", "< 2m", "-", "W", "", ""], ["7.2.5", "J3  Body to Chassis", "< 2m", "-", "W", "", ""], ["", "", "", "", "", "", ""], ["7.2.1", "CANbus Resistance Test", "", "", "", "", ""], ["7.2.1.1", "J1.17 to J1.18", "> 10K", "-", "W", "", ""], ["", "", "", "", "", "", ""], ["7.3", "Sealing Test", "N/A", "-", "", "", ""], ["", "", "", "", "", "", ""], ["7.4", "Communication Test", "", "", "", "", ""], ["7.4.1", "Serial RS-232", "N/A", "-", "", "", ""], ["7.4.2", "CAN Bus", "N/A", "-", "", "", ""], ["", "", "", "", "", "", ""], ["7.5", "Performances Tests", "", "", "", "", ""], ["7.5.1", "Reverse Polarity Test", "", "", "", "", ""], ["7.5.1.1", "DC Input Current", "< 1", "-", "mA", "", ""], ["", "", "", "", "", "", ""], ["7.5.2", "Enable Test", "", "", "", "", ""], ["7.5.2.1", "Fan Speed at Opened Enable ", "5000", "+/-200.0", "rpm", "", ""], ["7.5.2.2", "Fan Speed at Opened Enable ", "0", "+/-200.0", "rpm", "", ""], ["7.5.2.3", "Fan Speed at Closed Enable ", "5000", "+/-200.0", "rpm", "", ""], ["7.5.2.4", "Motor Rotation Direction", "Counter-clockwise (Inlet)", "-", "", "", ""], ["", "", "", "", "", "", ""], ["7.5.3", "Stop Time Test ", "", "", "", "", ""], ["7.5.3.1", "Motor Stop time", "< 50", "-", "sec", "", ""], ["", "", "", "", "", "", ""], ["7.5.4", "Speed Command Test", "", "", "", "", ""], ["7.5.4.1", "Fan Speed", "6000", "+/-200.0", "rpm", "", ""], ["7.5.4.2", "Fan Speed", "9000", "+/-200.0", "rpm", "", ""], ["7.5.4.3", "Fan Speed", "12100", "+/-200.0", "rpm", "", ""], ["", "", "", "", "", "", ""], ["7.5.5", "Temperature Sensor Calibration Test", "", "", "", "", ""], ["7.5.5.1", "Sensor Reading Analog Offset", "0", "+/-0.100", ".", "", ""], ["", "", "", "", "", "", ""], ["7.5.6", "Burn-in Test", "", "", "", "", ""], ["7.5.6.1", "DC Input Current", "28", "+/-3.000", "A", "", ""], ["7.5.6.2", "Fan Speed", "12100", "+/-200.000", "rpm", "", ""], ["7.5.6.3", "Ambient Temperature", "25", "+/-13.00", "C", "", ""], ["7.5.6.4", "After 10 min of operation", "", "", "C", "", ""], ["7.5.6.5", "After 20 min of operation", "", "", "C", "", ""], ["7.5.6.6", "After 30 min of operation", "", "", "C", "", ""], ["", "", "", "", "", "", ""], ["9", "Motor Temp Test", "", "", "", "", ""], ["9.1", "60 C", "60", "+/-3.000", "C", "", ""], ["9.2", "90 C", "90", "+/-3.000", "C", "", ""], ["9.3", "120 C", "120", "+/-3.000", "C", "", ""]] ("data")
            n673 = while {
              shift-right: [w1878] -> w1870
              shift-left: w1871 -> [w1879]
              tunnel: [w1873] -> w1869
              stop <- w1877 stop-if-true
              n674 = call "AHU UUT (subVI).vi"("error in (no error)"=w1879) -> ("AHU 47"=w1874:bool, "AHU 63"=w1873:bool, "OK"=w1876:bool, "error out"=w1878:errorcluster)  [unwired: 15 in]
              n675 = Exclusive Or(1:w1874, 2:w1873) -> (0:w1875:bool)
              n676 = And(x=w1876, y=w1875) -> (x .and. y?=w1877:bool)
            }
            n677 = Select(t=u8 63, s=w1869, f=u8 47) -> (s? t:f=w1866:u8)
          }
          frame True {
            (unwired) string[][] [["6.1", "Visual Inspection", "", "", "", "", ""], ["6.1.1", "Verification of Components Not Installed", "N/A", "-", "", "", ""], ["", "", "", "", "", "", ""], ["6.1.2", "Manufacturing Defects", "N/A", "-", "", "", ""], ["", "", "", "", "", "", ""], ["6.2", "Power Supply Testing", "", "", "", "", ""], ["6.2.1", "Input Current Drawn", "", "", "", "", ""], ["6.2.1.1", "DC Input Current", "< 150", "-", "mA", "", ""], ["", "", "", "", "", "", ""], ["6.2.2", "Power Supply Voltages", "", "", "", "", ""], ["6.2.2.1", "12V", "12.0", "+/-0.500", "V", "", ""], ["6.2.2.2", "5V", "5.0", "+/-0.200", "V", "", ""], ["6.2.2.3", "3.3V", "3.3", "+/-0.100", "V", "", ""], ["6.2.2.4", "1.8V", "1.8", "+/-0.100", "V", "", ""], ["", "", "", "", "", "", ""], ["7", "Functional Test Procedure", "", "", "", "", ""], ["7.1", "Weight Check", "4180", "+/-10.00", "gr", "", ""], ["", "", "", "", "", "", ""], ["7.2", "Insulation Resistance Test", "", "", "", "", ""], ["7.2.1", "J3.B to Chassis", "> 1M", "-", "W", "", ""], ["7.2.2", "J1.16 to Chassis", "> 100K", "-", "W", "", ""], ["", "", "", "", "", "", ""], ["7.2", "Bonding Resistance", "", "", "", "", ""], ["7.2.3", "J1 Body to Chassis", "< 2m", "-", "W", "", ""], ["7.2.4", "J2  Body to Chassis", "< 2m", "-", "W", "", ""], ["7.2.5", "J3  Body to Chassis", "< 2m", "-", "W", "", ""], ["", "", "", "", "", "", ""], ["7.2.1", "CANbus Resistance Test", "", "", "", "", ""], ["7.2.1.1", "J1.17 to J1.18", "> 10K", "-", "W", "", ""], ["", "", "", "", "", "", ""], ["7.3", "Sealing Test", "N/A", "-", "", "", ""], ["", "", "", "", "", "", ""], ["7.4", "Communication Test", "", "", "", "", ""], ["7.4.1", "Serial RS-232", "N/A", "-", "", "", ""], ["7.4.2", "CAN Bus", "N/A", "-", "", "", ""], ["", "", "", "", "", "", ""], ["7.5", "Performances Tests", "", "", "", "", ""], ["7.5.1", "Reverse Polarity Test", "", "", "", "", ""], ["7.5.1.1", "DC Input Current", "< 1", "-", "mA", "", ""], ["", "", "", "", "", "", ""], ["7.5.2", "Enable Test", "", "", "", "", ""], ["7.5.2.1", "Fan Speed at Opened Enable ", "5000", "+/-200.0", "rpm", "", ""], ["7.5.2.2", "Fan Speed at Opened Enable ", "0", "+/-200.0", "rpm", "", ""], ["7.5.2.3", "Fan Speed at Closed Enable ", "5000", "+/-200.0", "rpm", "", ""], ["7.5.2.4", "Motor Rotation Direction", "Counter-clockwise (Inlet)", "-", "", "", ""], ["", "", "", "", "", "", ""], ["7.5.3", "Stop Time Test ", "", "", "", "", ""], ["7.5.3.1", "Motor Stop time", "< 50", "-", "sec", "", ""], ["", "", "", "", "", "", ""], ["7.5.4", "Speed Command Test", "", "", "", "", ""], ["7.5.4.1", "Fan Speed", "6000", "+/-200.0", "rpm", "", ""], ["7.5.4.2", "Fan Speed", "11500", "+/-200.0", "rpm", "", ""], ["7.5.4.3", "Fan Speed", "15100", "+/-200.0", "rpm", "", ""], ["", "", "", "", "", "", ""], ["7.5.5", "Temperature Sensor Calibration Test", "", "", "", "", ""], ["7.5.5.1", "Sensor Reading Analog Offset", "0", "+/-0.100", ".", "", ""], ["", "", "", "", "", "", ""], ["7.5.6", "Temperature Control Algorithm Test", "", "", "", "", ""], ["7.5.6.1", "Tair <   68 ± 2 oC", "6000", "+/-200.0", "rpm", "", ""], ["7.5.6.2", "Measured Temp.", "", "", "C", "", ""], ["7.5.6.3", "Tair >= 68 ± 2 oC", "11500", "+/-200.0", "rpm", "", ""], ["7.5.6.4", "Transition Temp.", "", "", "C", "", ""], ["7.5.6.5", "Tair >= 88 ± 2 oC", "15100", "+/-400.0", "rpm", "", ""], ["7.5.6.6", "Transition Temp.", "", "", "C", "", ""], ["7.5.6.7", "Tair <= 80 ± 2 oC", "11500", "+/-200.0", "rpm", "", ""], ["7.5.6.8", "Transition Temp.", "", "", "C", "", ""], ["7.5.6.9", "Tair <= 60 ± 2 oC", "6000", "+/-200.0", "rpm", "", ""], ["7.5.6.10", "Transition Temp.", "", "", "C", "", ""], ["", "", "", "", "", "", ""], ["7.5.7", "Burn-in Test", "", "", "", "", ""], ["7.5.7.1", "DC Input Current", "50", "+/-5.000", "A", "", ""], ["7.5.7.2", "Fan Speed", "15100", "+/-200.0", "rpm", "", ""], ["7.5.7.3", "Ambient Temperature", "25", "+/-13.00", "C", "", ""], ["7.5.7.4", "After 10 min of operation", "", "-", "C", "", ""], ["7.5.7.5", "After 20 min of operation", "", "-", "C", "", ""], ["7.5.7.6", "After 30 min of operation", "", "-", "C", "", ""], ["", "", "", "", "", "", ""], ["8", "Auxiliary", "", "", "", "", ""], ["8.1", "Auxiliary Cooling Fan ON", "60", "+/-2.00", "C", "", ""], ["8.2", "Fan status", "ON", "-", "-", "", ""], ["8.3", "Auxiliary Cooling Fan OFF", "55", "+/-2.00", "C", "", ""], ["8.4", "Fan status", "OFF", "-", "-", "", ""], ["", "", "", "", "", "", ""], ["9", "Motor Temp. Test", "", "", "", "", ""], ["9.1", "60 Degree", "60", "+/-3.00", "C", "", ""], ["9.2", "90 Degree", "90", "+/-3.00", "C", "", ""], ["9.3", "120 Degree", "120", "+/-3.00", "C", "", ""]] ("data")
          }
        }
        "UUT" <- w1852
        "UUT" <- w1824
        n678 = for {
          tunnel: w1853 -> [w1888] mode=indexing
          tunnel: w1851 -> [w1886]
          tunnel: [w1885] -> w1847
          tunnel: w1853 -> [w1884]
          i -> [w1887]
          n679 = for {
            tunnel: w1888 -> [_] mode=indexing
            tunnel: w1887 -> [w1894]
            tunnel: w1886 -> [w1891]
            tunnel: [w1890] -> w1885
            tunnel: w1884 -> [w1889]
            i -> [w1895]
            n680 = Bundle By Name(cluster=T20 {"Row"=0, "Column"=0} ("Active Cell:Active Cell"), "Row"=w1894, "Column"=w1895) -> (w1893:T20)
            n681 = control-ref of="ATR"() -> (w1892:refnum<vi>)
            n682 = property class="Tbl (strict)"(reference=w1892, error in=w1891, "Active Cell"=w1893, "Cell BG Color"=u32 16777226, "Value"=w1889) -> (error out=w1890:errorcluster)  [unwired: 1 out]
          }
        }
        n683 = call "COM EvolutionBoard.vi"("error in (no error)"=w1847, "VISA resource name 2"=refnum<visa-resource-name> "COM1" ("VISA resource name")) -> ("error out"=w1843:errorcluster, "VISA resource name out"=w1842:refnum<visa-resource-name>)  [unwired: 8 in]
        n684 = call "TesterOption (SubVI).vi"("2 Options"=FALSE, "error in (no error)"=w1843, "On/Off"=FALSE, "Tester Option"=T11."Venable", "VISA Refnum in"=w1842) -> ("error out"=w1823:errorcluster, "VISA Refnum out"=→"VISA Tester":refnum<visa-resource-name>)  [unwired: 5 in]
        n685 = case shown="95" w1824 {
          tunnel: ["AHU Software Version" ("key") "EBAY Software Version" ("key")] -> w1833
          tunnel: ["AHU Serial Number" ("key") "EBAY Serial Number" ("key")] -> w1834
          frame 47, 63, Default {
          }
          frame 95 {
          }
        }
        n686 = call <vilib>:"Open Config Data.vi"("create file if necessary (T)"=FALSE, "configuration file path"=w1827) -> ("error out"=w1828:errorcluster, "refnum"=w1829:T25)  [unwired: 1 in, 7 out]
        n687 = call-poly <vilib>:"Read Key.vi"("section"=w1831, "error in (no error)"=w1828, "key"=w1833, "refnum"=w1829) -> ("error out"=w1835:errorcluster, "value"=→"UUT SoftwareVer":string, "refnum out"=w1832:T25)  [unwired: 2 in, 3 out]
        n688 = call-poly <vilib>:"Read Key.vi"("section"=w1831, "error in (no error)"=w1835, "key"=w1834, "refnum"=w1832) -> ("error out"=w1822:errorcluster, "value"=w1820:string, "refnum out"=w1821:T25)  [unwired: 2 in, 3 out]
        n689 = call <vilib>:"Close Config Data.vi"("error in (no error)"=w1822, "refnum"=w1821) -> ()  [unwired: 8 in, 2 out]
        n690 = Decimal String To Number(string=w1820) -> (number=w1825:i32)  [unwired: 2 in, 1 out]
        n691 = Increment(x=w1825) -> (x+1=→"Next SN":i32)
      }
      frame "Stop" {
        n692 = flat-sequence {
          tunnel: w1930 -> [w1968]
          tunnel: [w1967] -> w1923
          frame #0 {
            n693 = control-ref of="Pannel User Message"() -> (w1970:refnum<vi>)
            n694 = property class="Str"(reference=w1970, error in=w1968, "Value"="Program Stopped...\r\nPlease turn OFF All Power sinks") -> (error out=w1967:errorcluster)  [unwired: 1 out]
          }
        }
        n695 = control-ref of="VISA Tester"() -> (w1931:refnum<vi>)
        n696 = property class="VISAName"(reference=w1931, error in=w1923) -> ("Value"=w1929:refnum<visa-resource-name>)  [unwired: 2 out]
        n697 = disable-structure shown="Enabled" {
          disable-tunnel: w1923 -> [w1955 w1956]
          disable-tunnel: w1922 -> [w1953 _]
          disable-tunnel: [w1952 w1956] -> w1909
          frame Disabled {
            n698 = call "Clear CAN Buffer.vi"("error in (no error)"=w1955, "Cluster in"=w1953) -> ("error out"=w1954:errorcluster)  [unwired: 8 in, 1 out]
            n699 = call "Close CAN Device.vi"("error in (no error)"=w1954, "Cluster in"=w1953) -> ("error out"=w1952:errorcluster)  [unwired: 8 in, 1 out]
          }
          frame Enabled {
          }
        }
        n700 = VISA Close(VISA resource name=w1938, error in (no error)=w1923) -> (error out=w1932:errorcluster)
        n701 = property on="Stop Button" class="Bool (strict)"() -> ("Value"=w1901:bool)  [unwired: 2 in, 2 out]
        n702 = call "TesterOption (SubVI).vi"("2 Options"=FALSE, "On/Off"=FALSE, "Tester Option"=T11."Power", "VISA Refnum in"=w1929) -> ("error out"=w1918:errorcluster, "VISA Refnum out"=w1928:refnum<visa-resource-name>)  [unwired: 6 in]
        n703 = property on="ClosePanel" class="Bool (strict)"() -> ("Value"=w1902:bool)  [unwired: 2 in, 2 out]
        n704 = VISA Close(VISA resource name=w1928, error in (no error)=w1918) -> (error out=w1915:errorcluster)
        n705 = Or(x=w1902, y=w1901) -> (x .or. y?=w1900:bool)
        n706 = Flush Queue(queue=w1933, error in (no error)=w1932) -> (queue out=w1935:refnum<queue>, error out=w1934:errorcluster)  [unwired: 1 out]
        n707 = Flush Queue(queue=w1940, error in (no error)=w1932) -> (queue out=w1939:refnum<queue>, error out=w1941:errorcluster)  [unwired: 1 out]
        n708 = case shown="False" w1900 {
          tunnel: w1941 -> [w1943 w1951]
          tunnel: w1939 -> [w1945 w1947]
          tunnel: w1935 -> [w1944 w1946]
          tunnel: w1934 -> [w1942 w1950]
          tunnel: [w1943 w1949] -> w1917
          tunnel: [w1942 w1948] -> w1916
          tunnel: [w1945 w1947] -> w1899
          tunnel: [w1944 w1946] -> w1898
          frame False {
          }
          frame True {
            n709 = Release Queue(queue=w1946, error in (no error)=w1950) -> (error out=w1948:errorcluster)  [unwired: 1 in, 2 out]
            n710 = Release Queue(queue=w1947, error in (no error)=w1951) -> (error out=w1949:errorcluster)  [unwired: 1 in, 2 out]
          }
        }
        n711 = Merge Errors(w1917, w1916, w1915, w1909) -> (w1914:errorcluster)
        n712 = property on="Refresh Button" class="Bool (strict)"() -> ("Value"=w1903:bool)  [unwired: 2 in, 2 out]
        n713 = call <vilib>:"Clear Errors.vi"("error in (no error)"=w1914) -> ("error out"=w1913:errorcluster)  [unwired: 5 in, 1 out]
        n714 = property on="Stop Button" class="Bool (strict)"() -> ("Value"=w1907:bool)  [unwired: 2 in, 2 out]
        n715 = property on="ClosePanel" class="Bool (strict)"(error in=w1913) -> (error out=w1911:errorcluster, "Value"=w1912:bool)  [unwired: 1 in, 1 out]
        n716 = Not(x=w1903) -> (.not. x?=w1904:bool)
        n717 = Select(t=T10."Initialize", s=w1903, f=T10."Stop") -> (s? t:f=w1919:T10)
        n718 = Not(x=w1907) -> (.not. x?=w1906:bool)
        n719 = Compound Arithmetic op=AND(w1912, w1906, w1904) -> (w1908:bool)
        n720 = case shown="False" w1908 {
          tunnel: w1911 -> [w1959 w1963]
          tunnel: [w1959 w1963] -> w1910
          tunnel: [w1958 w1962] -> w1905
          tunnel: w1903 -> [w1957 _]
          frame False {
            n721 = case shown="False" w1957 {
              tunnel: [TRUE FALSE] -> w1958
              frame False {
              }
              frame True {
              }
            }
          }
          frame True {
            n722 = flat-sequence {
              tunnel: [TRUE] -> w1962
              frame #0 {
              }
              frame #1 {
                n723 = control-ref of="This VI"() -> (w1966:refnum<vi>)
                n724 = property class="VI"(reference=w1966, "FP.State"=T21."Closed" ("Front Panel Window:State")) -> ()  [unwired: 1 in, 2 out]
              }
            }
          }
        }
      }
      frame "MainProgram" {
        n725 = event shown="[1] \"SetSN\": Value Change" {
          selector: w1976 -> [_ _ _ _ _ _ _ _ _ _ _ _ _]
          dyn-events: _ -> [_ _ _ _ _ _ _ _ _ _ _ _ _]
          timeout: 120 -> [_ _ _ _ _ _ _ _ _ _ _ _ _]
          tunnel: [T10."MainProgram" T10."MainProgram" T10."MainProgram" T10."MainProgram" T10."MainProgram" T10."Stop" T10."MainProgram" w2540 T10."MainProgram" T10."MainProgram" T10."MainProgram" T10."Stop" T10."MainProgram"] -> w1989
          tunnel: [w1991 w2072 w2135 w2142 w2151 w2169 w2194 w2599 w2662 w2675 w2685 w2766 w2772] -> w1983
          tunnel: w1987 -> [w2004 w2072 w2134 w2144 w2151 w2169 w2201 w2599 w2663 w2674 w2681 w2766 w2777]
          tunnel: [w2012 w2066 w2136 w2143 w2152 w2167 w2190 w2548 w2660 w2672 w2686 w2764 w2770] -> w1984
          tunnel: w1985 -> [w2012 w2066 w2136 w2143 w2152 w2167 w2190 w2548 w2660 w2672 _ w2764 w2770]
          tunnel: w1982 -> [w2006 w2078 w2130 w2139 w2148 w2166 w2199 w2579 w2659 w2671 w2689 w2763 w2775]
          tunnel: w1981 -> [w2001 w2077 w2131 w2140 w2149 w2165 w2172 w2578 w2658 w2670 w2688 w2762 w2768]
          tunnel: [w2003 w2077 w2131 w2140 w2149 w2165 w2172 w2578 w2658 w2670 w2688 w2762 w2768] -> w1980
          tunnel: [w2005 w2078 w2130 w2139 w2148 w2166 w2199 w2579 w2659 w2671 w2689 w2763 w2775] -> w1979
          tunnel: w1978 -> [w1999 w2076 w2129 w2138 w2147 w2164 w2198 w2577 w2657 w2669 w2687 w2761 w2774]
          tunnel: [w1999 w2076 w2129 w2138 w2147 w2164 w2193 w2577 w2657 w2669 w2687 w2761 w2774] -> w1977
          tunnel: w1975 -> [_ _ _ _ _ _ _ w2546 _ _ _ _ _]
          tunnel: w1974 -> [w2000 w2075 w2128 w2137 w2146 w2162 w2188 w2552 w2656 w2668 w2683 w2760 w2773]
          tunnel: [w2000 w2075 w2128 w2137 w2146 w2162 w2188 w2551 w2656 w2668 w2683 w2760 w2773] -> w1973
          tunnel: w1972 -> [_ w2073 _ _ _ _ _ w2550 _ _ _ _ _]
          tunnel: w1971 -> [_ w2065 _ _ _ _ _ _ _ _ _ _ _]
          event Timeout {
            n726 = event-data() -> ()  [unwired: 1 in, 3 out]
            n727 = property class="Clust (strict)"(reference=w2001, error in=w2004) -> (reference out=w2003:refnum<vi>, error out=w2002:errorcluster, "Value"=w2009:T7)
            n728 = Unbundle By Name(w2009) -> ("DevType"=w2010:T2, "CanIndex"=w2008:T1)
            n729 = property on="ClosePanel" class="Bool (strict)"("Value"=FALSE ("ClosePanel")) -> ()  [unwired: 2 in, 2 out]
            n730 = call "VCI_Receive.vi"("CANIndex"=w2008, "DevIndex"=u32 0, "DevType"=w2010) -> ("Recieve"=w2007:T26[])  [unwired: 3 in, 5 out]
            n731 = Empty Array?(array=w2007) -> (empty?=w1994:bool)
            n732 = case shown="False" w1994 {
              tunnel: w2008 -> [w2026 _]
              tunnel: w2003 -> [w2024 _]
              tunnel: w2006 -> [w2023 w2059]
              tunnel: w2002 -> [w2022 w2058]
              tunnel: w2007 -> [w2027 _]
              tunnel: [w2017 w2058] -> w1991
              tunnel: [w2016 w2059] -> w2005
              tunnel: [TRUE FALSE] -> w1990
              frame False {
                n733 = call "Demo_MakeDispBuff.vi"("Channel"=w2026, "Type"=enum16{"接收", "发送"}."接收", "OBJs"=w2027) -> ("Buffer"=w2025:T27)
                n734 = for {
                  N: 3 -> [_]
                  tunnel: w2025 -> [w2041]
                  tunnel: w2024 -> [w2040]
                  tunnel: w2023 -> [w2031]
                  tunnel: w2022 -> [w2030]
                  tunnel: [w2033] -> w2020 mode=indexing
                  tunnel: [w2031] -> w2019
                  tunnel: [w2030] -> w2018
                  i -> [w2029]
                  n735 = property class="Clust (strict)"(reference=w2040) -> ("Value"=w2038:T7)  [unwired: 1 in, 2 out]
                  n736 = Index Array(array=w2041, index=w2029) -> (element=w2034:T28)
                  n737 = Unbundle By Name(w2034) -> ("Channel"=w2036:T1, "VCI_CAN_OBJ"=w2039:T26)  [unwired: 2 out]
                  n738 = Unbundle By Name(w2038) -> ("CanIndex"=w2037:T1)
                  n739 = Equal?(x=w2037, y=w2036) -> (x = y?=w2035:bool)
                  n740 = case shown="True" w2035 {
                    tunnel: w2039 -> [_ w2052]
                    tunnel: [w2042 w2048] -> w2033
                    tunnel: T22 {"ID"=0, "MSGTYPE"=0, "LEN"=0, "aDATA"=[]} ("Msg") -> [w2042 w2047]
                    frame False {
                    }
                    frame True {
                      n741 = Unbundle By Name(w2052) -> ("ID"=w2046:u32, "DataLen"=w2051:u8, "Data"=w2049:u8[])
                      n742 = Bundle By Name(cluster=w2047, "ID"=w2046, "MSGTYPE"=u8 0, "LEN"=w2051, "aDATA"=w2049) -> (w2048:T22)
                      n743 = Unbundle By Name(w2048) -> ("ID"=w2044:u32)
                      n744 = Split Number(x=w2044) -> (lo(x)=w2045:u16)  [unwired: 1 out]
                      n745 = Split Number(x=w2045) -> (lo(x)=w2043:u8)  [unwired: 1 out]
                      n746 = case shown="63" w2043 {
                        tunnel: ["EBAY 5F" "" "AHU 3F" "AHU 2F"] -> _
                        frame 95 {
                        }
                        frame Default {
                        }
                        frame 63 {
                        }
                        frame 47 {
                        }
                      }
                    }
                  }
                }
                n747 = Enqueue Element(queue=w2019, element=w2020, error in (no error)=w2018) -> (queue out=w2016:refnum<queue>, error out=w2017:errorcluster)  [unwired: 2 out]
              }
              frame True {
              }
            }
            n748 = control-ref of="ATR"() -> (w1993:refnum<vi>)
            n749 = property on="CAN Status" class="Bool (strict)"("Value"=w1990) -> ()  [unwired: 2 in, 2 out]
            n750 = call "PassFailUUT (SubVI).vi"("error in (no error)"=w1991, "Table in"=w1993) -> ("PassFaileUUTresult"=w1992:bool)  [unwired: 8 in, 1 out]
            n751 = property on="Test Failed" class="Bool (strict)"("Value"=w1992) -> ()  [unwired: 2 in, 2 out]
            n752 = property on="Automation" class="Bool (strict)"() -> ("Value"=w1996:bool)  [unwired: 2 in, 2 out]
            n753 = property on="Start" class="Bool (strict)"() -> ("Value"=w1998:bool)  [unwired: 2 in, 2 out]
            n754 = Or(x=w1996, y=w1998) -> (x .or. y?=w1997:bool)
            n755 = case shown="False" w1997 {
              frame False {
                n756 = property on="Pannel User Message" class="Str"("Value"="You can press start to execute(s) test(s).") -> ()  [unwired: 2 in, 2 out]
              }
              frame True {
              }
            }
          }
          event "SetSN": Value Change {
            n757 = event-data() -> ()  [unwired: 1 in, 6 out]
            n758 = property on="Current SN" class="DigNum (strict)"(error in=w2072) -> ("Value"=w2071:i32)  [unwired: 1 in, 2 out]
            n759 = Equal To 0?(x=w2071) -> (x = 0?=w2068:bool)
            n760 = Equal?(x=w2071, y=-1) -> (x = y?=w2069:bool)
            n761 = Or(x=w2069, y=w2068) -> (x .or. y?=w2067:bool)
            n762 = property on="Status" class="Bool (strict)"() -> ("Value"=w2063:bool)  [unwired: 2 in, 2 out]
            n763 = case shown="True" w2063 {
              tunnel: w2073 -> [_ w2090]
              tunnel: w2067 -> [_ w2089]
              tunnel: w2066 -> [_ w2087]
              tunnel: w2065 -> [_ w2085]
              tunnel: [errorcluster {"status"=FALSE, "code"=0, "source"=""} ("error out") w2084] -> w2062
              tunnel: [w2079 w2083] -> w2064
              frame False {
                w2079 = FALSE ("Value")
                n764 = property on="SetSN" class="Bool (strict)"("Value"=w2079) -> ()  [unwired: 2 in, 2 out]
                n765 = call "Display Message to User10"() -> ()  [unwired: 10 in, 2 out]
              }
              frame True {
                n766 = property on="Test Failed" class="Bool (strict)"() -> ("Value"=w2081:bool)  [unwired: 2 in, 2 out]
                n767 = property on="Automation" class="Bool (strict)"() -> ("Value"=w2083:bool)  [unwired: 2 in, 2 out]
                n768 = Not(x=w2081) -> (.not. x?=w2082:bool)
                n769 = Select(t=w2082, s=w2083, f=w2085) -> (s? t:f=w2088:bool)
                n770 = And(x=w2089, y=w2088) -> (x .and. y?=w2086:bool)
                n771 = case shown="False" w2086 {
                  tunnel: w2090 -> [_ w2120]
                  tunnel: w2087 -> [_ w2113]
                  tunnel: [w2092 w2105] -> w2084
                  tunnel: w2081 -> [w2091 _]
                  frame False {
                    n772 = case shown="False" w2091 {
                      tunnel: [w2094 w2095] -> w2092
                      frame False {
                        n773 = call "Display Message to User9"() -> ("error out"=w2094:errorcluster)  [unwired: 10 in, 1 out]
                      }
                      frame True {
                        n774 = call "Display Message to User3"() -> ("error out"=w2095:errorcluster)  [unwired: 10 in, 1 out]
                      }
                    }
                    n775 = property on="Automation" class="Bool (strict)"(error in=w2092, "Value"=FALSE ("Automation")) -> ()  [unwired: 1 in, 2 out]
                  }
                  frame True {
                    w2112 = FALSE ("SetSN")
                    n776 = property on="Next SN" class="DigNum (strict)"() -> ("Value"=w2096:i32)  [unwired: 2 in, 2 out]
                    n777 = property on="VISA Tester" class="VISAName"() -> ("Value"=w2103:refnum<visa-resource-name>)  [unwired: 2 in, 2 out]
                    n778 = call "TesterOption (SubVI).vi"("2 Options"=FALSE, "On/Off"=FALSE, "Tester Option"=T11."Venable", "VISA Refnum in"=w2103) -> ("error out"=w2098:errorcluster)  [unwired: 6 in, 1 out]
                    n779 = call <vilib>:"Clear Errors.vi"("error in (no error)"=w2098) -> ("error out"=w2099:errorcluster)  [unwired: 5 in, 1 out]
                    n780 = Number To Decimal String(number=w2096) -> (decimal integer string=w2097:string)  [unwired: 1 in]
                    "UUT SN Report" <- w2097
                    n781 = Search and Replace String(input string="EP=1\r\nSN=0\r\n" ("write buffer"), search string="0", replace string=w2097) -> (result string=w2115:string)  [unwired: 5 in, 3 out]
                    n782 = call "SerialMarvinSendGet.vi"("error in (no error)"=w2099, "Clear Log"=FALSE, "write buffer"=w2115, "VISA resource name"=w2113) -> ("error out"=w2104:errorcluster)  [unwired: 6 in, 1 out]
                    n783 = property on="UUT" class="DigNum (strict)"(error in=w2104) -> ("Value"=w2121:u8)  [unwired: 1 in, 2 out]
                    n784 = case shown="47, 63, Default" w2121 {
                      tunnel: ["AHU Serial Number" ("key") "EBAY Serial Number" ("key")] -> w2124
                      frame 47, 63, Default {
                      }
                      frame 95 {
                      }
                    }
                    n785 = call <vilib>:"Open Config Data.vi"("create file if necessary (T)"=FALSE, "configuration file path"=w2120) -> ("error out"=w2118:errorcluster, "refnum"=w2119:T25)  [unwired: 1 in, 7 out]
                    n786 = call-poly <vilib>:"Write Key.vi"("section"="Marvin", "error in (no error)"=w2118, "value"=w2097, "key"=w2124, "refnum"=w2119) -> ("error out"=w2108:errorcluster, "refnum out"=w2107:T25)  [unwired: 4 in, 1 out]
                    n787 = call <vilib>:"Close Config Data.vi"("error in (no error)"=w2108, "refnum"=w2107) -> ("error out"=w2106:errorcluster)  [unwired: 8 in, 1 out]
                    n788 = property on="Current SN" class="DigNum (strict)"("Value"=w2096) -> ()  [unwired: 2 in, 2 out]
                    n789 = property on="SetSN" class="Bool (strict)"(error in=w2106, "Value"=w2112) -> (error out=w2111:errorcluster)  [unwired: 1 in, 1 out]
                    n790 = property on="Automation" class="Bool (strict)"(error in=w2111, "Value"=w2112) -> (error out=w2110:errorcluster)  [unwired: 1 in, 1 out]
                    n791 = Increment(x=w2096) -> (x+1=w2109:i32)
                    n792 = property on="Next SN" class="DigNum (strict)"(error in=w2110, "Value"=w2109) -> (error out=w2105:errorcluster)  [unwired: 1 in, 1 out]
                  }
                }
              }
            }
            n793 = property on="SetSN" class="Bool (strict)"(error in=w2062, "Value"=FALSE ("SetSN")) -> (error out=w2061:errorcluster)  [unwired: 1 in, 1 out]
            n794 = case shown="True" w2064 {
              tunnel: w2061 -> [_ _]
              frame False {
              }
              frame True {
                w2127 = TRUE ("Value (Signaling)")
                n795 = property on="Report" class="Bool (strict)"("Val(Sgnl)"=w2127, "Value"=w2127) -> ()  [unwired: 2 in, 2 out]
              }
            }
          }
          event "ATR": Mouse Enter {
            n796 = event-data() -> ()  [unwired: 1 in, 4 out]
            n797 = call-poly <vilib>:"Set Cursor.vi"("error in (no error)"=w2134, "icon"=u16 1) -> ("error out"=w2135:errorcluster)  [unwired: 8 in, 1 out]
          }
          event "ATR": Mouse Leave {
            n798 = event-data() -> ()  [unwired: 1 in, 4 out]
            n799 = call-poly <vilib>:"Set Cursor.vi"("error in (no error)"=w2144, "icon"=u16 0) -> ("error out"=w2142:errorcluster)  [unwired: 8 in, 1 out]
          }
          event "ATR": Mouse Down? {
            n800 = event-data() -> ("Coords"=w2159:T29)  [unwired: 1 in, 4 out]
            n801 = invoke on="ATR" class="Tbl (strict)" method="Point To Row Column"("Point"=w2159) -> ("InBounds"=w2155:bool, "CellPosition"=w2154:T20)  [unwired: 5 in, 4 out]
            n802 = Greater Than 0?(x=w2154) -> (x > 0?=w2158:cluster{"Row":bool, "Column":bool})
            n803 = Cluster To Array(cluster=w2158) -> (array=w2157:bool[])
            n804 = Or Array Elements(Boolean array=w2157) -> (logical OR=w2156:bool)
            n805 = Or(x=w2155, y=w2156) -> (x .or. y?=w2153:bool)
            n806 = event-data("Discard?"=w2153) -> ()  [unwired: 1 in, 1 out]
          }
          event Panel Close? {
            n807 = event-data() -> ("VIRef"=w2163:refnum<vi>)  [unwired: 1 in, 3 out]
            n808 = Close Reference(reference=w2163) -> ()  [unwired: 1 in, 1 out]
            n809 = disable-structure shown="Disabled" {
              frame Disabled {
                n810 = property on="Stop Button" class="Bool (strict)"("Val(Sgnl)"=TRUE ("Stop Button"), "Value"=FALSE ("Stop Button")) -> ()  [unwired: 2 in, 2 out]
              }
              frame Enabled {
              }
            }
            n811 = event-data("Discard?"=TRUE) -> ()  [unwired: 1 in, 1 out]
            "ClosePanel" <- TRUE ("ClosePanel")
          }
          event "Start": Value Change {
            w2189 = T16 [] items=["Auxiliary", "Temp Sens Cal", "Com Test", "Enable Test", "Speed Command", "Stop Time", "Temp Control", "Burn in", "Visual Inspec", "Empty"]
            n812 = event-data() -> ()  [unwired: 1 in, 2 out]
            n813 = property on="VISA Tester" class="VISAName"() -> ("Value"=w2187:refnum<visa-resource-name>)  [unwired: 2 in, 2 out]
            n814 = property on="UUT" class="Str"(error in=w2201) -> (error out=w2183:errorcluster, "Value"=w2200:string)  [unwired: 1 in, 1 out]
            n815 = control-ref of="Pannel User Message"() -> (w2180:refnum<vi>)
            n816 = control-ref of="Motor Speed RPM"() -> (w2175:refnum<vi>)
            n817 = call "TesterOption (SubVI).vi"("2 Options"=FALSE, "error in (no error)"=w2183, "On/Off"=FALSE, "Tester Option"=T11."Venable", "VISA Refnum in"=w2187) -> ("error out"=w2182:errorcluster)  [unwired: 5 in, 1 out]
            n818 = control-ref of="Stop Burn-in"() -> (w2178:refnum<vi>)
            n819 = control-ref of="Stop Button"() -> (w2179:refnum<vi>)
            n820 = call "Write panel message (SubVI).vi"("Stop BurnIn"=w2178, 4:"rpm"=w2175, 5:"rpm"=FALSE ("rpm"), "PrintTime"=TRUE, "Stop"=w2179, "error in (no error)"=w2182, "Time to wait"=5.0, "Strin"="TESTER BIT TEST OPERATION IN PROCESS", "String in"=w2180) -> ("error out"=w2181:errorcluster)  [unwired: 2 in]
            n821 = while {
              tunnel: w2200 -> [w2229]
              tunnel: [w2228] -> w2196
              tunnel: [w2227] -> w2195
              shift-right: [w2224] -> _
              shift-left: enum16{"Stop", "Tests", "Bit test", "Start"}."Start" -> [w2226]
              tunnel: w2190 -> [w2225]
              tunnel: w2189 -> [w2223]
              tunnel: w2181 -> [w2208]
              tunnel: w2179 -> [w2217]
              tunnel: w2178 -> [w2216]
              tunnel: w2180 -> [w2215]
              tunnel: w2175 -> [w2214]
              tunnel: w2172 -> [w2207]
              stop <- w2222 stop-if-true
              n822 = property class="Clust (strict)"(reference=w2207, error in=w2208) -> ("Value"=w2210:T7)  [unwired: 2 out]
              n823 = Unbundle By Name(w2210) -> ("DevType"=w2212:T2, "CanIndex"=w2211:T1)
              n824 = property on="VISA Tester" class="VISAName"() -> ("Value"=w2220:refnum<visa-resource-name>)  [unwired: 2 in, 2 out]
              n825 = call "VCI_Receive.vi"("CANIndex"=w2211, "DevIndex"=u32 0, "DevType"=w2212) -> ("Recieve"=w2213:T26[])  [unwired: 3 in, 5 out]
              n826 = Empty Array?(array=w2213) -> (empty?=w2206:bool)
              n827 = Not(x=w2206) -> (.not. x?=w2205:bool)
              n828 = property on="CAN Status" class="Bool (strict)"("Value"=w2205) -> (error out=w2204:errorcluster)  [unwired: 2 in, 1 out]
              n829 = property on="CAN Status" class="Bool (strict)"(error in=w2204) -> (error out=w2203:errorcluster, "Value"=w2218:bool)  [unwired: 1 in, 1 out]
              n830 = property on="Status" class="Bool (strict)"(error in=w2203) -> (error out=w2219:errorcluster, "Value"=w2221:bool)  [unwired: 1 in, 1 out]
              n831 = case shown="\"Tests\"" w2226 {
                tunnel: w2229 -> [_ w2244 w2354 _]
                tunnel: [w2234 w2243 w2389 w2495] -> w2228
                tunnel: [w2230 w2242 w2352 w2487] -> w2227
                tunnel: w2225 -> [_ _ w2370 w2500]
                tunnel: w2215 -> [_ _ _ w2499]
                tunnel: w2217 -> [_ _ _ w2498]
                tunnel: w2216 -> [_ _ _ w2497]
                tunnel: w2214 -> [_ _ _ w2496]
                tunnel: [w2233 w2241 w2357 w2491] -> w2224
                tunnel: w2223 -> [w2234 _ w2389 w2495]
                tunnel: [w2232 w2240 FALSE FALSE] -> w2222
                tunnel: w2221 -> [_ _ _ w2493]
                tunnel: w2220 -> [_ _ w2371 _]
                tunnel: w2219 -> [w2230 _ _ _]
                tunnel: w2218 -> [_ _ _ w2488]
                frame "Stop", Default {
                  n832 = property on="Start" class="Bool (strict)"(error in=w2230, "Value"=FALSE ("Start")) -> ()  [unwired: 1 in, 2 out]
                  n833 = flat-sequence {
                    tunnel: [enum16{"Stop", "Tests", "Bit test", "Start"}."Stop"] -> w2233
                    tunnel: w2230 -> [_]
                    tunnel: [TRUE] -> w2232
                    frame #0 {
                    }
                  }
                }
                frame "Tests" {
                  w2237 = FALSE ("Stop Burn-in")
                  w2239 = T19."Disabled and Grayed Out" ("Disabled")
                  n834 = case shown="\"AHU\", Default" w2244 {
                    tunnel: [w2259 w2308] -> w2243
                    tunnel: [w2258 w2307] -> w2242
                    tunnel: [w2247 w2295] -> w2238
                    frame "AHU", Default {
                      n835 = call "Load Program Process AHU.vi"() -> ("Speed Command Test"=w2252:bool, "Enable Test"=w2253:bool, "Burn-in Test"=w2250:bool, "Auxiliary"=w2248:bool, "Temperature Sensor Calibration Test"=w2255:bool, "Communication Test"=w2254:bool, "Stop Time Test"=w2251:bool, "Visual Inspection"=w2249:bool, "OK"=w2256:bool, "Automation"=w2247:bool, "error out"=w2258:errorcluster)  [unwired: 8 in, 9 out]
                      n836 = Or(x=w2256, y=w2247) -> (x .or. y?=w2257:bool)
                      n837 = case shown="True" w2257 {
                        tunnel: [w2260 w2270] -> w2259
                        tunnel: w2247 -> [_ w2269]
                        tunnel: w2255 -> [_ w2268]
                        tunnel: w2254 -> [_ w2267]
                        tunnel: w2253 -> [_ w2266]
                        tunnel: w2252 -> [_ w2265]
                        tunnel: w2251 -> [_ w2264]
                        tunnel: w2250 -> [_ w2263]
                        tunnel: w2249 -> [_ w2262]
                        tunnel: w2248 -> [_ w2261]
                        frame False {
                          w2260 = T16 [] items=["Auxiliary", "Temp Sens Cal", "Com Test", "Enable Test", "Speed Command", "Stop Time", "Temp Control", "Burn in", "Visual Inspec", "Empty"]
                        }
                        frame True {
                          n838 = case shown="False" w2269 {
                            tunnel: [w2293 w2294] -> w2270
                            tunnel: w2268 -> [w2275 _]
                            tunnel: w2267 -> [w2274 _]
                            tunnel: w2266 -> [w2276 _]
                            tunnel: w2265 -> [w2273 _]
                            tunnel: w2264 -> [w2272 _]
                            tunnel: w2263 -> [w2286 _]
                            tunnel: w2262 -> [w2271 _]
                            tunnel: w2261 -> [_ _]
                            frame False {
                              w2279 = T23."Empty" ("f")
                              n839 = Select(t=T23."Com Test" ("f"), s=w2274, f=w2279) -> (s? t:f=w2285:T23)
                              n840 = Select(t=T23."Temp Sens Cal" ("f"), s=w2275, f=w2279) -> (s? t:f=w2284:T23)
                              n841 = Select(t=T23."Stop Time" ("f"), s=w2272, f=w2279) -> (s? t:f=w2283:T23)
                              n842 = Select(t=T23."Enable Test" ("f"), s=w2276, f=w2279) -> (s? t:f=w2282:T23)
                              n843 = Select(t=T23."Speed Command" ("f"), s=w2273, f=w2279) -> (s? t:f=w2281:T23)
                              n844 = Select(t=T23."Burn in" ("f"), s=w2286, f=w2279) -> (s? t:f=w2280:T23)
                              n845 = Select(t=T23."Visual Inspec" ("f"), s=w2271, f=w2279) -> (s? t:f=w2277:T23)
                              n846 = Build Array(w2285, w2284, w2283, w2282, w2281, w2280, w2277) -> (w2293:T16)
                            }
                            frame True {
                              w2294 = T16 [enum."Com Test", enum."Temp Sens Cal", enum."Stop Time", enum."Enable Test", enum."Speed Command", enum."Burn in", enum."Visual Inspec"] items=["Auxiliary", "Temp Sens Cal", "Com Test", "Enable Test", "Speed Command", "Stop Time", "Temp Control", "Burn in", "Visual Inspec", "Empty"]
                            }
                          }
                        }
                      }
                    }
                    frame "EBAY" {
                      n847 = call "Load Program Process EBAY.vi"() -> ("Speed Command Test"=w2301:bool, "Enable Test"=w2302:bool, "Burn-in Test"=w2299:bool, "Temperature Control Algorithm Test"=w2298:bool, "Auxiliary"=w2296:bool, "Temperature Sensor Calibration Test"=w2304:bool, "Communication Test"=w2303:bool, "Stop Time Test"=w2300:bool, "Visual Inspection"=w2297:bool, "OK"=w2305:bool, "Automation"=w2295:bool, "error out"=w2307:errorcluster)  [unwired: 8 in, 8 out]
                      n848 = Or(x=w2305, y=w2295) -> (x .or. y?=w2306:bool)
                      n849 = case shown="True" w2306 {
                        tunnel: [w2309 w2320] -> w2308
                        tunnel: w2295 -> [_ w2319]
                        tunnel: w2304 -> [_ w2318]
                        tunnel: w2303 -> [_ w2317]
                        tunnel: w2302 -> [_ w2316]
                        tunnel: w2301 -> [_ w2315]
                        tunnel: w2300 -> [_ w2314]
                        tunnel: w2299 -> [_ w2313]
                        tunnel: w2298 -> [_ w2312]
                        tunnel: w2297 -> [_ w2311]
                        tunnel: w2296 -> [_ w2310]
                        frame False {
                          w2309 = T16 [] items=["Auxiliary", "Temp Sens Cal", "Com Test", "Enable Test", "Speed Command", "Stop Time", "Temp Control", "Burn in", "Visual Inspec", "Empty"]
                        }
                        frame True {
                          n850 = case shown="False" w2319 {
                            tunnel: [w2349 w2350] -> w2320
                            tunnel: w2318 -> [w2325 _]
                            tunnel: w2317 -> [w2324 _]
                            tunnel: w2316 -> [w2323 _]
                            tunnel: w2315 -> [w2322 _]
                            tunnel: w2314 -> [w2321 _]
                            tunnel: w2313 -> [w2327 _]
                            tunnel: w2312 -> [w2326 _]
                            tunnel: w2311 -> [w2340 _]
                            tunnel: w2310 -> [w2331 _]
                            frame False {
                              w2329 = T23."Empty" ("f")
                              n851 = Select(t=T23."Com Test" ("f"), s=w2324, f=w2329) -> (s? t:f=w2339:T23)
                              n852 = Select(t=T23."Temp Sens Cal" ("f"), s=w2325, f=w2329) -> (s? t:f=w2338:T23)
                              n853 = Select(t=T23."Stop Time" ("f"), s=w2321, f=w2329) -> (s? t:f=w2337:T23)
                              n854 = Select(t=T23."Enable Test" ("f"), s=w2323, f=w2329) -> (s? t:f=w2336:T23)
                              n855 = Select(t=T23."Speed Command" ("f"), s=w2322, f=w2329) -> (s? t:f=w2335:T23)
                              n856 = Select(t=T23."Temp Control" ("f"), s=w2326, f=w2329) -> (s? t:f=w2334:T23)
                              n857 = Select(t=T23."Burn in" ("f"), s=w2327, f=w2329) -> (s? t:f=w2333:T23)
                              n858 = Select(t=T23."Visual Inspec" ("f"), s=w2340, f=w2329) -> (s? t:f=w2332:T23)
                              n859 = Select(t=T23."Auxiliary" ("f"), s=w2331, f=w2329) -> (s? t:f=w2328:T23)
                              n860 = Build Array(w2339, w2338, w2337, w2336, w2335, w2334, w2333, w2328, w2332) -> (w2349:T16)
                            }
                            frame True {
                              w2350 = T16 [enum."Com Test", enum."Temp Sens Cal", enum."Stop Time", enum."Enable Test", enum."Speed Command", enum."Temp Control", enum."Burn in", enum."Auxiliary", enum."Visual Inspec"] items=["Auxiliary", "Temp Sens Cal", "Com Test", "Enable Test", "Speed Command", "Stop Time", "Temp Control", "Burn in", "Visual Inspec", "Empty"]
                            }
                          }
                        }
                      }
                    }
                  }
                  "Automation" <- w2238
                  n861 = flat-sequence {
                    tunnel: [enum16{"Stop", "Tests", "Bit test", "Start"}."Tests"] -> w2241
                    tunnel: [TRUE] -> w2240
                    frame #0 {
                    }
                  }
                  n862 = property on="Stop Button" class="Bool (strict)"("Value"=w2237) -> ()  [unwired: 2 in, 2 out]
                  n863 = property on="Stop Burn-in" class="Bool (strict)"("Value"=w2237) -> ()  [unwired: 2 in, 2 out]
                  n864 = property on="Start" class="Bool (strict)"("DisabledEnum"=w2239) -> ()  [unwired: 2 in, 2 out]
                  n865 = property on="Report" class="Bool (strict)"("DisabledEnum"=w2239) -> ()  [unwired: 2 in, 2 out]
                }
                frame "Bit test" {
                  # "Stop"
                  n866 = call "SerialMarvinSendGet.vi"("write buffer"="TA[1]\r\n", "VISA resource name"=w2370) -> ("error out"=w2383:errorcluster, "read buffer"=w2386:string)  [unwired: 8 in]
                  n867 = Fract/Exp String To Number(string=w2386) -> (number=w2385:dbl)  [unwired: 3 in, 1 out]
                  n868 = Less Or Equal?(x=w2385, y=100.0) -> (x <= y?=w2368:bool)
                  n869 = call "TesterOption (SubVI).vi"("On/Off 2"=FALSE, "Tester Option 2"=T11."Venable", "2 Options"=TRUE, "error in (no error)"=w2383, "On/Off"=TRUE, "Tester Option"=T11."25C", "VISA Refnum in"=w2371) -> ("error out"=w2373:errorcluster)  [unwired: 3 in, 1 out]
                  n870 = call "Time Delay5"("error in (no error)"=w2373) -> ("error out"=w2372:errorcluster)  [unwired: 10 in]
                  n871 = call "SerialMarvinSendGet.vi"("error in (no error)"=w2372, "write buffer"="TA[2]\r\n", "VISA resource name"=w2370) -> ("error out"=w2369:errorcluster, "read buffer"=w2375:string)  [unwired: 7 in]
                  n872 = case shown="Default" w2354 {
                    tunnel: w2371 -> [w2419 _ w2447]
                    tunnel: w2370 -> [_ _ w2450]
                    tunnel: w2369 -> [w2420 w2438 w2449]
                    tunnel: [w2413 w2438 w2445] -> w2356
                    tunnel: [w2410 "" w2440] -> w2363
                    tunnel: [w2409 bool[] [] w2439] -> w2361
                    frame "AHU" {
                      n873 = call "TesterOption (SubVI).vi"("On/Off 2"=FALSE, "Tester Option 2"=T11."Venable", "2 Options"=TRUE, "error in (no error)"=w2420, "On/Off"=TRUE, "Tester Option"=T11."K17", "VISA Refnum in"=w2419) -> ("error out"=w2422:errorcluster)  [unwired: 3 in, 1 out]
                      n874 = call "Time Delay7"("error in (no error)"=w2422) -> ("error out"=w2421:errorcluster)  [unwired: 10 in]
                      n875 = call "GetADCTester (SubVI).vi"("error in (no error)"=w2421, "GetADCTester"=T13."Current", "TimeToGet"=5, "VISA Refnum in"=w2419) -> ("error out"=w2413:errorcluster, "ADCValOutput Single"=w2415:dbl)  [unwired: 5 in, 1 out]
                      n876 = Less Or Equal?(x=w2415, y=50.0) -> (x <= y?=w2414:bool)
                      n877 = Build Array(w2414) -> (w2409:bool[])
                      n878 = for {
                        tunnel: w2409 -> [w2435] mode=indexing
                        tunnel: string[] ["CURRENT OPERATION FAILED!"] -> [w2431] mode=indexing
                        shift-right: [w2433] -> w2410
                        shift-left: "" -> [w2432]
                        n879 = Concatenate Strings(w2431, "  TEST FAILED!" ("string"), "\r\n") -> (w2428:string)
                        n880 = Select(t=w2428, s=w2435, f=w2432) -> (s? t:f=w2434:string)
                        n881 = Concatenate Strings(w2432, w2434) -> (w2433:string)
                      }
                    }
                    frame Default {
                    }
                    frame "EBAY" {
                      w2448 = T30 [enum."Fan", enum."Current"] items=["Term1", "Term2", "Current", "Fan", "TempCPU"]
                      n882 = call "TesterOption (SubVI).vi"("On/Off 2"=FALSE, "Tester Option 2"=T11."Venable", "2 Options"=TRUE, "error in (no error)"=w2449, "On/Off"=TRUE, "Tester Option"=T11."K17", "VISA Refnum in"=w2447) -> ("error out"=w2452:errorcluster)  [unwired: 3 in, 1 out]
                      n883 = call "Time Delay6"("error in (no error)"=w2452) -> ("error out"=w2451:errorcluster)  [unwired: 10 in]
                      n884 = call "SerialMarvinSendGet.vi"("error in (no error)"=w2451, "write buffer"="TA[3]\r\n", "VISA resource name"=w2450) -> ("error out"=w2446:errorcluster, "read buffer"=w2454:string)  [unwired: 7 in]
                      n885 = Fract/Exp String To Number(string=w2454) -> (number=w2455:dbl)  [unwired: 3 in, 1 out]
                      n886 = for {
                        tunnel: w2448 -> [w2479] mode=indexing
                        tunnel: w2447 -> [w2478]
                        tunnel: w2446 -> [w2476]
                        tunnel: [w2475] -> w2445
                        tunnel: [w2472] -> w2443 mode=indexing
                        i -> [w2473]
                        n887 = call "GetADCTester (SubVI).vi"("error in (no error)"=w2476, "GetADCTester"=w2479, "TimeToGet"=0, "VISA Refnum in"=w2478) -> ("error out"=w2475:errorcluster, "ADCValOutput Single"=w2474:dbl)  [unwired: 5 in, 1 out]
                        n888 = case shown="1" w2473 {
                          tunnel: w2474 -> [w2482 w2485 _]
                          tunnel: [w2480 w2483 FALSE] -> w2472
                          frame 1 {
                            n889 = Less Or Equal?(x=w2482, y=50.0) -> (x <= y?=w2480:bool)
                          }
                          frame 0 {
                            n890 = Greater Or Equal?(x=w2485, y=2200.0) -> (x >= y?=w2483:bool)
                          }
                          frame Default {
                          }
                        }
                      }
                      n891 = Less Or Equal?(x=w2455, y=100.0) -> (x <= y?=w2444:bool)
                      n892 = Build Array (concatenate)(w2444, w2443) -> (w2439:bool[])
                      n893 = for {
                        tunnel: w2439 -> [w2462] mode=indexing
                        tunnel: string[] ["TA[3] OPERATION FAILED!", "EBAY FAN OPERATION FAILED!", "CURRENT OPERATION FAILED!"] -> [w2465] mode=indexing
                        shift-right: [w2467] -> w2440
                        shift-left: "" -> [w2466]
                        n894 = Concatenate Strings(w2465, "\r\n") -> (w2463:string)
                        n895 = case shown="False" w2462 {
                          tunnel: [w2470 w2471] -> w2467
                          tunnel: w2466 -> [w2469 w2471]
                          tunnel: w2463 -> [w2468 _]
                          frame False {
                            n896 = Concatenate Strings(w2469, w2468) -> (w2470:string)
                          }
                          frame True {
                          }
                        }
                      }
                    }
                  }
                  n897 = Fract/Exp String To Number(string=w2375) -> (number=w2376:dbl)  [unwired: 3 in, 1 out]
                  n898 = Less Or Equal?(x=w2376, y=100.0) -> (x <= y?=w2367:bool)
                  n899 = Build Array(w2368, w2367) -> (w2362:bool[])
                  n900 = for {
                    tunnel: w2362 -> [w2398] mode=indexing
                    tunnel: string[] ["TA[1] OPERATION FAILED!", "TA[2] OPERATION FAILED!"] -> [w2402] mode=indexing
                    shift-right: [w2404] -> w2364
                    shift-left: "" -> [w2403]
                    tunnel: w2356 -> [w2399]
                    tunnel: [w2399] -> w2355
                    n901 = Concatenate Strings(w2402, "\r\n") -> (w2400:string)
                    n902 = case shown="False" w2398 {
                      tunnel: [w2407 w2408] -> w2404
                      tunnel: w2403 -> [w2406 w2408]
                      tunnel: w2400 -> [w2405 _]
                      frame False {
                        n903 = Concatenate Strings(w2406, w2405) -> (w2407:string)
                      }
                      frame True {
                      }
                    }
                  }
                  n904 = Build Array (concatenate)(w2362, w2361) -> (w2360:bool[])
                  n905 = And Array Elements(Boolean array=w2360) -> (logical AND=w2351:bool)
                  n906 = case shown="False" w2351 {
                    tunnel: w2364 -> [w2396 _]
                    tunnel: w2363 -> [w2395 _]
                    tunnel: w2355 -> [w2393 w2397]
                    tunnel: [w2393 w2397] -> w2353
                    frame False {
                      n907 = Concatenate Strings(w2396, w2395) -> (w2394:string)
                      n908 = One Button Dialog(message=w2394) -> ()  [unwired: 1 in, 1 out]
                    }
                    frame True {
                    }
                  }
                  n909 = case shown="False" w2351 {
                    tunnel: w2353 -> [w2391 w2392]
                    tunnel: [w2390 w2392] -> w2352
                    frame False {
                      n910 = call "Display Message to User6"("error in (no error)"=w2391) -> ("error out"=w2390:errorcluster)  [unwired: 9 in, 1 out]
                    }
                    frame True {
                    }
                  }
                  n911 = Select(t=enum16{"Stop", "Tests", "Bit test", "Start"}."Tests", s=w2351, f=enum16{"Stop", "Tests", "Bit test", "Start"}."Stop") -> (s? t:f=w2357:enum16{"Stop", "Tests", "Bit test", "Start"})
                }
                frame "Start" {
                  n912 = And(x=w2488, y=w2493) -> (x .and. y?=w2489:bool)
                  n913 = case shown="True" w2489 {
                    tunnel: w2500 -> [_ w2527]
                    tunnel: w2499 -> [_ w2518]
                    tunnel: w2498 -> [_ w2514]
                    tunnel: w2497 -> [_ w2512]
                    tunnel: w2496 -> [_ w2511]
                    tunnel: [FALSE w2510] -> w2492
                    tunnel: [w2506 w2509] -> w2487
                    tunnel: [FALSE TRUE] -> w2490
                    frame False {
                      n914 = call "Display Message to User5"() -> ("error out"=w2506:errorcluster)  [unwired: 10 in, 1 out]
                    }
                    frame True {
                      n915 = property on="VISA Tester" class="VISAName"() -> (error out=w2525:errorcluster, "Value"=w2524:refnum<visa-resource-name>)  [unwired: 2 in, 1 out]
                      n916 = call "TesterOption (SubVI).vi"("2 Options"=FALSE, "error in (no error)"=w2525, "On/Off"=FALSE, "Tester Option"=T11."Venable", "VISA Refnum in"=w2524) -> ("error out"=w2520:errorcluster)  [unwired: 5 in, 1 out]
                      n917 = call "Write panel message (SubVI).vi"("Stop BurnIn"=w2512, 4:"rpm"=w2511, 5:"rpm"=FALSE ("rpm"), "PrintTime"=FALSE, "Stop"=w2514, "error in (no error)"=w2520, "Time to wait"=3.0, "Strin"="TESTER BIT TEST OPERATION IN PROCESS\nPlease wait...", "String in"=w2518) -> ("error out"=w2519:errorcluster)  [unwired: 2 in]
                      n918 = property on="UUT SoftwareVer" class="Str"() -> ("Value"=w2508:string)  [unwired: 2 in, 2 out]
                      n919 = call "SerialMarvinSendGet.vi"("error in (no error)"=w2519, "write buffer"="VR\r\n", "VISA resource name"=w2527) -> ("error out"=w2509:errorcluster, "read buffer"=w2526:string)  [unwired: 7 in]
                      n920 = Equal?(x=w2526, y=w2508) -> (x = y?=w2510:bool)
                    }
                  }
                  n921 = case shown="False" w2492 {
                    tunnel: [enum16{"Stop", "Tests", "Bit test", "Start"}."Stop" enum16{"Stop", "Tests", "Bit test", "Start"}."Bit test"] -> w2491
                    tunnel: w2490 -> [w2501 _]
                    frame False {
                      n922 = case shown="True" w2501 {
                        frame False {
                        }
                        frame True {
                          n923 = call "Display Message to User4"() -> ()  [unwired: 10 in, 2 out]
                        }
                      }
                    }
                    frame True {
                    }
                  }
                }
              }
            }
            n924 = Bundle By Name(cluster=T8 {"VISA"="COM1", "Array Test"=[]}, "VISA"=w2190, "Array Test"=w2196) -> (w2192:T8)
            n925 = Enqueue Element(queue=w2198, element=w2192, error in (no error)=w2195) -> (queue out=w2193:refnum<queue>, error out=w2194:errorcluster)  [unwired: 2 out]
          }
          event "Report", "Stop Button": Value Change {
            w2558 = "Marvin" ("section")
            n926 = event-data() -> ("CtlRef"=w2544:refnum<vi>)  [unwired: 1 in]
            n927 = local read "UUT"() -> (w2554:string)
            n928 = call <vilib>:"Application Directory.vi"() -> ("Application Directory"=w2586:path)
            n929 = Build Path(base path=w2586, name or relative path="Reports") -> (appended path=w2589:path)
            n930 = property on="Status" class="Bool (strict)"() -> ("Value"=w2529:bool)  [unwired: 2 in, 2 out]
            n931 = case shown="\"EBAY\", Default" w2554 {
              tunnel: ["REV EBAY" ("key") "REV AHU" ("key")] -> w2556
              frame "EBAY", Default {
              }
              frame "AHU" {
              }
            }
            n932 = call <vilib>:"Check if File or Folder Exists.vi"("path"=w2589) -> ("error out"=w2587:errorcluster, "file or folder exists?"=w2590:bool, "dup path"=w2588:path)  [unwired: 8 in]
            n933 = case shown="False" w2590 {
              tunnel: w2587 -> [w2653 w2654]
              tunnel: w2588 -> [w2652 w2655]
              tunnel: [w2651 w2655] -> w2595
              tunnel: [w2650 w2654] -> w2592
              frame False {
                n934 = Create Folder(path (use dialog)=w2652, error in=w2653) -> (created path=w2651:path, error out=w2650:errorcluster)  [unwired: 1 in, 1 out]
              }
              frame True {
              }
            }
            n935 = case shown="True" w2529 {
              tunnel: [w2602 w2618] -> w2575
              tunnel: [w2602 w2617] -> w2553
              tunnel: w2548 -> [_ w2612]
              tunnel: [w2602 w2608] -> w2545
              tunnel: [w2602 w2606] -> w2547
              tunnel: [w2602 w2613] -> w2538
              tunnel: [w2602 w2611] -> w2530
              frame False {
                (unwired) "47"
                (unwired) " 413-8005_47_AHU"
                (unwired) "413-8005-1-47"
                (unwired) "5.3.9" ("read buffer")
                (unwired) "95"
                (unwired) "414-8005_95_EBAY_"
                (unwired) "414-8005-95"
                (unwired) "414-8005-95   "
                w2602 = "N_A" ("read buffer")
                n936 = disable-structure shown="Disabled" {
                  frame Disabled {
                    n937 = call "Display Message to User7"() -> ()  [unwired: 10 in, 2 out]
                  }
                  frame Enabled {
                  }
                }
                n938 = Decimal String To Number(string="1" ("Value")) -> (number=w2603:i32)  [unwired: 2 in, 1 out]
                n939 = Number To Decimal String(number=w2603, width (-)=i16 4) -> ()  [unwired: 1 out]
              }
              frame True {
                n940 = property on="UUT SN Report" class="Str"() -> ("Value"=w2607:string)  [unwired: 2 in, 2 out]
                n941 = Decimal String To Number(string=w2607) -> (number=w2609:i32)  [unwired: 2 in, 1 out]
                n942 = Number To Decimal String(number=w2609, width (-)=i16 4) -> (decimal integer string=w2608:string)
                n943 = call "SerialMarvinSendGet.vi"("write buffer"="VR\r\n", "VISA resource name"=w2612) -> ("error out"=w2614:errorcluster, "read buffer"=w2606:string)  [unwired: 8 in]
                n944 = property on="UUT" class="DigNum (strict)"(error in=w2614) -> ("Value"=w2616:u8)  [unwired: 1 in, 2 out]
                n945 = case shown="95, Default" w2616 {
                  tunnel: ["414-8005_95_EBAY_" " 413-8005_47_AHU" " 413-8005_63_AHU"] -> w2618
                  tunnel: ["414-8005-95   " w2624 w2627] -> w2617
                  tunnel: ["414-8005-95" w2624 w2627] -> w2613
                  tunnel: ["95" "47" "63"] -> w2611
                  frame 95, Default {
                  }
                  frame 47 {
                    w2624 = "413-8005-1-47"
                    (unwired) "AHU-L (47) 413-8005-1"
                  }
                  frame 63 {
                    w2627 = "413-8005-2-63"
                    (unwired) "AHU-R (63) 413-8005-2"
                  }
                }
              }
            }
            n946 = Get Date/Time String(want seconds? (F)=TRUE) -> (date string=w2591:string)  [unwired: 2 in, 1 out]
            n947 = call <vilib>:"Open Config Data.vi"("create file if necessary (T)"=FALSE, "configuration file path"=w2550) -> ("refnum"=w2565:T25)  [unwired: 1 in, 8 out]
            n948 = property on="Logger Path" class="Path"(error in=w2592, "Value"=w2595, "StartPath"=w2595) -> (error out=w2593:errorcluster)  [unwired: 1 in, 1 out]
            n949 = Search and Replace String(replace all?=TRUE ("replace all? (F)"), input string=w2591, search string="/") -> (result string=w2572:string)  [unwired: 5 in, 3 out]
            n950 = call-poly <vilib>:"Read Key.vi"("section"=w2558, "key"=w2556, "refnum"=w2565) -> ("error out"=w2560:errorcluster, "value"=w2563:string, "refnum out"=w2562:T25)  [unwired: 5 in, 1 out]
            n951 = property on="Logger Path" class="Path"(error in=w2593) -> (error out=w2568:errorcluster, "StartPath"=w2571:path)  [unwired: 1 in, 1 out]
            n952 = call-poly <vilib>:"Read Key.vi"("section"=w2558, "error in (no error)"=w2560, "key"="Tester Software Ver", "refnum"=w2562) -> ("error out"=w2557:errorcluster, "value"=w2555:string, "refnum out"=w2561:T25)  [unwired: 4 in, 1 out]
            n953 = Concatenate Strings("ATR" ("string"), w2575, w2545, "_", w2572, ".docx" ("string")) -> (w2569:string)
            n954 = call <vilib>:"Close Config Data.vi"("error in (no error)"=w2557, "refnum"=w2561) -> ()  [unwired: 8 in, 2 out]
            n955 = Build Path(base path=w2571, name or relative path=w2569) -> (appended path=w2570:path)
            n956 = call "HeaderuRayon.vi"("Oper."=w2546, "VR"=w2547, "S/N"=w2545, "UUT"=w2553, "UA"=w2530, "UUTHeader"=w2554, "Tester Software Ver"=w2555) -> ("HEADER1"=w2596:string)  [unwired: 1 in]
            n957 = Concatenate Strings("  Rev-" ("string"), w2563) -> (w2549:string)
            n958 = while {
              tunnel: w2569 -> [w2635]
              tunnel: w2571 -> [w2632]
              shift-right: [w2634] -> w2567
              shift-left: w2570 -> [w2633]
              shift-right: [w2630] -> w2551
              shift-left: w2552 -> [w2631]
              tunnel: w2568 -> [w2636]
              tunnel: [w2637] -> _
              stop <- w2629 continue-if-true
              n959 = call <vilib>:"Check if File or Folder Exists.vi"("error in (no error)"=w2636, "path"=w2633) -> ("error out"=w2637:errorcluster, "file or folder exists?"=w2629:bool)  [unwired: 7 in, 1 out]
              n960 = case shown="True" w2629 {
                tunnel: w2635 -> [_ w2649]
                tunnel: w2631 -> [_ w2641]
                tunnel: [w2639 w2646] -> w2634
                tunnel: w2633 -> [w2639 _]
                tunnel: w2632 -> [_ w2647]
                tunnel: [1 w2640] -> w2630
                frame False {
                }
                frame True {
                  w2642 = ".docx" ("search string")
                  n961 = Search and Replace String(input string=w2649, search string=w2642) -> (result string=w2648:string)  [unwired: 6 in, 3 out]
                  n962 = Number To Decimal String(number=w2641) -> (decimal integer string=w2644:string)  [unwired: 1 in]
                  n963 = call <vilib>:"Space Constant.vi"() -> ("String"=w2643:string)
                  n964 = Concatenate Strings(w2648, w2643, w2644, w2642) -> (w2645:string)
                  n965 = Build Path(base path=w2647, name or relative path=w2645) -> (appended path=w2646:path)
                  n966 = Increment(x=w2641) -> (x+1=w2640:i32)
                }
              }
            }
            n967 = Open/Create/Replace File(file path (use dialog)=w2567, operation (0:open)=T24."create") -> (error out=w2581:errorcluster)  [unwired: 4 in, 2 out]
            n968 = control-ref of="ATR"() -> (w2597:refnum<vi>)
            n969 = property class="Tbl (strict)"(reference=w2597, error in=w2581) -> ("Value"=w2598:string[][])  [unwired: 2 out]
            n970 = call "MarvinReport.vi"("HEADER1"=w2596, "ATR Or"=w2597, "Steps   pfull"=w2598, "Footer UUT"=w2538, "pageNum"=3, "FILE NAME"=w2569, "Report Folder"=w2567, "REV"=w2549, "Test-Conductor"=w2546) -> ("error out"=w2533:errorcluster)  [unwired: 5 in, 1 out]
            n971 = call <vilib>:"Clear Errors.vi"("error in (no error)"=w2533) -> ("error out"=w2532:errorcluster)  [unwired: 5 in, 1 out]
            n972 = property class="Bool (strict)"(reference=w2544, error in=w2532) -> ("BoolText.Text"=w2543:string)  [unwired: 2 out]
            n973 = Equal?(x=w2543, y="Report") -> (x = y?=w2537:bool)
            n974 = Select(t=T10."MainProgram", s=w2537, f=T10."Stop") -> (s? t:f=w2540:T10)
            n975 = Select(t="Save Report...", s=w2537, f="Program Stopped...\r\nPlease turn OFF All Power sinks") -> (s? t:f=w2535:string)
            n976 = property on="Report" class="Bool (strict)"(error in=w2532, "Value"=FALSE ("Report")) -> ()  [unwired: 1 in, 2 out]
            n977 = property on="Pannel User Message" class="Str"("Value"=w2535) -> ()  [unwired: 2 in, 2 out]
          }
          event "Help Button": Value Change {
            n978 = event-data() -> ()  [unwired: 1 in, 6 out]
            n979 = vi-ref "Help.vi"() -> (w2665:refnum<vi>)
            n980 = invoke class="VI" method="FP.Open"(reference=w2665, error in=w2663, "Activate"=TRUE ("Activate?"), "State"=T21."Standard") -> (error out=w2664:errorcluster)  [unwired: 1 in, 4 out]
            n981 = call "Help.vi"("error in"=w2664) -> ("error out"=w2662:errorcluster)  [unwired: 7 in]
          }
          event "Serial Com": Value Change {
            n982 = event-data() -> ()  [unwired: 1 in, 6 out]
            n983 = property on="Serial Com" class="Bool"(error in=w2674, "Visible"=FALSE) -> (error out=w2678:errorcluster)  [unwired: 1 in, 1 out]
            n984 = property on="VISA Marvin" class="VISAName"(error in=w2678, "Visible"=TRUE) -> (error out=w2675:errorcluster)  [unwired: 1 in, 1 out]
          }
          event "VISA Marvin": Value Change {
            n985 = event-data() -> ()  [unwired: 1 in, 6 out]
            n986 = property on="Serial Com" class="Bool"(error in=w2681, "Visible"=FALSE) -> (error out=w2680:errorcluster)  [unwired: 1 in, 1 out]
            n987 = control-ref of="This VI"() -> (w2692:refnum<vi>)
            n988 = property on="Pannel User Message" class="Str"(error in=w2681, "Value"="Serial connection in process" ("Pannel User Message")) -> ()  [unwired: 1 in, 2 out]
            n989 = call "Serial InitMarvin.vi"("error in (no error)"=w2680, "VI reference (current VI)"=w2692, "VISA Refnum in"="VISA Marvin") -> ("error out"=w2684:errorcluster, "Boolean"=w2682:bool)  [unwired: 7 in]
            n990 = property on="VISA Marvin" class="VISAName"(error in=w2684, "Visible"=FALSE) -> (error out=w2695:errorcluster)  [unwired: 1 in, 1 out]
            n991 = property on="Serial Com" class="Bool"(error in=w2695, "Visible"=TRUE) -> (error out=w2691:errorcluster)  [unwired: 1 in, 1 out]
            n992 = case shown="True" w2682 {
              tunnel: w2691 -> [w2698 w2710]
              tunnel: "VISA Marvin" -> [w2699 w2707]
              tunnel: [w2699 w2706] -> w2686
              tunnel: [w2698 w2705] -> w2685
              frame False {
              }
              frame True {
                n993 = call "SerialMarvinSendGet.vi"("error in (no error)"=w2710, "Clear Log"=FALSE, "write buffer"="VC\r\n", "VISA resource name"=w2707) -> ("error out"=w2709:errorcluster, "read buffer"=w2703:string)  [unwired: 6 in]
                n994 = Decimal String To Number(string=w2703) -> (number=w2702:i32)  [unwired: 2 in, 1 out]
                n995 = Less Or Equal?(x=w2702, y=50) -> (x <= y?=w2700:bool)
                n996 = property on="Status" class="Bool (strict)"("Value"=w2700) -> ()  [unwired: 2 in, 2 out]
                n997 = case shown="True" w2700 {
                  tunnel: w2709 -> [w2711 w2735]
                  tunnel: w2707 -> [w2712 w2734]
                  tunnel: [w2712 w2725] -> w2706
                  tunnel: [w2711 w2719] -> w2705
                  frame False {
                  }
                  frame True {
                    n998 = call <vilib>:"Clear Errors.vi"("error in (no error)"=w2735) -> ("error out"=w2736:errorcluster)  [unwired: 5 in, 1 out]
                    n999 = control-ref of="ATR"() -> (w2722:refnum<vi>)
                    n1000 = VISA Flush I/O Buffer(VISA resource name=w2734, error in (no error)=w2736) -> (VISA resource name out=w2725:refnum<visa-resource-name>, error out=w2733:errorcluster)  [unwired: 1 in]
                    n1001 = call "Display Message to User2"("error in (no error)"=w2733) -> ("error out"=w2732:errorcluster, "Yes"=w2731:bool)  [unwired: 9 in]
                    n1002 = case shown="True" w2731 {
                      tunnel: w2732 -> [w2737 w2759]
                      tunnel: [w2737 w2738] -> w2730
                      tunnel: w2725 -> [_ w2756]
                      frame False {
                      }
                      frame True {
                        w2744 = FALSE ("2 Options")
                        n1003 = property on="UUT" class="DigNum (strict)"() -> ("Value"=w2758:u8)  [unwired: 2 in, 2 out]
                        n1004 = call "SetParam.vi"("RS"=TRUE, "error in (no error)"=w2759, "Param to Set in"=w2758, "Visa"=w2756) -> ("error out"=w2739:errorcluster)  [unwired: 7 in]
                        n1005 = control-ref of="Pannel User Message"() -> (w2755:refnum<vi>)
                        n1006 = control-ref of="Stop Burn-in"() -> (w2753:refnum<vi>)
                        n1007 = control-ref of="Stop Button"() -> (w2754:refnum<vi>)
                        n1008 = control-ref of="Motor Speed RPM"() -> (w2752:refnum<vi>)
                        n1009 = property on="VISA Tester" class="VISAName"() -> ("Value"=w2748:refnum<visa-resource-name>)  [unwired: 2 in, 2 out]
                        n1010 = call "TesterOption (SubVI).vi"("2 Options"=w2744, "error in (no error)"=w2739, "On/Off"=FALSE, "Tester Option"=T11."Power", "VISA Refnum in"=w2748) -> ("error out"=w2749:errorcluster, "VISA Refnum out"=w2751:refnum<visa-resource-name>)  [unwired: 5 in]
                        n1011 = call "Write panel message (SubVI).vi"("Stop BurnIn"=w2753, "rpm"=w2752, "PrintTime"=TRUE, "Stop"=w2754, "error in (no error)"=w2749, "Time to wait"=20.0, "Strin"="Restart the UUT\nPlease wait...", "String in"=w2755) -> ("error out"=w2750:errorcluster)  [unwired: 3 in]
                        n1012 = call "TesterOption (SubVI).vi"("2 Options"=w2744, "error in (no error)"=w2750, "On/Off"=FALSE, "Tester Option"=T11."Venable", "VISA Refnum in"=w2751) -> ("error out"=w2738:errorcluster)  [unwired: 5 in, 1 out]
                      }
                    }
                    n1013 = call "Find_Number_LineMARVIN.vi"("Test Paragraph"="2.1", "TableIn"=w2722) -> ("Line number"=w2723:i32)  [unwired: 3 in, 3 out]
                    n1014 = call "SerialMarvinSendGet.vi"("error in (no error)"=w2730, "write buffer"="SN\r\n", "VISA resource name"=w2725) -> ("error out"=w2726:errorcluster, "read buffer"=w2714:string)  [unwired: 7 in]
                    n1015 = call "SerialMarvinSendGet.vi"("error in (no error)"=w2726, "write buffer"="AO[1]\r\n", "VISA resource name"=w2725) -> ("error out"=w2720:errorcluster, "read buffer"=w2721:string)  [unwired: 7 in]
                    n1016 = Fract/Exp String To Number(string=w2721) -> (number=w2716:dbl)  [unwired: 3 in, 1 out]
                    n1017 = In Range and Coerce(upper limit=0.1 ("x"), x=w2716, lower limit=-0.1) -> (In Range?=w2715:bool)  [unwired: 1 out]
                    n1018 = call "PassOrFail (SubVI).vi"("Test#"="2", "index (row)"=w2723, "error in (no error)"=w2720, "Data in"=w2716, "Pass?Fail"=w2715, "Table in"=w2722) -> ("error out"=w2719:errorcluster)  [unwired: 5 in]
                    n1019 = property on="UUT SN Report" class="Str"("Value"=w2714) -> ()  [unwired: 2 in, 2 out]
                    n1020 = Decimal String To Number(string=w2714) -> (number=→"Current SN":i32)  [unwired: 2 in, 1 out]
                  }
                }
              }
            }
          }
          event "Refresh Button": Value Change {
            n1021 = event-data() -> ()  [unwired: 1 in, 6 out]
          }
          event "Settings": Value Change {
            n1022 = event-data() -> ()  [unwired: 1 in, 6 out]
            n1023 = control-ref of="VISA Tester"() -> (w2769:refnum<vi>)
            n1024 = control-ref of="UUT"() -> (w2767:refnum<vi>)
            n1025 = property on="Status" class="Bool (strict)"() -> ("Value"=w2771:bool)  [unwired: 2 in, 2 out]
            n1026 = case shown="True" w2771 {
              tunnel: w2777 -> [_ w2789]
              tunnel: [w2778 w2784] -> w2772
              tunnel: w2770 -> [_ w2783]
              tunnel: w2769 -> [_ w2782]
              tunnel: w2768 -> [_ w2781]
              tunnel: w2767 -> [_ w2780]
              frame False {
                n1027 = call "Display Message to User8"() -> ("error out"=w2778:errorcluster)  [unwired: 10 in, 1 out]
              }
              frame True {
                n1028 = vi-ref "Calibration (SubVI).vi"() -> (w2788:refnum<vi>)
                n1029 = invoke class="VI" method="FP.Open"(reference=w2788, error in=w2789, "Activate"=TRUE ("Activate?"), "State"=T21."Standard") -> (error out=w2785:errorcluster)  [unwired: 1 in, 4 out]
                n1030 = call "Calibration (SubVI).vi"("VISA UUT"=w2783, "error constant"=w2785, "UUT"=w2780, "CAN Cluster in"=w2781, "Visa Tester"=w2782) -> ("error constant 2"=w2784:errorcluster, "AO[1]Meas"=→"Cal":dbl)  [unwired: 5 in]
              }
            }
          }
        }
      }
      frame "Initialize" {
        w2793 = FALSE ("Visible")
        w2794 = FALSE ("Visible")
        w2795 = FALSE ("Visible")
        w2796 = FALSE ("Visible")
        w2808 = refnum<visa-resource-name> "COM1" ("VISA resource name")
        w2798 = FALSE ("Visible")
        w2791 = FALSE ("Serial Status")
        n1031 = property on="ComTestResult" class="Bool (strict)"("Value"=w2796) -> ()  [unwired: 2 in, 2 out]
        n1032 = property on="VenableResult" class="Bool (strict)"("Value"=w2796) -> ()  [unwired: 2 in, 2 out]
        n1033 = property on="VenableDirectionResult" class="Bool (strict)"("Value"=w2796) -> ()  [unwired: 2 in, 2 out]
        n1034 = property on="SpeedResult" class="Bool (strict)"("Value"=w2796) -> ()  [unwired: 2 in, 2 out]
        n1035 = property on="Serial Com" class="Bool"(error in=errorcluster {"status"=FALSE, "code"=0, "source"=""} ("error out"), "Visible"=TRUE) -> (error out=w2810:errorcluster)  [unwired: 1 in, 1 out]
        n1036 = property on="AuxiOFFResult" class="Bool (strict)"("Value"=w2795) -> ()  [unwired: 2 in, 2 out]
        n1037 = property on="AuxiONResult" class="Bool (strict)"("Value"=w2795) -> ()  [unwired: 2 in, 2 out]
        n1038 = property on="VisualInspectionResult" class="Bool (strict)"("Value"=w2795) -> ()  [unwired: 2 in, 2 out]
        n1039 = property on="SensCalResult" class="Bool (strict)"("Value"=w2795) -> ()  [unwired: 2 in, 2 out]
        n1040 = property on="VISA Marvin" class="VISAName"(error in=w2810, "Visible"=w2798, "Value"=w2808) -> (error out=w2799:errorcluster)  [unwired: 1 in, 1 out]
        n1041 = property on="Stop Burn-in" class="Bool (strict)"(error in=w2799, "Visible"=w2798) -> (error out=w2792:errorcluster)  [unwired: 1 in, 1 out]
        n1042 = property on="BurnDC" class="Bool (strict)"("Value"=w2794) -> ()  [unwired: 2 in, 2 out]
        n1043 = property on="BurnTemp" class="Bool (strict)"("Value"=w2794) -> ()  [unwired: 2 in, 2 out]
        n1044 = property on="BurnSpeed" class="Bool (strict)"("Value"=w2794) -> ()  [unwired: 2 in, 2 out]
        n1045 = property on="BurnResult" class="Bool (strict)"("Value"=w2794) -> ()  [unwired: 2 in, 2 out]
        n1046 = property on="Refresh Button" class="Bool (strict)"(error in=w2792, "Value"=FALSE ("Refresh Button")) -> ()  [unwired: 1 in, 2 out]
        n1047 = property on="StopTimeResult" class="Bool (strict)"("Value"=w2793) -> ()  [unwired: 2 in, 2 out]
        n1048 = property on="MotorTempResult" class="Bool (strict)"("Value"=w2793) -> ()  [unwired: 2 in, 2 out]
        n1049 = property on="TempControlResult" class="Bool (strict)"("Value"=w2793) -> ()  [unwired: 2 in, 2 out]
        n1050 = property on="Automation" class="Bool (strict)"("Value"=w2793) -> ()  [unwired: 2 in, 2 out]
        n1051 = flat-sequence {
          tunnel: w2792 -> [w2813]
          tunnel: [w2812] -> w2806
          tunnel: [w2816] -> w2805
          tunnel: w2806 -> [w2816]
          tunnel: [w2828] -> w2804
          tunnel: w2805 -> [w2829]
          tunnel: [w2829] -> w2803
          frame #0 {
            n1052 = control-ref of="This VI"() -> (w2814:refnum<vi>)
            n1053 = invoke class="VI" method="Default Vals.Reinit All"(reference=w2814, error in=w2813) -> (error out=w2812:errorcluster)  [unwired: 1 in, 2 out]
          }
          frame #1 {
            w2819 = u32 4294967295  # AccMask
            w2815 = T4 0 items=["使用Flash参数", "使用界面设置参数"] ("InitFlag")
            w2817 = T6 0 items=["normal operation", "Listen-only mode", "test mode"]  # Mode
            w2818 = T5 3 items=["接收所有类型"=1, "只接收标准帧"=2, "只接收扩展帧"=3] ("Fliter")
            w2823 = u8 10 items=["5k bps"=1, "10k bps"=2, "20k bps"=3, "40k bps"=4, "50k bps"=5, "80k bps"=6, "100k bps"=7, "125k bps"=8, "200k bps"=9, "250k bps"=10, "400k bps"=11, "500k bps"=12, "666k bps"=13, "800k bps"=14, "1000k bps"=15, "33.33k bps"=16, "66.66k bps"=17, "83.33k bps"=18]  # kBaudRate
            w2820 = u32 0  # AccCode
            w2821 = T2 4 items=["USB-CAN"=3, "USB-CAN2"=4] ("DevType")
            w2822 = T7 {"DevType"=3, "DevIndex"=0, "CanIndex"=0, "VCI_INIT_CONFIG"={"AccCode"=0, "AccMask"=0, "InitFlag"=1, "Fliter"=7, "Timing0"=0, "Timing1"=0, "Mode"=0}}  # Config
            # "CANalystII"
            n1054 = call "Demo_GetT0T1.vi"("kBaudRate"=w2823) -> ("Timing0"=w2825:u8, "Timing1"=w2826:u8)
            n1055 = Bundle By Name(cluster=w2822, "DevType"=w2821, "CanIndex"="Channel 2", "VCI_INIT_CONFIG.AccCode"=w2820, "VCI_INIT_CONFIG.AccMask"=w2819, "VCI_INIT_CONFIG.InitFlag"=w2815, "VCI_INIT_CONFIG.Fliter"=w2818, "VCI_INIT_CONFIG.Timing0"=w2825, "VCI_INIT_CONFIG.Timing1"=w2826, "VCI_INIT_CONFIG.Mode"=w2817) -> (→"Config_CANAT":T7)
          }
          frame #2 {
            w2830 = u16 284 items=["1M"=20, "500K"=28, "250K"=284, "125K"=796, "100K"=17199, "50K"=18223, "20K"=21295, "10K"=26415, "5K"=32639] ("baud in")
            n1056 = control-ref of="Config_CANAT"() -> (w2828:refnum<vi>)
            n1057 = call "InitCAN_ATII.vi"("Config"=w2828) -> ("Sts"=→"CAN Status":bool)
            n1058 = call "ChangeCANBaud.vi"("baud in"=w2830, "reference"=w2828) -> ()
          }
        }
        "Status" <- w2791
        "Test Failed" <- w2791
      }
    }
  }
  n1059 = property on="Settings" class="Bool (strict)"("Visible"=w4) -> ()  [unwired: 2 in, 2 out]
  n1060 = property on="Cal" class="DigNum (strict)"("Visible"=w4) -> ()  [unwired: 2 in, 2 out]
  n1061 = disable-structure shown="Disabled" {
    frame Disabled {
      w2832 = T19."Disabled and Grayed Out" ("Disabled")
      w2833 = FALSE ("Start")
      n1062 = property on="VISA Tester" class="VISAName" props=["Value"]() -> ()  [unwired: 2 in, 3 out]
      n1063 = property on="Current SN" class="DigNum (strict)" props=["Value"]() -> ()  [unwired: 2 in, 3 out]
      n1064 = property on="UUT" class="DigNum (strict)" props=["Value"]() -> ()  [unwired: 2 in, 3 out]
      n1065 = property on="Status" class="Bool (strict)" props=["Value"]() -> ()  [unwired: 2 in, 3 out]
      n1066 = property on="UUT SoftwareVer" class="Str" props=["Value"]() -> ()  [unwired: 2 in, 3 out]
      n1067 = property on="Next SN" class="DigNum (strict)" props=["Value"]() -> ()  [unwired: 3 in, 2 out]
      n1068 = property on="Start" class="Bool (strict)"("Value"=w2833, "DisabledEnum"=w2832) -> ()  [unwired: 2 in, 2 out]
      n1069 = property on="Report" class="Bool (strict)"("Value"=w2833, "DisabledEnum"=w2832) -> ()  [unwired: 2 in, 2 out]
    }
    frame Enabled {
    }
  }
  n1070 = disable-structure shown="Disabled" {
    frame Disabled {
      (unwired) 0.02003173828125 ("x")
      n1071 = control-ref of="Stop Burn-in"() -> ()  [unwired: 1 out]
      n1072 = control-ref of="Stop Button"() -> ()  [unwired: 1 out]
      n1073 = control-ref of="Motor Speed RPM"() -> ()  [unwired: 1 out]
      n1074 = control-ref of="Config_CANAT"() -> ()  [unwired: 1 out]
      n1075 = control-ref of="UUT"() -> ()  [unwired: 1 out]
      n1076 = call "GetADCTester (SubVI).vi"() -> ()  [unwired: 9 in, 3 out]
      n1077 = call "CANSendMotorSpeed.vi"() -> ()  [unwired: 11 in, 1 out]
      n1078 = control-ref of="Config_CANAT"() -> ()  [unwired: 1 out]
      n1079 = call "Find_Number_LineMARVIN.vi"() -> ()  [unwired: 5 in, 4 out]
      n1080 = property on="UUT" class="DigNum (strict)" props=["Value"]() -> ()  [unwired: 2 in, 3 out]
      n1081 = control-ref of="UUT"() -> ()  [unwired: 1 out]
      n1082 = call "DegToDAC (SubVI).vi"() -> ()  [unwired: 10 in, 2 out]
      n1083 = call "Write panel message (SubVI).vi"() -> ()  [unwired: 11 in, 1 out]
      n1084 = property on="VISA Tester" class="VISAName" props=["Value"]() -> ()  [unwired: 2 in, 3 out]
      n1085 = control-ref of="ATR"() -> ()  [unwired: 1 out]
      n1086 = call "TesterOption (SubVI).vi"() -> ()  [unwired: 10 in, 2 out]
      n1087 = call "TesterOption (SubVI).vi"() -> ()  [unwired: 10 in, 2 out]
      n1088 = call "PassOrFail (SubVI).vi"() -> ()  [unwired: 11 in, 1 out]
    }
    frame Enabled {
    }
  }
  n1089 = disable-structure shown="Disabled" {
    frame Disabled {
      n1090 = flat-sequence {
        frame #0 {
          n1091 = call "CANSendMotorSpeed.vi"("Remote"=TRUE, "Motor Speed RPM"=u16 0) -> ("error out"=w2835:errorcluster, "UUT"=w2838:refnum<vi>)  [unwired: 8 in]
          n1092 = property on="VISA Tester" class="VISAName"() -> ("Value"=w2834:refnum<visa-resource-name>)  [unwired: 2 in, 2 out]
          n1093 = call "TesterOption (SubVI).vi"("error in (no error)"=w2835, "On/Off"=FALSE, "Tester Option"=T11."Power", "VISA Refnum in"=w2834) -> ()  [unwired: 6 in, 2 out]
        }
      }
    }
    frame Enabled {
    }
  }
  "Pannel User Message" <- w2
